vi "MAIN.vi"() -> ()   [LabVIEW 2015]
doc: "Use this template to create an application that executes repeatedly until you click the Stop button. This template polls the state of the Stop button and does not use events. Use the Top-Level Application template (not available in the Base package) to create a single-loop application with event handling."
uses:
  Lib_Bled112 toolkit/type_def/connection_status_bundle.ctl
  Lib_Bled112 toolkit/type_def/address_type.ctl
  Lib_Bled112 toolkit/type_def/message_type.ctl
  Lib_Bled112 toolkit/type_def/message_class.ctl
  <vilib>/Utility/miscctls.llb/LVPointTypeDef.ctl
  SUB_Load and Save Controls.llb/RWC_Actions.ctl
  <vilib>/Utility/miscctls.llb/LVRowAndColumnTypeDef.ctl
  <vilib>/event_ctls.llb/eventvkey.ctl
  <vilib>/Utility/sysdir.llb/System Directory Type.ctl
  <vilib>/addons/_office/_exclsub.llb/font.ctl
  <vilib>/Analysis/baseanly.llb/Mean (DBL).vi
  <vilib>/Utility/config.llb/Read Key (String).vi
  <vilib>/Utility/config.llb/Read Key (I32).vi
  Lib_Bled112 toolkit/ble_functions/ble_write_by_handle_uint8array.vi
  <vilib>/addons/_office/excel.llb/Excel Easy Table (str).vi
  <vilib>/Utility/config.llb/Write Key (String).vi
  <vilib>/Utility/config.llb/Write Key (U32).vi
  <vilib>/Utility/NIReport.llb/NI_report.lvclass
  <vilib>/Utility/config.llb/NI_LVConfig.lvlib
  <vilib>/Analysis/NI_AALBase.lvlib
  <vilib>/addons/_office/NI_ReportGenerationToolkit.lvlib
  <vilib>/Utility/NIReport.llb/Excel/NI_Excel.lvclass
panel:
  out "Packet No.":u16
  out "Rx-debug":bool
  out "FTS table index":i32
  out "ms timer 5":u32=38996702
  out "ms timer 4":u32=27271323
  out "ms timer 3":u32=38996702
  in  "Update(ms)":u16=100
  out "ms timer 2":u32=38996702
  out "Rx-ROM":bool
  out "BLE Packet (mon)":u8[](array[numeric])=[119, 32, 48, 163, 32, 0, 45, 32, 53, 143, 30, 162, 83, 32, 86, 151, 32, 67, 185, 208, 89, 94, 66, 75, 91, 193, 107, 187, 98, 158, 102, 165, 208]
  out "Timer-ble log":u32=38996556
  out "log data1":bool
  out "log ble buf":string
  out "Packet Detect":bool
  out "Disconnected":bool
  out "Rx buf 1":string
  out "Rx Cnt":i32
  out "Rx Packet Structure":T1={"Message Type (Response)"=128, "Payload length"=25, "Command Class (System)"=4, "Message ID"=5, "Connection handle"=0, "Attribute handle"=11, "Attribute type"=1, "Attribute value (data)"=[119, 32, 48, 110, 31, 255, 217, 32, 53, 83, 30, 161, 69, 32, 87, 130, 32, 68, 21, 209]} {"Attribute type" format="%02x" items=["read", "notify", "indicate", "read_by_type", "read_blob", "indicate_rsp_req"]; "Attribute value (data)" format="%02x"; "Attribute handle" format="%04x"; "Connection handle" format="%02x"; "Message ID" format="%02x"; "Message Type (Response)" format="%02x" items=["Command / Response"=0, "Event"=128]; "Command Class (System)" format="%02x" items=["System", "Persistent Store", "Attribute database", "Connection", "Attribute client", "Security Manager", "Generic Access Profile", "Hardware"]}
  out "Device Name":string="GEN4_PERSONA_3rd_jun"
  out "Connection Status":T4={"MAC Address"="F8:B8:54:EF:76:8D", "cnx handle"=0, "cnx flags"=5, "Address Type"=1, "Connection Interval (ms)"=8, "Timeout(ms)"=1000, "Latency"=0, "bonding handle"=255} {"Address Type" items=["Public", "Random"]}
  in  "Log no":string="1" caption="No."
  out "FTS OP status":T6="시험 시작"
  out "Test profile":string[][](array[string])=[["Load(1)-0lb", "0", "1000", "0", "0"], ["Init(1)-70lb", "70", "1000", "0", "0"], ["Init(2)-140lb", "140", "1000", "0", "0"], ["Init(1)-70lb", "70", "1000", "0", "0"], ["Init(2)-140lb", "140", "1000", "0", "0"], ["Load(1)-0lb", "0", "10000", "1", "1"], ["Load(2)-10lb", "10", "3000", "0", "1"], ["Load(3)-20lb", "20", "3000", "0", "1"], ["Load(4)-40lb", "40", "3000", "0", "1"], ["Load(5)-60lb", "60", "3000", "0", "1"], ["Load(6)-80lb", "80", "3000", "0", "1"]]
  out "log refnum":refnum<file> caption="참조 번호 복제"
  out "ms timer":u32=38996556
  out "Logging No.":u32
  in  "Data Logging":bool caption="Data Logging (Desktop folder)"
  out "RxD":string
  out "Graph timer 2":u32=38996702
  out "창크게":bool
  out "Comm err cnt 1":i32
  out "Graph timer 1":u32=38996702
  in  "Setting load":bool=TRUE
  out "ACT-Comm":bool
  in  "Comm con 1":bool
  in  "Port close 1":bool
  in  "Port open 1":bool
  in  "탭-Top":T7(tab)
  in  "CDC Graph plot":bool
  in  "Offset Souce":enum32{"Normal", "Raw"}(radio)
  out "CDC Offet":T8 caption="CDC Offset data" {"Right Wing-C, C6/C0" format="%#.9f"; "Right Wing-B, C5/C0" format="%#.9f"; "Right Wing-A, C4/C0" format="%#.9f"; "Left Wing-C, C3/C0" format="%#.9f"; "Left Wing-B, C2/C0" format="%#.9f"; "Left Wing-A, C1/C0" format="%#.9f"}
  in  "Export graph 1":bool
  in  "Clear graph 1":bool
  out "CDC(PCAP02) Graph":waveform(dbl)[](graph)=[{"t0"=timestamp(3566271640.952271 s since 1904-01-01), "dt"=0.10400000000000001, "Y"=[22878.0]}, {"t0"=timestamp(3566271640.952271 s since 1904-01-01), "dt"=0.10400000000000001, "Y"=[16971.0]}, {"t0"=timestamp(3566271640.952271 s since 1904-01-01), "dt"=0.10400000000000001, "Y"=[23489.0]}, {"t0"=timestamp(3566271640.952271 s since 1904-01-01), "dt"=0.10400000000000001, "Y"=[27579.0]}, {"t0"=timestamp(3566271640.952271 s since 1904-01-01), "dt"=0.10400000000000001, "Y"=[25246.0]}, {"t0"=timestamp(3566271640.952271 s since 1904-01-01), "dt"=0.10400000000000001, "Y"=[26279.0]}, {"t0"=timestamp(3566271640.952271 s since 1904-01-01), "dt"=0.10400000000000001, "Y"=[1.0058650970458984]}, {"t0"=timestamp(3566271640.952271 s since 1904-01-01), "dt"=0.10400000000000001, "Y"=[0.9999599456787109]}, {"t0"=timestamp(3566271640.952271 s since 1904-01-01), "dt"=0.10400000000000001, "Y"=[1.0064787864685059]}, {"t0"=timestamp(3566271640.952271 s since 1904-01-01), "dt"=0.10400000000000001, "Y"=[0.9571785926818848]}, {"t0"=timestamp(3566271640.952271 s since 1904-01-01), "dt"=0.10400000000000001, "Y"=[1.0106620788574219]}, {"t0"=timestamp(3566271640.952271 s since 1904-01-01), "dt"=0.10400000000000001, "Y"=[1.0083107948303223]}]
  out "CDC data":T8 caption="CDC Monitoring data" {"Right Wing-C, C6/C0" format="%#.9f"; "Right Wing-B, C5/C0" format="%#.9f"; "Right Wing-A, C4/C0" format="%#.9f"; "Left Wing-C, C3/C0" format="%#.9f"; "Left Wing-B, C2/C0" format="%#.9f"; "Left Wing-A, C1/C0" format="%#.9f"}
  in  "Offset 1":bool
  out "IMU Offet":T9 caption="IMU Offset data" {"Accelerometer Z" format="%#.9f"; "Accelerometer Y" format="%#.9f"; "Accelerometer X" format="%#.9f"; "Gyroscope Z" format="%#.9f"; "Gyroscope Y" format="%#.9f"; "Gyroscope X" format="%#.9f"}
  out "IMU Graph":waveform(dbl)[](graph)=[{"t0"=timestamp(3566271136.852438 s since 1904-01-01), "dt"=0.108, "Y"=[-1.063125]}, {"t0"=timestamp(3566271136.852438 s since 1904-01-01), "dt"=0.108, "Y"=[0.118125]}, {"t0"=timestamp(3566271136.852438 s since 1904-01-01), "dt"=0.108, "Y"=[0.20125]}, {"t0"=timestamp(3566271136.852438 s since 1904-01-01), "dt"=0.108, "Y"=[-0.014029999999999999]}, {"t0"=timestamp(3566271136.852438 s since 1904-01-01), "dt"=0.108, "Y"=[-0.00366]}, {"t0"=timestamp(3566271136.852438 s since 1904-01-01), "dt"=0.108, "Y"=[1.0149789999999999]}]
  in  "Clear graph 2":bool
  in  "Export graph2":bool
  out "IMU data":T9 caption="IMU Monitoring data" {"Accelerometer Z" format="%#.9f"; "Accelerometer Y" format="%#.9f"; "Accelerometer X" format="%#.9f"; "Gyroscope Z" format="%#.9f"; "Gyroscope Y" format="%#.9f"; "Gyroscope X" format="%#.9f"}
  in  "Offset 2":bool
  out "Full ROM data":bool
  in  "Flash Map":enum32{"Data Map", "Raw Data"}(tab)
  out "ROM Table":string[][](table)=[["Device ID", "-", "-"], ["Main Chip", "-", "-"], ["YEAR", "-", "-"], ["Month", "-", "-"], ["Day", "-", "-"], ["Device Type", "-", "-"], ["Manufacturer ID", "-", "-"], ["Cal_Acc. X", "-", "-"], ["Cal_Acc. Y", "-", "-"], ["Cal_Acc. Z", "-", "-"], ["Cal_Gy. X", "-", "-"], ["Cal_Gy. Y", "-", "-"], ["Cal_Gy. Z", "-", "-"], ["Cal_Vol H", "-", "-"], ["Cal_Vol L", "-", "-"], ["Cal_CDC Off 1", "-", "-"], ["Cal_CDC Off 2", "-", "-"], ["Cal_CDC Off 3", "-", "-"], ["Cal_CDC Off 4", "-", "-"], ["Cal_CDC Off 5", "-", "-"], ["Cal_CDC Off 6", "-", "-"], ["Cal_CDC Gain A", "-", "-"], ["Cal_CDC Gain B", "-", "-"]]
  out "Rx ROM-log":string
  out "ROM Data":T10(array[cluster]) {"Index" format="%02x"; "ROM Data" format="%02x"}
  in  "Mode":bool=TRUE
  in  "Debugging Mode":bool
  in  "Data Log":string
  out "Data_mon(h)":string
  in  "Data(h)":string="\u0001"
  in  "Send":bool
  in  "Handle":u8=16 format="%02x"
  in  "Grahp Clear":bool
  out "BLE RSSI buf":i16(graph)=-63
  out "BLE RSSI Graph":dbl(graph)=-65.56666666666666
  out "BLE RSSI (dBm)":dbl format="%.1f"
  out "BLE AVG-Interval Graph":dbl(graph)=11.355
  out "BLE Interval Time(ms)":dbl format="%.1f"
  out "BLE Interval buf":u32(graph)=11
  out "Bat(raw)":u16 format="%04x"
  in  "Cal/Test select":bool=TRUE
  in  "Head Up":bool
  in  "Load(lb)":dbl=10.0 min=0.0 max=150.0 step=0.1
  in  "Test name":string="Noname"
  out "Load vs CDC Graph":cluster{dbl[], dbl[]}[](graph)
  out "Mark10 Gauge (lb)":dbl format="%.2f"
  out "Test Status":string
  out "Test Data table":string[][](table)=[["-", "-", "-", "-", "-", "-", "-"], ["-", "-", "-", "-", "-", "-", "-"], ["-", "-", "-", "-", "-", "-", "-"], ["-", "-", "-", "-", "-", "-", "-"], ["-", "-", "-", "-", "-", "-", "-"], ["-", "-", "-", "-", "-", "-", "-"], ["-", "-", "-", "-", "-", "-", "-"], ["-", "-", "-", "-", "-", "-", "-"], ["-", "-", "-", "-", "-", "-", "-"]]
  in  "Test Start":bool
  in  "Port-FTS":refnum<visa-resource-name>="COM6" caption="FTS \nCOM port"
  in  "FTS Testing":bool
  out "FTS comm.":bool
  in  "Force Set":bool
  out "Rx-mon":bool
  out "Comm con status 1":bool caption="Status"
  out "*Board ID1":string="None...." caption="S/N"
  in  "Port-set 1":refnum<visa-resource-name>="COM8" caption="COM port"
  out "Port-act 1":refnum<visa-resource-name>="COM8"
  in  "stop":bool=TRUE
  out "Data trx(led)":bool
  in  "Setting load(led)":bool
  out "status string":string="Ready (available after the communication connection)"
  # "GEN4 PP3 - GUI Program"
  # "Ver. 170112A"
  # "Comm. Connection"
  # "(Connection)"
  # "Serial port"
  # "Gyroscope X"
  # "Gyroscope Y"
  # "Gyro. (dps)"
  # "Gyroscope Z"
  # "Accelerometer X"
  # "Accelerometer Y"
  # "Acc. (g)"
  # "Accelerometer Z"
  # "* Debugging mode\nHandler : 0x000B\nWrite : 0x4A 0x73 0x50"
  # "Reserved"
  # "ESM301: 115200bps\nMARK10: 9600bps"
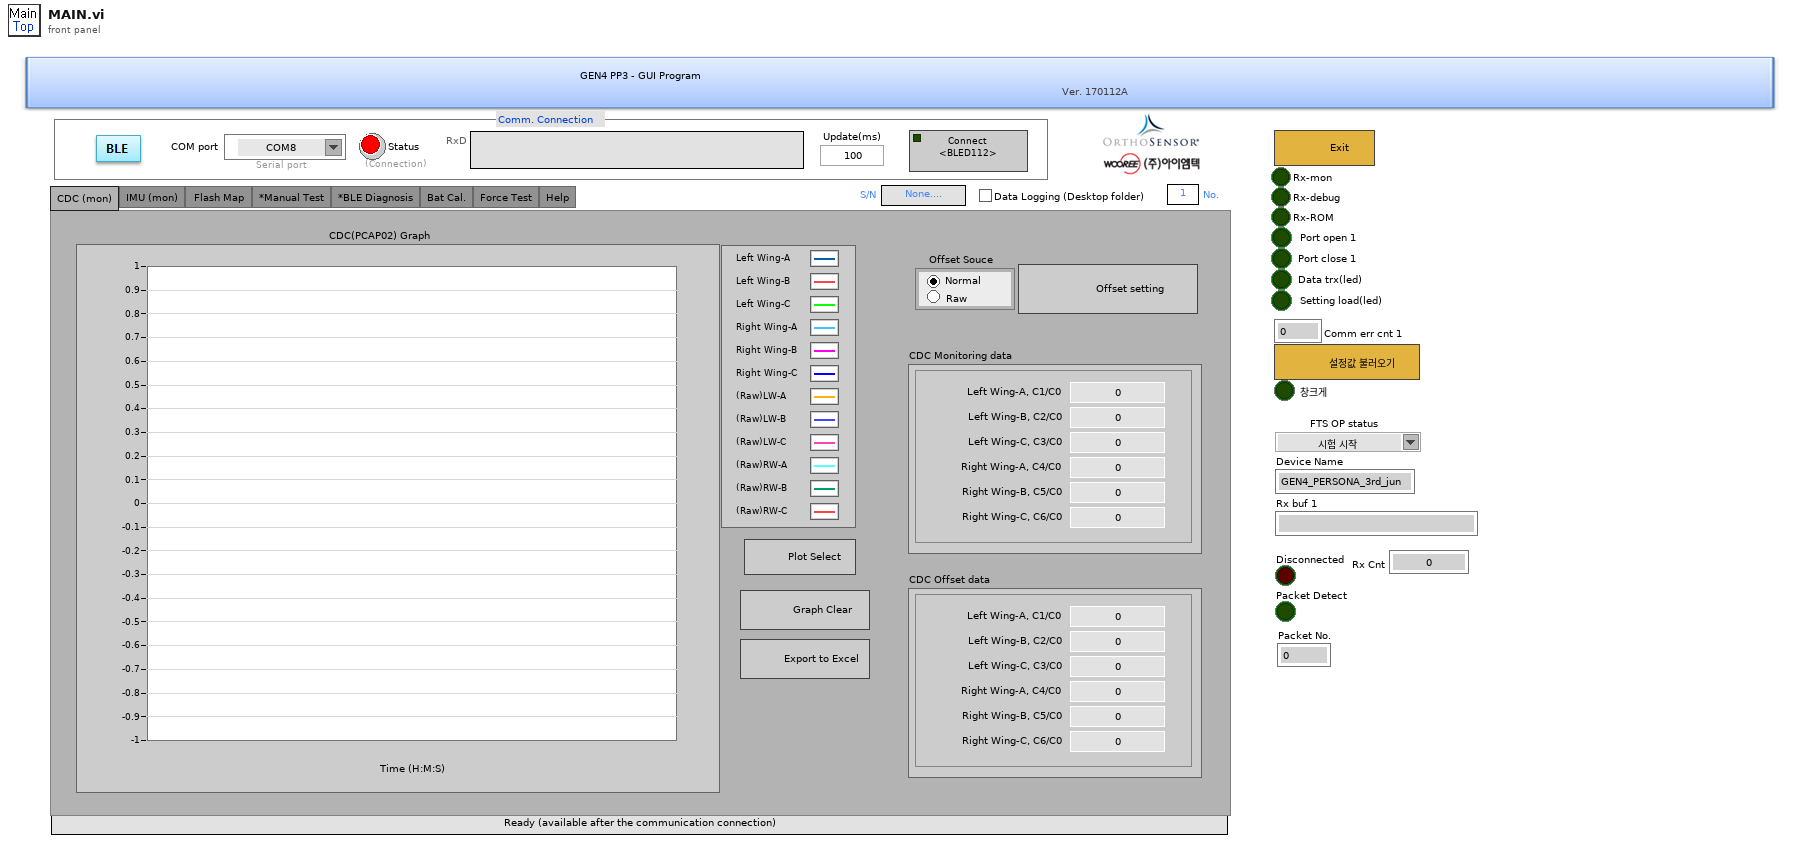
[diagram p1: front panel]
types:
  T1 = typedef "컨트롤-BLED Rx (EVENT-Attribute Client).ctl" = cluster{"Message Type (Response)":T2, "Payload length":u8, "Command Class (System)":T3, "Message ID":u8, "Connection handle":u8, "Attribute handle":u16, "Attribute type":T3, "Attribute value (data)":u8[]}
  T2 = typedef "message_type.ctl" = u8
  T3 = typedef "message_class.ctl" = u8
  T4 = typedef "connection_status_bundle.ctl" = cluster{"MAC Address":string, "cnx handle":u8, "cnx flags":u8, "Address Type":T5, "Connection Interval (ms)":u16, "Timeout(ms)":u16, "Latency":u16, "bonding handle":u8}
  T5 = typedef "address_type.ctl" = u8
  T6 = typedef "컨트롤-동작시험상태 FTS.ctl" = string
  T7 = enum32{"CDC (mon)", "IMU (mon)", "Flash Map ", "*Manual Test", "*BLE Diagnosis", "Bat Cal.", "Force Test", "Help"}
  T8 = typedef "컨트롤-CDC data.ctl" = cluster{"Left Wing-A, C1/C0":dbl, "Left Wing-B, C2/C0":dbl, "Left Wing-C, C3/C0":dbl, "Right Wing-A, C4/C0":dbl, "Right Wing-B, C5/C0":dbl, "Right Wing-C, C6/C0":dbl}
  T9 = typedef "컨트롤-IMU data.ctl" = cluster{"Gyroscope X":dbl, "Gyroscope Y":dbl, "Gyroscope Z":dbl, "Accelerometer X":dbl, "Accelerometer Y":dbl, "Accelerometer Z":dbl}
  T10 = cluster{"RxOK":bool, "ROM Data":u8[], "Index":u8}[]
  T11 = typedef "RWC_Actions.ctl" = enum16{"Read", "Write", "Read and Create"}
  T12 = enum16{"Always On", "Always Off", "Off While Running"}
  T13 = typedef "LVPointTypeDef.ctl" = cluster{"Horizontal":i16, "Vertical":i16}
  T14 = cluster{"RxOK":bool, "ROM Data":u8[], "Index":u8}
  T15 = typedef "LVRowAndColumnTypeDef.ctl" = cluster{"Row":i32, "Column":i32}
  T16 = enum16{"Standard Report", "HTML", "Word", "Excel"}
  T17 = enum16{"maximized", "minimized", "normal", "no change"}
  T18 = typedef "NI_ReportGenerationToolkit.lvlib/font.ctl" = cluster{"font name":string, "font size":dbl, "bold":u16, "italic":u16, "underline":u16, "strike through":u16, "font color":u32}
  T19 = cluster{"on/off":bool, "weight":i32, "color":u32}
  T20 = typedef "컨트롤-동작상태 FTS.ctl" = string
  T21 = typedef "eventvkey.ctl" = enum16{"ASCII", "Enter", "Return", "Shift", "Ctrl", "Alt", "Cmd", "Opt", "Caps", "NumLock", "Clear", "Break", "Up", "Down", "Left", "Right", "Insert", "Delete", "Home", "End", "PageUp", "PageDown", "Escape", "Help", "Pause", "ScrollLock", "F1", "F2", "F3", "F4", "F5", "F6", "F7", "F8", "F9", "F10", "F11", "F12", "F13", "F14", "F15", "F16", "F17", "F18", "F19", "F20", "F21", "F22", "F23", "F24", "Play", "VolumeUp", "VolumeDown", "Mute", "Two Byte Char"}
  T22 = enum16{"open", "replace", "create", "open or create", "replace or create", "replace or create with confirmation"}
  T23 = typedef "NI_LVConfig.lvlib/Config Data RefNum.ctl" = refnum<k1>
  T24 = typedef "System Directory Type.ctl" = i32
  T25 = typedef "LVRectTypeDef.ctl" = cluster{"Left":i16, "Top":i16, "Right":i16, "Bottom":i16}
  T26 = typedef "컨트롤-BLED Rx (EVENT-Connection status).ctl" = cluster{"Message Type (Response)":T2, "Payload length":u8, "Command Class (System)":T3, "Message ID":u8, "Connection handle":u8, "flags":u8, "Bluetooth address":u8[], "address type":T3, "conn_interval(ms)":dbl, "timeout(ms)":dbl, "latency":u16, "bonding(0xFF)":u8}
  T27 = typedef "컨트롤-BLED Rx (Get RSSI).ctl" = cluster{"Message Type (Response)":T2, "Payload length":u8, "Message class":u8, "Message ID":u8, "connection":u8, "rssi":i16}
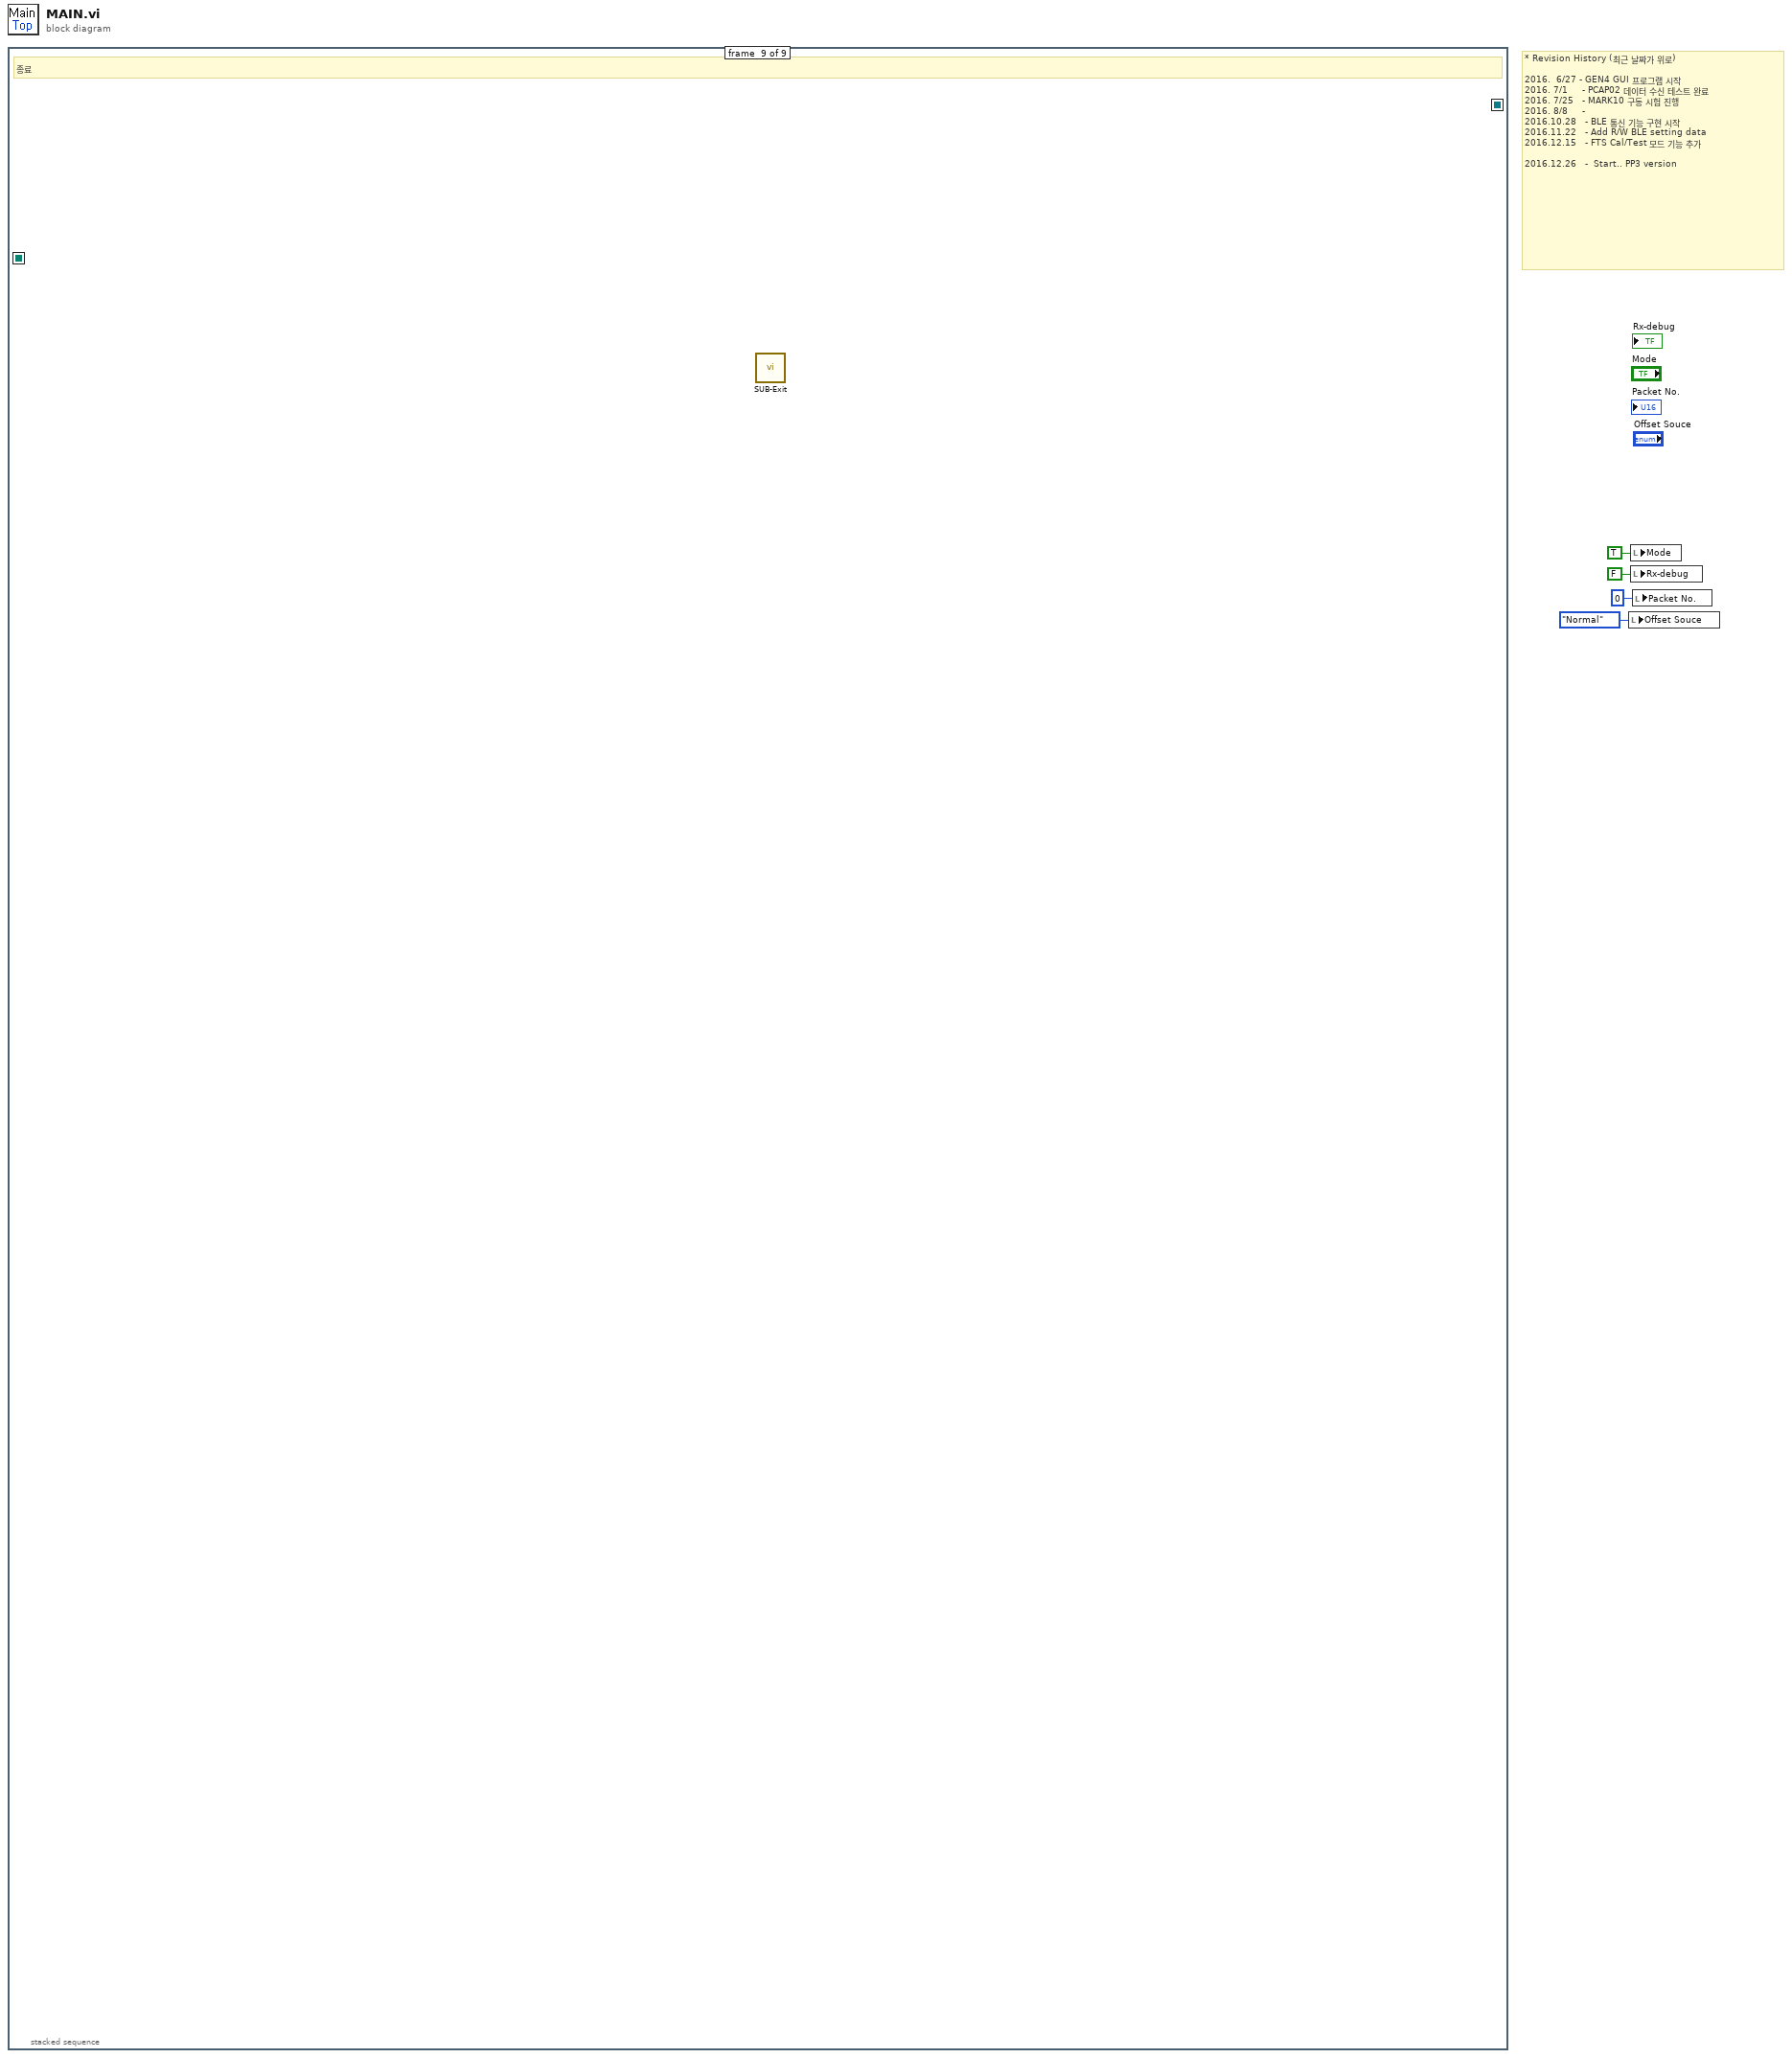
[diagram p0: block diagram]
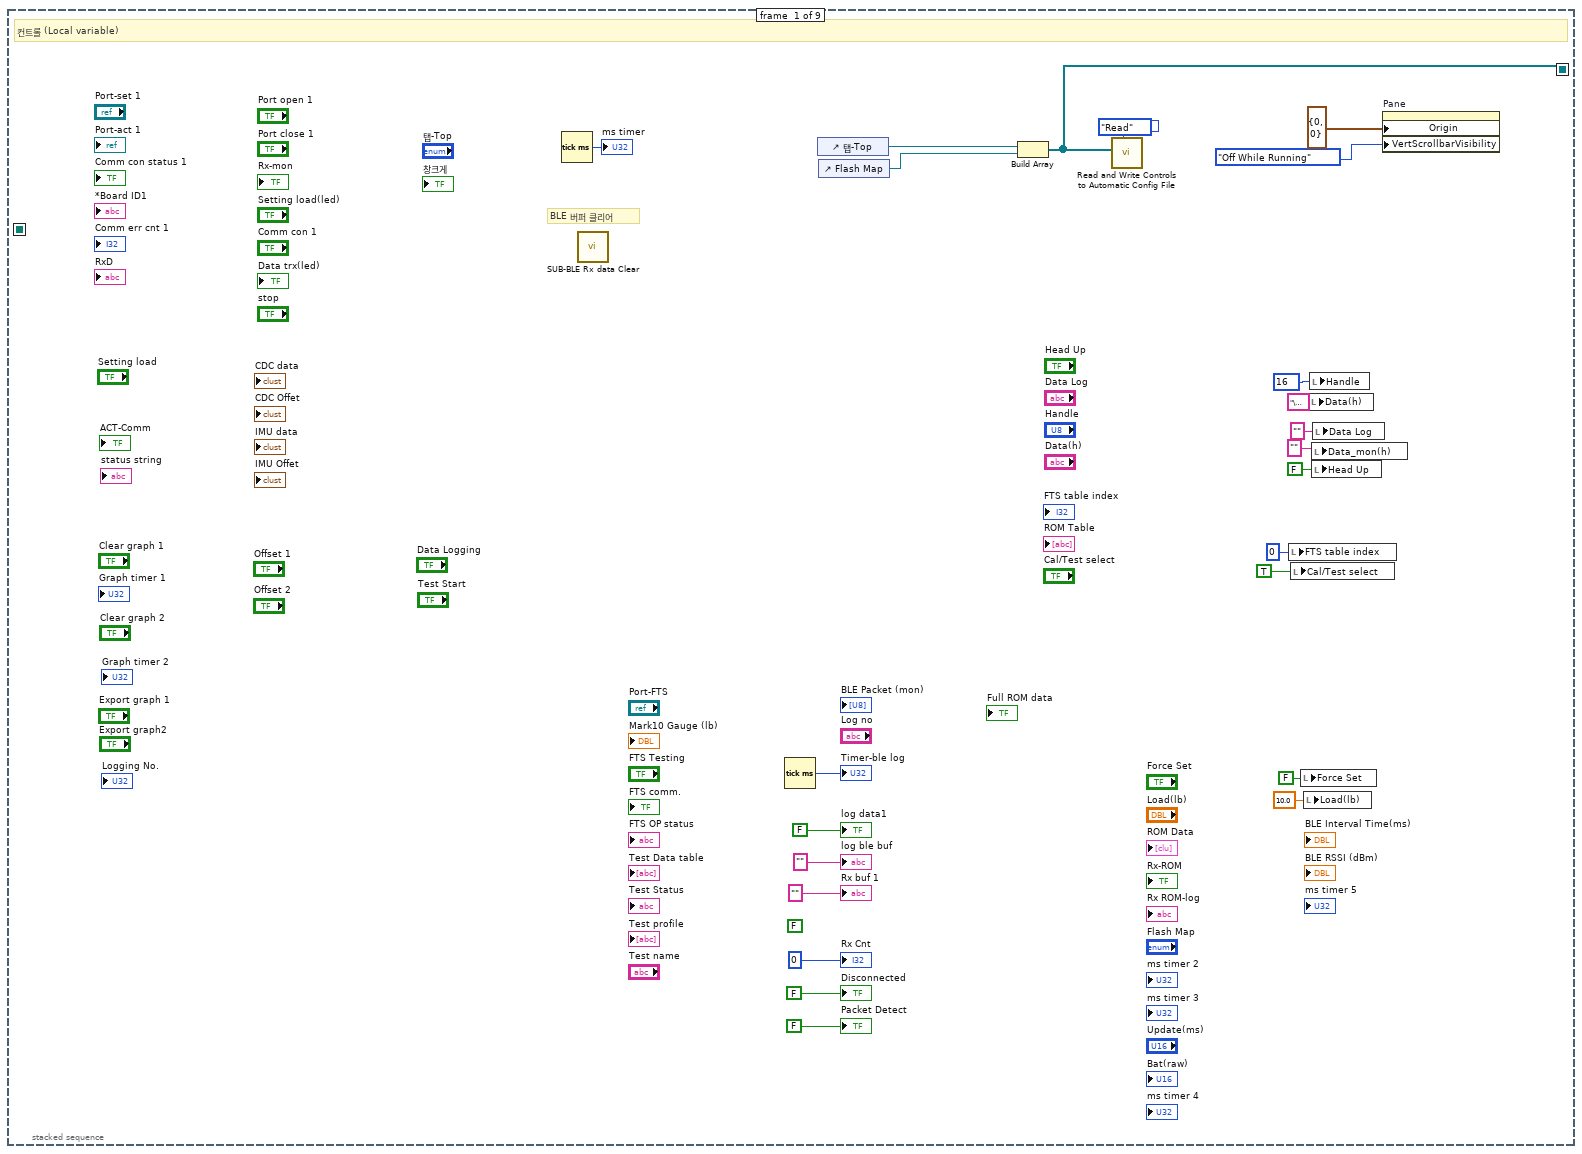
[diagram p2: hidden frame]
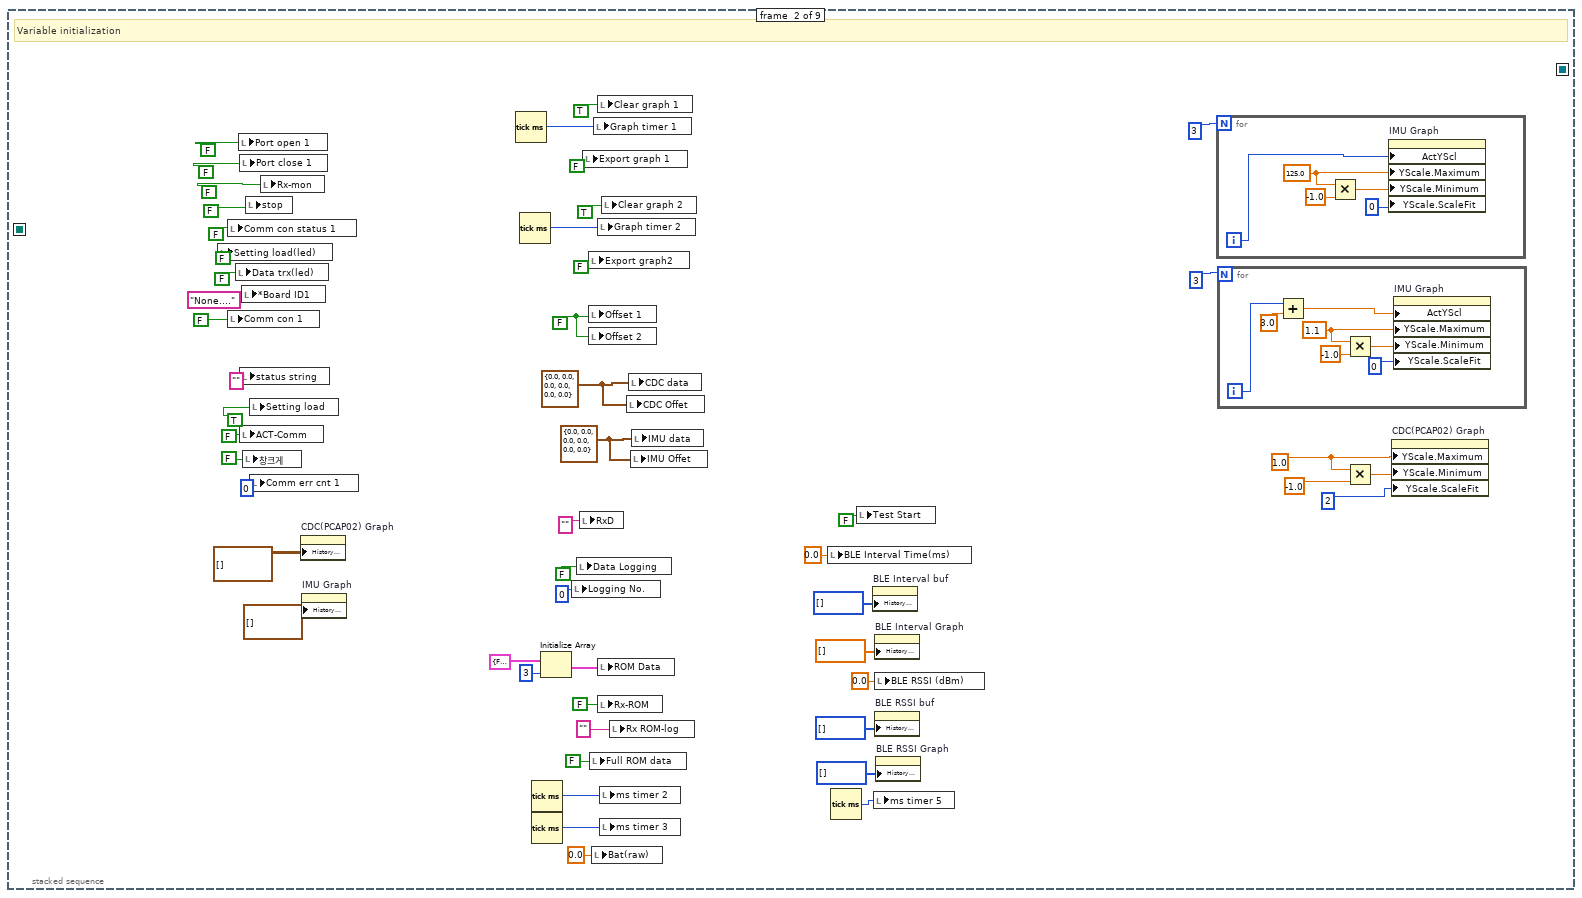
[diagram p3: hidden frame]
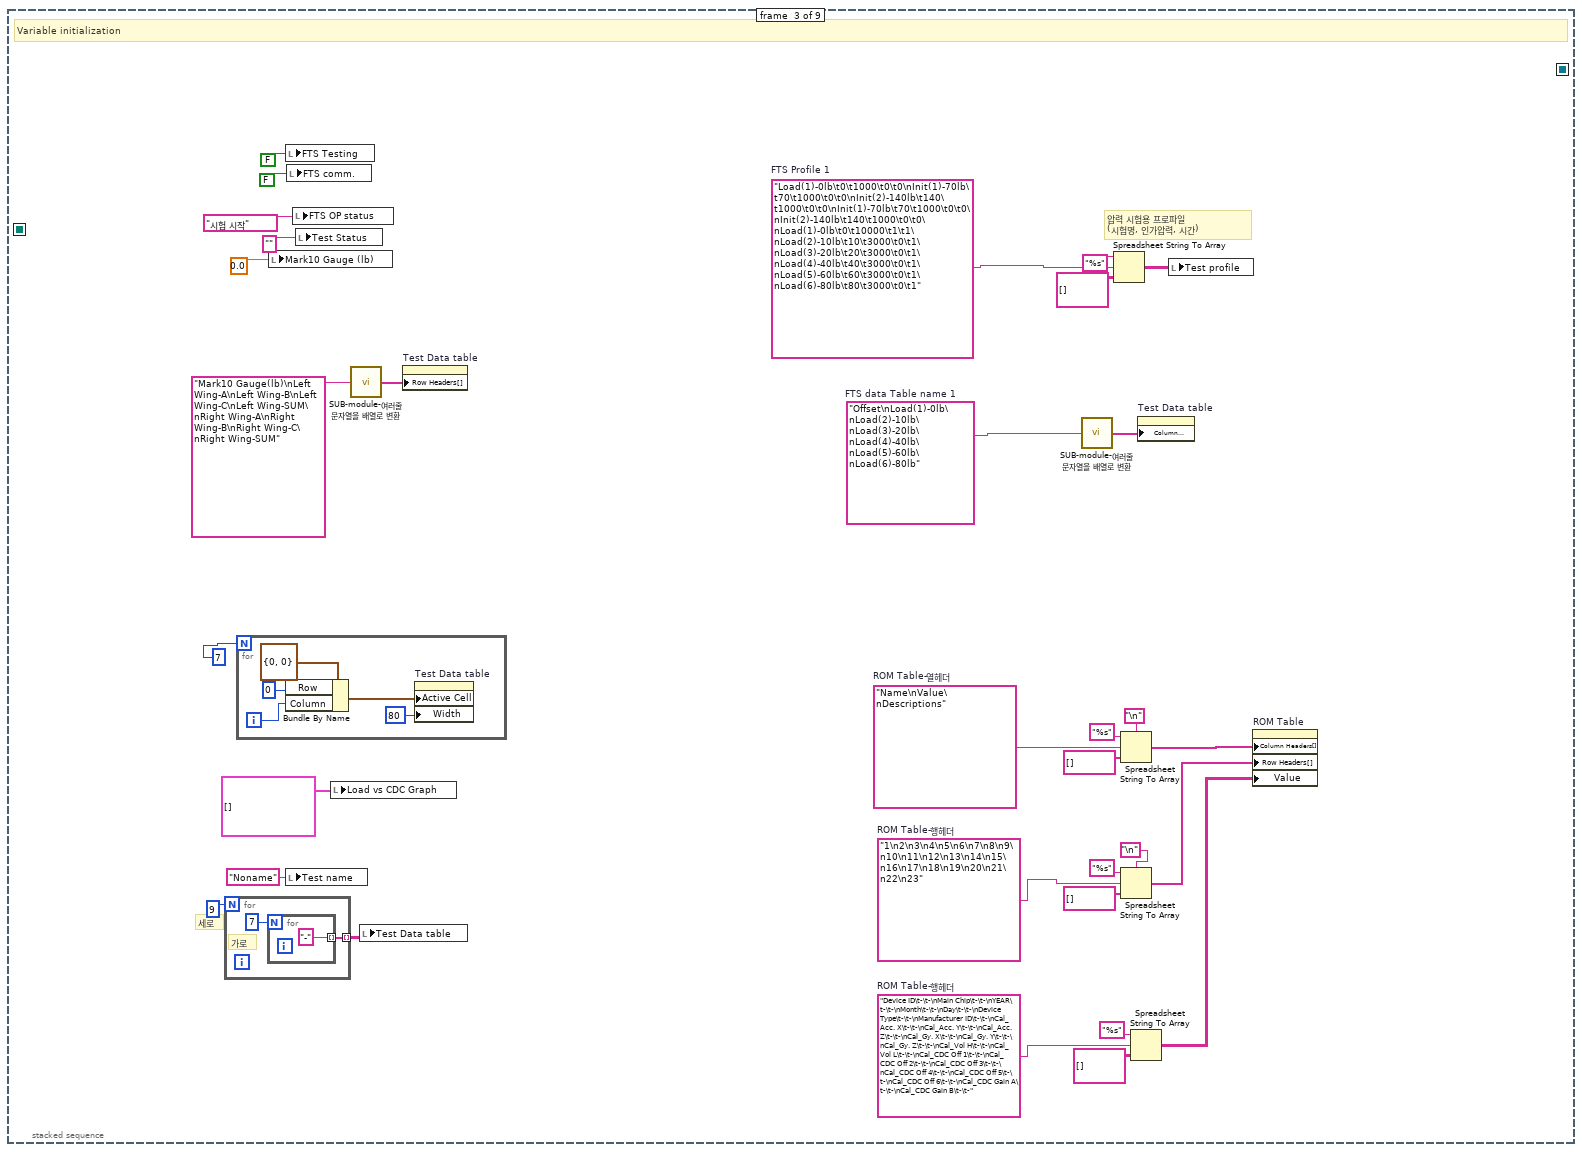
[diagram p4: hidden frame]
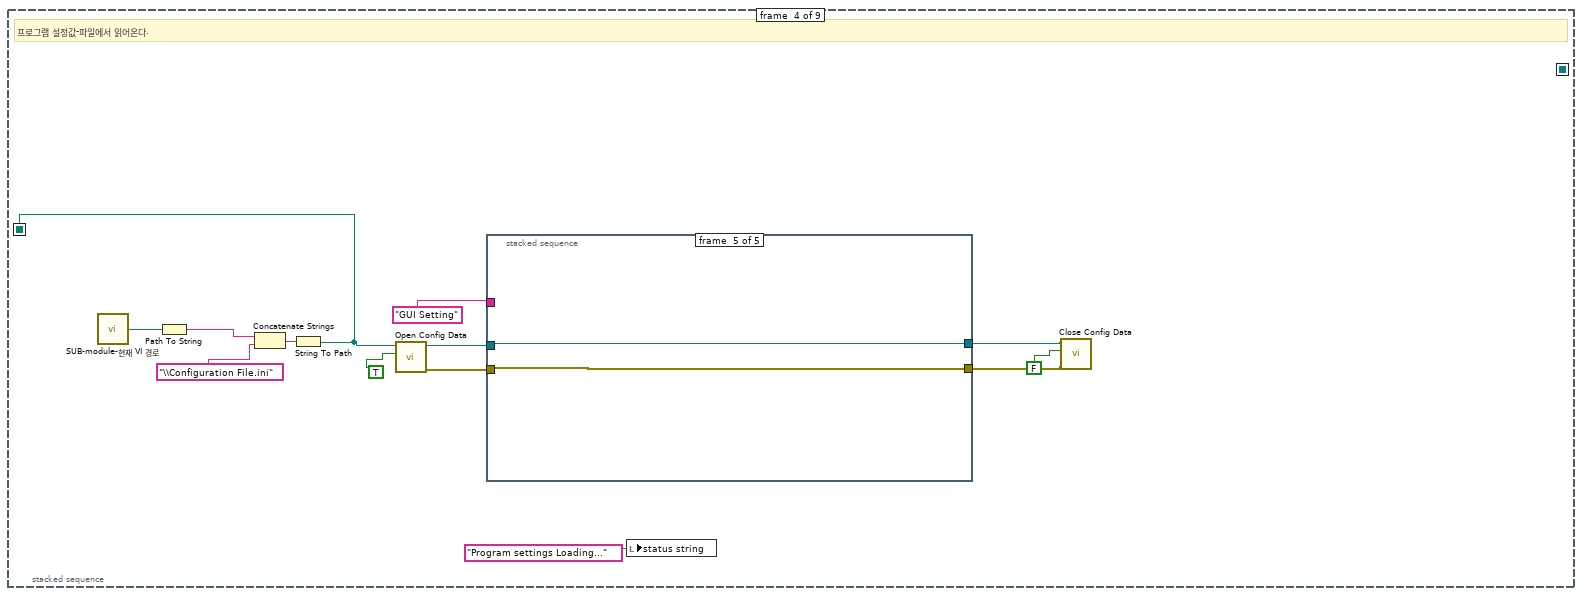
[diagram p5: hidden frame]
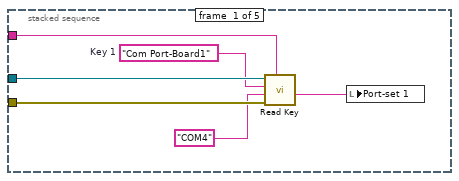
[diagram p6: hidden frame]
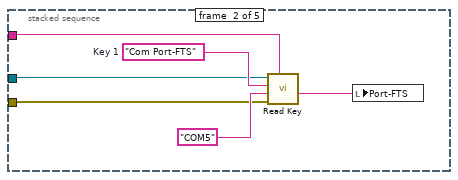
[diagram p7: hidden frame]
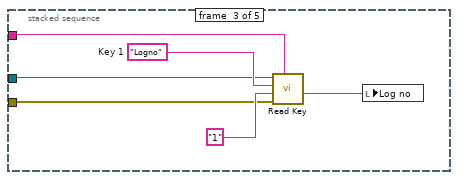
[diagram p8: hidden frame]
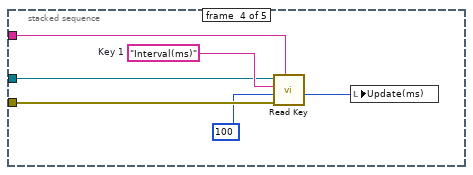
[diagram p9: hidden frame]
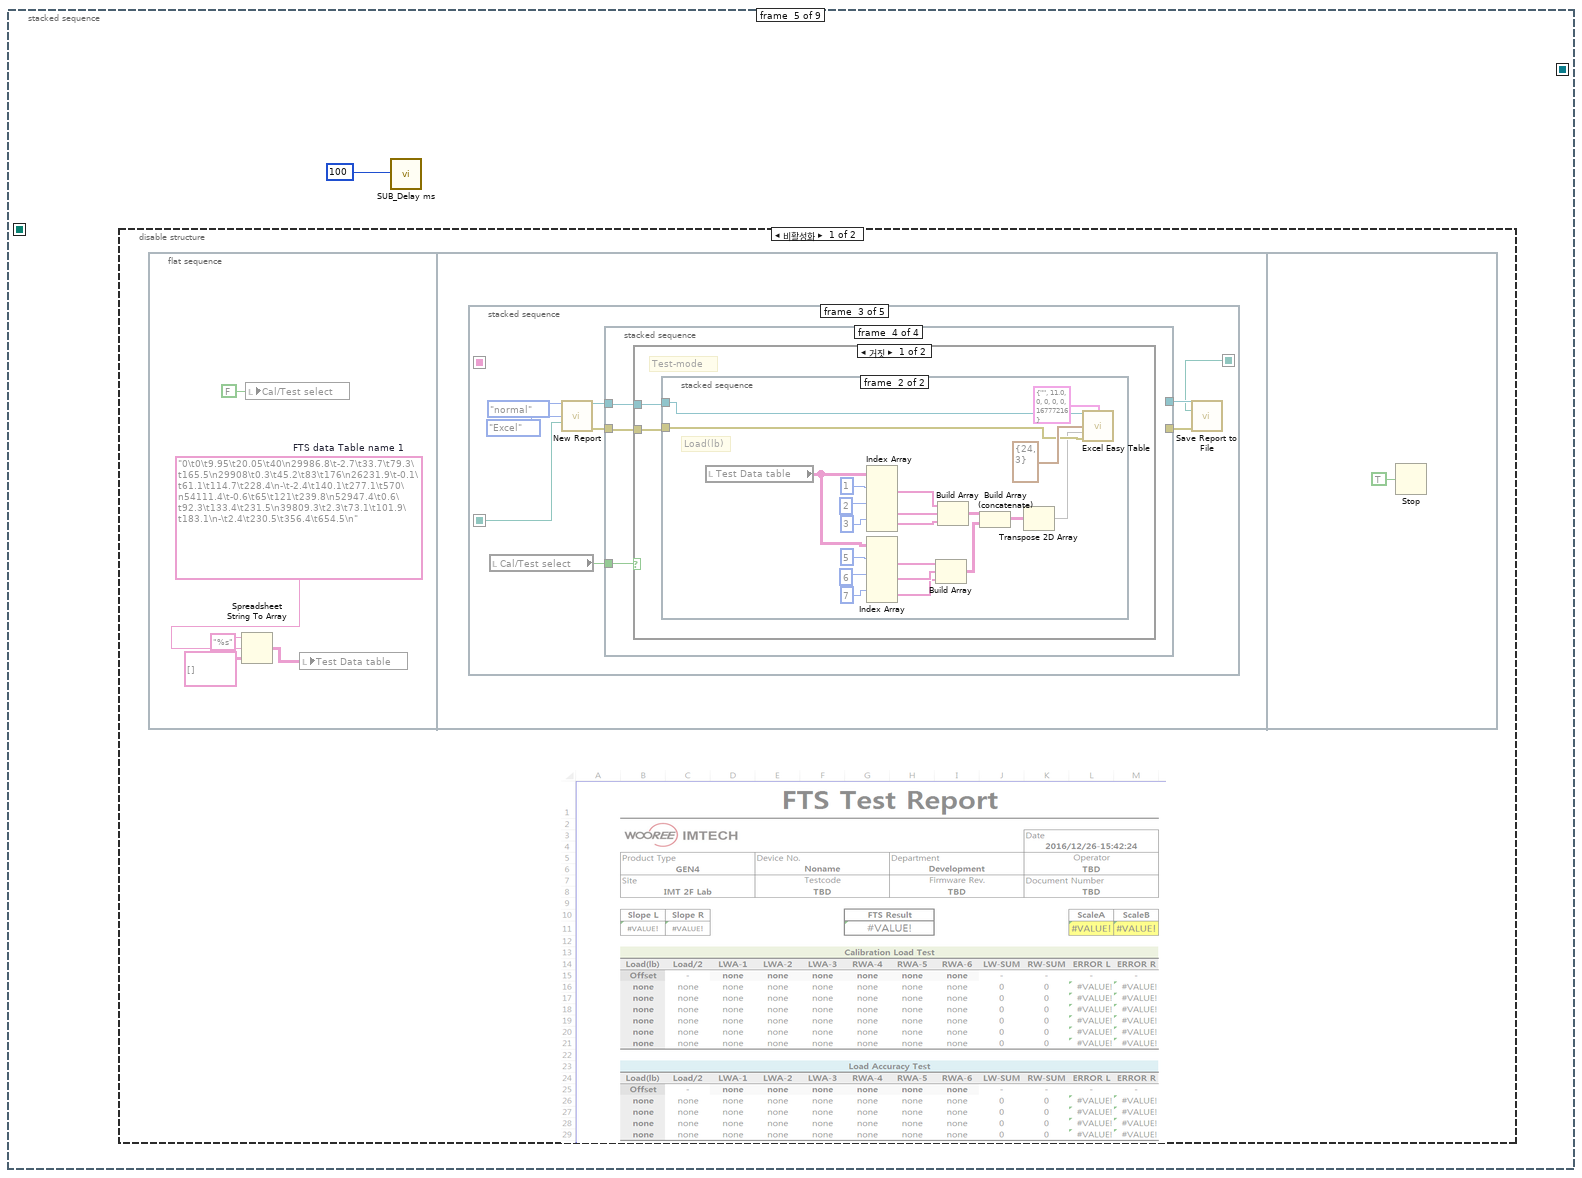
[diagram p10: hidden frame]
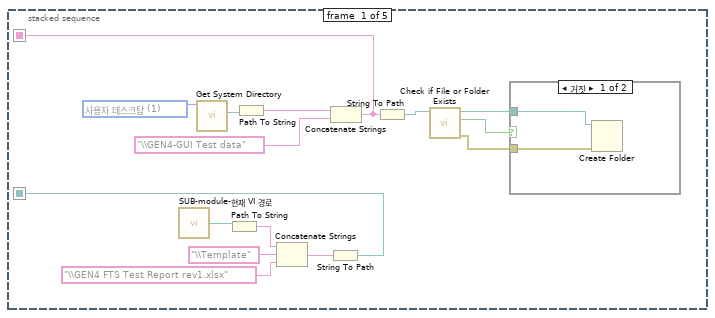
[diagram p11: hidden frame]
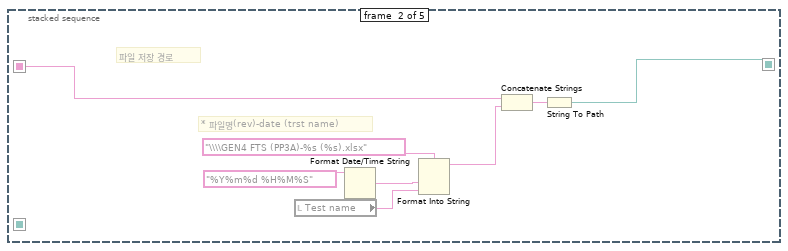
[diagram p13: hidden frame]
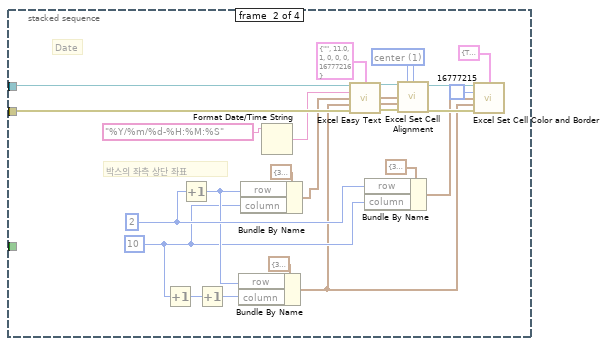
[diagram p15: hidden frame]
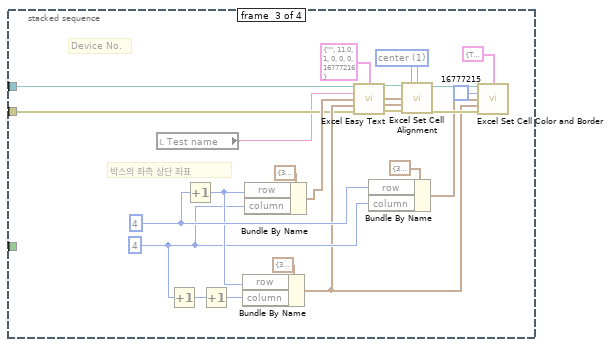
[diagram p16: hidden frame]
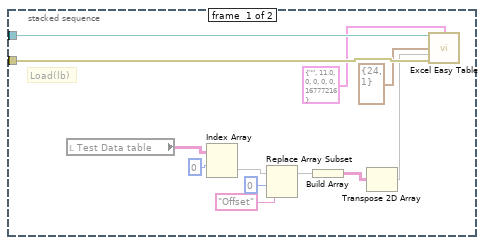
[diagram p17: hidden frame]
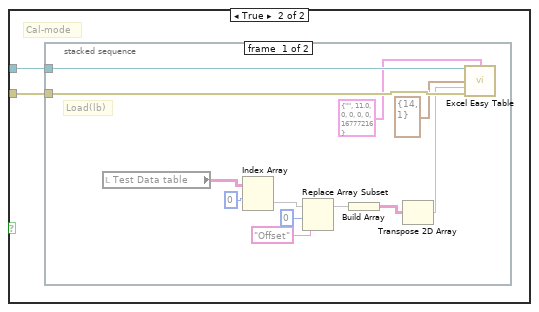
[diagram p18: hidden frame]
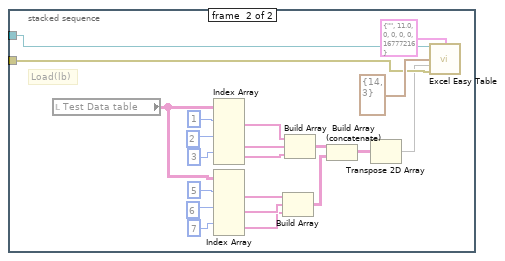
[diagram p19: hidden frame]
diagram:
  # "* Revision History (최근 날짜가 위로)\n\n2016.  6/27 - GEN4 GUI 프로그램 시작\n2016. 7/1     - PCAP02 데이터 수신 테스트 완료\n2016. 7/25   - MARK10 구동 시험 진행\n2016. 8/8     -  \n2016.10.28   - BLE 통신 기능 구현 시작\n2016.11.22   - Add R/W BLE setting data\n2016.12.15   - FTS Cal/Test 모드 기능 추가\n\n2016.12.26   -  Start.. PP3 version"
  n1 = stacked-sequence {
    seq-local: [_ _ _ w135 _ _ _ _ _] -> [_ _ _ _ _ _ _ w1621 _]
    seq-local: [w25 _ _ _ _ _ _ _ _] -> [_ _ _ _ _ _ _ w1617 _]
    frame #0 {
      (unwired) FALSE ("Rx OK")
      # "BLE 버퍼 클리어"
      # "컨트롤 (Local variable)"
      n2 = Tick Count (ms)() -> (millisecond timer value=→"ms timer":u32)
      n3 = call "SUB-BLE Rx data Clear.vi"() -> ()  [unwired: 6 in]
      n4 = Tick Count (ms)() -> (millisecond timer value=→"Timer-ble log":u32)
      n5 = control-ref of="탭-Top"() -> (w23:refnum<vi>)
      n6 = control-ref of="Flash Map"() -> (w7:refnum<vi>)
      n7 = Build Array(w23, w7) -> (w25:refnum<vi>[])
      n8 = call "Read and Write Controls to Automatic Config File.vi"("Action"=RWC_Actions."Read", "Control References"=w25) -> ()  [unwired: 9 in, 1 out]
      n9 = local write "FTS table index"(0 ("FTS table index")) -> ()
      n10 = local write "Cal/Test select"(TRUE ("Cal select")) -> ()
      n11 = local write "Force Set"(FALSE ("Force Set")) -> ()
      n12 = local write "Load(lb)"(10.0 ("Load(lb)")) -> ()
      n13 = local write "Data(h)"("\u0001" ("Data")) -> ()
      n14 = local write "Handle"(u16 16 ("Handle")) -> ()
      n15 = local write "Data_mon(h)"("" ("Data_mon")) -> ()
      n16 = local write "Head Up"(FALSE ("Head Up")) -> ()
      n17 = local write "Data Log"("" ("Data Log")) -> ()
      n18 = property on="Pane" class="Pane"("Origin"=T13 {"Horizontal"=0, "Vertical"=0} ("원점"), "VertScrollbarVisibility"=T12."Off While Running" ("수직 스크롤 막대 보이기")) -> ()  [unwired: 2 in, 2 out]
      "Rx Cnt" <- 0 ("Rx Cnt")
      "Rx buf 1" <- "" ("Rx 문자열 1")
      "Disconnected" <- FALSE ("Disconnected")
      "Packet Detect" <- FALSE ("Packet Detect")
      "log ble buf" <- "" ("log ble buf")
      "log data1" <- FALSE ("log data1")
    }
    frame #1 {
      w49 = 1.0 ("Y 스케일.범위:최대값")
      w55 = T9 {"Gyroscope X"=0.0, "Gyroscope Y"=0.0, "Gyroscope Z"=0.0, "Accelerometer X"=0.0, "Accelerometer Y"=0.0, "Accelerometer Z"=0.0} ("IMU data")
      w56 = T8 {"Left Wing-A, C1/C0"=0.0, "Left Wing-B, C2/C0"=0.0, "Left Wing-C, C3/C0"=0.0, "Right Wing-A, C4/C0"=0.0, "Right Wing-B, C5/C0"=0.0, "Right Wing-C, C6/C0"=0.0} ("CDC data")
      w57 = FALSE ("Offset 1")
      # "Variable initialization"
      n19 = local write "Setting load(led)"(FALSE ("Power On Flag")) -> ()
      n20 = local write "Comm con status 1"(FALSE ("Connected")) -> ()
      n21 = local write "Comm con 1"(FALSE ("포트 연결")) -> ()
      n22 = local write "Data trx(led)"(FALSE ("Rx")) -> ()
      n23 = local write "Port open 1"(FALSE) -> ()
      n24 = local write "Port close 1"(FALSE) -> ()
      n25 = local write "status string"("" ("status string")) -> ()
      n26 = local write "ACT-Comm"(FALSE ("ACT-RS422")) -> ()
      n27 = local write "*Board ID1"("None...." ("*Board ID")) -> ()
      n28 = local write "창크게"(FALSE ("창크게")) -> ()
      n29 = local write "stop"(FALSE ("stop")) -> ()
      n30 = local write "Setting load"(TRUE ("설정값 불러오기")) -> ()
      n31 = local write "Comm err cnt 1"(0 ("통신에러카운트")) -> ()
      n32 = local write "Rx-mon"(FALSE) -> ()
      n33 = property on="CDC(PCAP02) Graph" class="WFChart (엄격한)"("History Data"=waveform(dbl)[][] [] ("히스토리 데이터")) -> ()  [unwired: 2 in, 2 out]
      n34 = property on="IMU Graph" class="WFChart (엄격한)"("History Data"=waveform(dbl)[][] [] ("히스토리 데이터")) -> ()  [unwired: 2 in, 2 out]
      n35 = Tick Count (ms)() -> (millisecond timer value=w66:u32)
      n36 = Tick Count (ms)() -> (millisecond timer value=w59:u32)
      n37 = Tick Count (ms)() -> (millisecond timer value=w41:u32)
      n38 = Tick Count (ms)() -> (millisecond timer value=w42:u32)
      n39 = Initialize Array(T14 {"RxOK"=FALSE, "ROM Data"=[], "Index"=0} ("클러스터"), 3 ("차원 크기")) -> (w37:T10)
      n40 = local write "Logging No."(u32 0 ("Logging No.")) -> ()
      n41 = local write "Data Logging"(FALSE ("Data Logging")) -> ()
      n42 = local write "RxD"("" ("RxD")) -> ()
      n43 = local write "Export graph 1"(FALSE ("그래프 반출")) -> ()
      n44 = local write "Export graph2"(FALSE ("그래프 반출")) -> ()
      n45 = local write "Offset 1"(w57) -> ()
      n46 = local write "Offset 2"(w57) -> ()
      n47 = local write "Full ROM data"(FALSE ("Full ROM data")) -> ()
      n48 = local write "Bat(raw)"(0.0 ("Bat(raw)")) -> ()
      n49 = local write "Graph timer 1"(w66) -> ()
      n50 = local write "Clear graph 1"(TRUE ("그래프 지우기")) -> ()
      n51 = local write "Graph timer 2"(w59) -> ()
      n52 = local write "ROM Data"(w37) -> ()
      n53 = local write "Rx-ROM"(FALSE ("Rx-ROM")) -> ()
      n54 = local write "ms timer 2"(w41) -> ()
      n55 = local write "ms timer 3"(w42) -> ()
      n56 = local write "Clear graph 2"(TRUE ("그래프 지우기")) -> ()
      n57 = local write "Rx ROM-log"("" ("문자열-Rx ROM")) -> ()
      n58 = local write "CDC Offet"(w56) -> ()
      n59 = local write "CDC data"(w56) -> ()
      n60 = local write "IMU Offet"(w55) -> ()
      n61 = local write "IMU data"(w55) -> ()
      n62 = local write "BLE Interval Time(ms)"(0.0 ("BLE Interval Time(ms)")) -> ()
      n63 = Tick Count (ms)() -> (millisecond timer value=w34:u32)
      n64 = local write "Test Start"(FALSE ("Test Start")) -> ()
      n65 = property on="BLE Interval buf" class="WFChart (엄격한)"("History Data"=u32[] [] ("히스토리 데이터")) -> ()  [unwired: 2 in, 2 out]
      n66 = local write "ms timer 5"(w34) -> ()
      n67 = property on="BLE Interval Graph" class="WFChart (엄격한)"("History Data"=dbl[] [] ("히스토리 데이터")) -> ()  [unwired: 2 in, 2 out]
      n68 = local write "BLE RSSI (dBm)"(0.0 ("BLE RSSI (dBm)")) -> ()
      n69 = property on="BLE RSSI buf" class="WFChart (엄격한)"("History Data"=i16[] [] ("히스토리 데이터")) -> ()  [unwired: 2 in, 2 out]
      n70 = property on="BLE RSSI Graph" class="WFChart (엄격한)"("History Data"=i16[] [] ("히스토리 데이터")) -> ()  [unwired: 2 in, 2 out]
      n71 = for {
        N: 3 -> [_]
        i -> [w87]
        w88 = 125.0 ("Y 스케일.범위:최대값")
        n72 = Multiply(x=w88, y=-1.0 ("Y 스케일.범위:최대값")) -> (x*y=w90:dbl)
        n73 = property on="IMU Graph" class="WFChart (엄격한)"("ActYScl"=w87, "YScale.Maximum"=w88, "YScale.Minimum"=w90, "YScale.ScaleFit"=u8 0 ("Y 스케일.스케일 맞춤")) -> ()  [unwired: 2 in, 2 out]
      }
      n74 = for {
        N: 3 -> [_]
        i -> [w82]
        w83 = 1.1 ("Y 스케일.범위:최대값")
        n75 = Add(x=w82, y=3.0 ("Y 스케일.범위:최대값")) -> (x+y=w80:dbl)
        n76 = Multiply(x=w83, y=-1.0 ("Y 스케일.범위:최대값")) -> (x*y=w85:dbl)
        n77 = property on="IMU Graph" class="WFChart (엄격한)"("ActYScl"=w80, "YScale.Maximum"=w83, "YScale.Minimum"=w85, "YScale.ScaleFit"=u8 0 ("Y 스케일.스케일 맞춤")) -> ()  [unwired: 2 in, 2 out]
      }
      n78 = Multiply(x=w49, y=-1.0 ("Y 스케일.범위:최대값")) -> (x*y=w48:dbl)
      n79 = property on="CDC(PCAP02) Graph" class="WFChart (엄격한)"("YScale.Maximum"=w49, "YScale.Minimum"=w48, "YScale.ScaleFit"=u8 2 ("Y 스케일.스케일 맞춤")) -> ()  [unwired: 2 in, 2 out]
    }
    frame #2 {
      w91 = "Device ID\t-\t-\nMain Chip\t-\t-\nYEAR\t-\t-\nMonth\t-\t-\nDay\t-\t-\nDevice Type\t-\t-\nManufacturer ID\t-\t-\nCal_Acc. X\t-\t-\nCal_Acc. Y\t-\t-\nCal_Acc. Z\t-\t-\nCal_Gy. X\t-\t-\nCal_Gy. Y\t-\t-\nCal_Gy. Z\t-\t-\nCal_Vol H\t-\t-\nCal_Vol L\t-\t-\nCal_CDC Off 1\t-\t-\nCal_CDC Off 2\t-\t-\nCal_CDC Off 3\t-\t-\nCal_CDC Off 4\t-\t-\nCal_CDC Off 5\t-\t-\nCal_CDC Off 6\t-\t-\nCal_CDC Gain A\t-\t-\nCal_CDC Gain B\t-\t-"  # ROM Table-행헤더
      w98 = "1\n2\n3\n4\n5\n6\n7\n8\n9\n10\n11\n12\n13\n14\n15\n16\n17\n18\n19\n20\n21\n22\n23"  # ROM Table-행헤더
      w102 = "Name\nValue\nDescriptions"  # ROM Table-열헤더
      w105 = "Load(1)-0lb\t0\t1000\t0\t0\nInit(1)-70lb\t70\t1000\t0\t0\nInit(2)-140lb\t140\t1000\t0\t0\nInit(1)-70lb\t70\t1000\t0\t0\nInit(2)-140lb\t140\t1000\t0\t0\nLoad(1)-0lb\t0\t10000\t1\t1\nLoad(2)-10lb\t10\t3000\t0\t1\nLoad(3)-20lb\t20\t3000\t0\t1\nLoad(4)-40lb\t40\t3000\t0\t1\nLoad(5)-60lb\t60\t3000\t0\t1\nLoad(6)-80lb\t80\t3000\t0\t1"  # FTS Profile 1
      w111 = "Offset\nLoad(1)-0lb\nLoad(2)-10lb\nLoad(3)-20lb\nLoad(4)-40lb\nLoad(5)-60lb\nLoad(6)-80lb"  # FTS data Table name 1
      # "압력 시험용 프로파일\n(시험명, 인가압력, 시간)"
      # "세로"
      # "Variable initialization"
      n80 = for {
        N: 9 -> [_]
        tunnel: [w123] -> w113 mode=indexing
        # "가로"
        n81 = for {
          N: 7 -> [_]
          tunnel: ["-"] -> w123 mode=indexing
        }
      }
      n82 = for {
        N: 7 -> [_]
        i -> [w127]
        n83 = Bundle By Name(cluster=T15 {"Row"=0, "Column"=0} ("활성 셀:활성 셀"), "Row"=0, "Column"=w127) -> (w129:T15)
        n84 = property on="Test Data table" class="Tbl (엄격한)"("Active Cell"=w129, "Width"=u32 80 ("활성 셀:셀 크기:폭")) -> ()  [unwired: 2 in, 2 out]
      }
      n85 = local write "Mark10 Gauge (lb)"(0.0 ("Mark10 Gauge")) -> ()
      n86 = local write "FTS Testing"(FALSE ("FTS 시험 진행")) -> ()
      n87 = local write "Test name"("Noname" ("Test name")) -> ()
      n88 = local write "FTS comm."(FALSE ("FTS 수신 정상")) -> ()
      n89 = local write "FTS OP status"(T6 "시험 시작" ("FTS 동작시험 상태")) -> ()
      n90 = local write "Test Status"("" ("Force Test Status")) -> ()
      n91 = local write "Load vs CDC Graph"(cluster{dbl[], dbl[]}[] [] ("Load vs Ratio Graph")) -> ()
      n92 = call "SUB-module-여러줄 문자열을 배열로 변환.vi"("문자열"="Mark10 Gauge(lb)\nLeft Wing-A\nLeft Wing-B\nLeft Wing-C\nLeft Wing-SUM\nRight Wing-A\nRight Wing-B\nRight Wing-C\nRight Wing-SUM") -> ("배열"=w108:string[])
      n93 = local write "Test Data table"(w113) -> ()
      n94 = property on="Test Data table" class="Tbl (엄격한)"("Row Headers[]"=w108) -> ()  [unwired: 2 in, 2 out]
      n95 = call "SUB-module-여러줄 문자열을 배열로 변환.vi"("문자열"=w111) -> ("배열"=w110:string[])
      n96 = Spreadsheet String To Array(format string="%s" ("포맷 문자열"), spreadsheet string=w105, array type (2D Dbl)=string[][] [] ("배열 타입(2D Dbl)")) -> (array=w117:string[][])  [unwired: 1 in]
      n97 = Spreadsheet String To Array(delimiter (Tab)="\n", format string="%s" ("포맷 문자열"), spreadsheet string=w102, array type (2D Dbl)=string[] [] ("배열 타입(2D Dbl)")) -> (array=w101:string[])
      n98 = Spreadsheet String To Array(delimiter (Tab)="\n", format string="%s" ("포맷 문자열"), spreadsheet string=w98, array type (2D Dbl)=string[] [] ("배열 타입(2D Dbl)")) -> (array=w97:string[])
      n99 = Spreadsheet String To Array(format string="%s" ("포맷 문자열"), spreadsheet string=w91, array type (2D Dbl)=string[][] [] ("배열 타입(2D Dbl)")) -> (array=w92:string[][])  [unwired: 1 in]
      n100 = property on="Test Data table" class="Tbl (엄격한)"("Column Headers[]"=w110) -> ()  [unwired: 2 in, 2 out]
      n101 = local write "Test profile"(w117) -> ()
      n102 = property on="ROM Table" class="Tbl (엄격한)"("Column Headers[]"=w101, "Row Headers[]"=w97, "Value"=w92) -> ()  [unwired: 2 in, 2 out]
    }
    frame #3 {
      # "프로그램 설정값-파일에서 읽어온다."
      n103 = call "SUB-module-현재 VI 경로.vi"() -> ("현재 VI 경로"=w136:path)
      n104 = Path To String(path=w136) -> (string=w138:string)
      n105 = Concatenate Strings(w138, "\\Configuration File.ini") -> (w137:string)
      n106 = String To Path(string=w137) -> (path=w135:path)
      n107 = call <vilib>:"Open Config Data.vi"("create file if necessary (T)"=TRUE, "configuration file path"=w135) -> ("error out"=w142:errorcluster, "refnum"=w141:T23)  [unwired: 7 in, 1 out]
      n108 = stacked-sequence {
        tunnel: w141 -> [w149 w151 w157 w164 w169]
        tunnel: w142 -> [w148 w150 w156 w163 w168]
        tunnel: "GUI Setting" ("section") -> [w147 w152 w158 w165 _]
        tunnel: [_ _ _ _ w169] -> w133
        tunnel: [_ _ _ _ w168] -> w132
        frame #0 {
          w146 = "Com Port-Board1"  # Key 1
          n109 = call-poly <vilib>:"Read Key.vi"("section"=w147, "error in (no error)"=w148, "default value"="COM4" ("output string"), "key"=w146, "refnum"=w149) -> ("value"=w145:string)  [unwired: 3 in, 3 out]
          n110 = local write "Port-set 1"(w145) -> ()
        }
        frame #1 {
          w155 = "Com Port-FTS"  # Key 1
          n111 = call-poly <vilib>:"Read Key.vi"("section"=w152, "error in (no error)"=w150, "default value"="COM5" ("output string"), "key"=w155, "refnum"=w151) -> ("value"=w154:string)  [unwired: 3 in, 3 out]
          n112 = local write "Port-FTS"(w154) -> ()
        }
        frame #2 {
          w161 = "Logno"  # Key 1
          n113 = call-poly <vilib>:"Read Key.vi"("section"=w158, "error in (no error)"=w156, "default value"="1" ("output string"), "key"=w161, "refnum"=w157) -> ("value"=w160:string)  [unwired: 3 in, 3 out]
          n114 = local write "Log no"(w160) -> ()
        }
        frame #3 {
          w167 = "Interval(ms)"  # Key 1
          n115 = call-poly <vilib>:"Read Key.vi"("section"=w165, "error in (no error)"=w163, "default value"=100, "key"=w167, "refnum"=w164) -> ("value"=w166:i32)  [unwired: 3 in, 3 out]
          n116 = local write "Update(ms)"(w166) -> ()
        }
        frame #4 {
        }
      }
      n117 = local write "status string"("Program settings Loading..." ("status string")) -> ()
      n118 = call <vilib>:"Close Config Data.vi"("error in (no error)"=w132, "write file if changed (T)"=FALSE ("write configuration file? (T)"), "refnum"=w133) -> ()  [unwired: 9 out]
    }
    frame #4 {
      n119 = disable-structure shown="비활성화" {
        frame Disabled {
          n120 = flat-sequence {
            frame #0 {
              w173 = "0\t0\t9.95\t20.05\t40\n29986.8\t-2.7\t33.7\t79.3\t165.5\n29908\t0.3\t45.2\t83\t176\n26231.9\t-0.1\t61.1\t114.7\t228.4\n-\t-2.4\t140.1\t277.1\t570\n54111.4\t-0.6\t65\t121\t239.8\n52947.4\t0.6\t92.3\t133.4\t231.5\n39809.3\t2.3\t73.1\t101.9\t183.1\n-\t2.4\t230.5\t356.4\t654.5\n"  # FTS data Table name 1
              n121 = Spreadsheet String To Array(format string="%s" ("포맷 문자열"), spreadsheet string=w173, array type (2D Dbl)=string[][] [] ("배열 타입(2D Dbl)")) -> (array=w172:string[][])  [unwired: 1 in]
              n122 = local write "Cal/Test select"(FALSE ("Cal/Test select")) -> ()
              n123 = local write "Test Data table"(w172) -> ()
            }
            frame #1 {
              n124 = stacked-sequence {
                seq-local: [_ w194 _ _ _] -> [_ _ w203 _ _]
                seq-local: [w182 _ _ _ _] -> [_ w193 _ _ _]
                seq-local: [w176 _ _ _ _] -> [_ _ w202 _ _]
                frame #0 {
                  w190 = T24 1 items=["사용자 홈"=0, "사용자 데스크탑"=1, "사용자 문서"=2, "사용자 어플리케이션 데이터"=3, "사용자 환경"=4, "사용자 임시"=5, "퍼블릭 문서"=6, "퍼블릭 어플리케이션 데이터"=7, "퍼블릭 환경"=8, "퍼블릭 캐시"=13, "시스템 코어 라이브러리"=9, "시스템 설치된 라이브러리"=10, "어플리케이션 파일"=11, "부팅 볼륨 루트"=12] ("system directory type")
                  n125 = call "SUB-module-현재 VI 경로.vi"() -> ("현재 VI 경로"=w179:path)
                  n126 = call <vilib>:"Get System Directory.vi"("system directory type"=w190) -> ("system directory"=w189:path)  [unwired: 10 in]
                  n127 = Path To String(path=w179) -> (string=w178:string)
                  n128 = Path To String(path=w189) -> (string=w188:string)
                  n129 = Concatenate Strings(w178, "\\Template" ("이름 또는 상대 경로"), "\\GEN4 FTS Test Report rev1.xlsx" ("이름 또는 상대 경로")) -> (w177:string)
                  n130 = String To Path(string=w177) -> (path=w176:path)
                  n131 = Concatenate Strings(w188, "\\GEN4-GUI Test data" ("상태")) -> (w182:string)
                  n132 = String To Path(string=w182) -> (path=w186:path)
                  n133 = call <vilib>:"Check if File or Folder Exists.vi"("path"=w186) -> ("error out"=w183:errorcluster, "file or folder exists?"=w185:bool, "dup path"=w184:path)  [unwired: 8 in]
                  n134 = case shown="거짓" w185 {
                    tunnel: w184 -> [w192 _]
                    tunnel: w183 -> [w191 _]
                    frame False {
                      n135 = Create Folder(path (use dialog)=w192, error in=w191) -> ()  [unwired: 1 in, 3 out]
                    }
                    frame True {
                    }
                  }
                }
                frame #1 {
                  # "* 파일명(rev)-date (trst name)"
                  # "파일 저장 경로"
                  n136 = local read "Test name"() -> (w199:string)
                  n137 = Format Date/Time String(time format string (%c)="%Y%m%d %H%M%S" ("상태")) -> (date/time string=w198:string)  [unwired: 2 in]
                  n138 = Format Into String(format string="\\\\GEN4 FTS (PP3A)-%s (%s).xlsx" ("상태"), w198, w199) -> (resulting string=w195:string)  [unwired: 2 in, 1 out]
                  n139 = Concatenate Strings(w193, w195) -> (w200:string)
                  n140 = String To Path(string=w200) -> (path=w194:path)
                }
                frame #2 {
                  n141 = local read "Cal/Test select"() -> (w201:bool)
                  n142 = call <vilib>:"New Report.vi"("window state (normal)"=T17."normal", "report type"=T16."Excel", "template (empty)"=w202) -> ("report out"=w206:refnum<class "NI_report.lvclass">, "error out"=w207:errorcluster)  [unwired: 11 in]
                  n143 = stacked-sequence {
                    tunnel: w206 -> [w211 w236 w238 w263]
                    tunnel: w207 -> [w210 w235 w239 w262]
                    tunnel: [w211 _ _ _] -> w209
                    tunnel: [w210 _ _ _] -> w208
                    tunnel: w201 -> [_ _ _ w261]
                    frame #0 {
                    }
                    frame #1 {
                      w214 = 10 ("column")
                      w221 = 2 ("row")
                      w228 = 1 items=["top", "center", "bottom"] ("vertical alignment (top)")
                      # "Date"
                      # "박스의 좌측 상단 좌표"
                      n144 = Increment(x=w214) -> (x+1=w213:i32)
                      n145 = Increment(x=w221) -> (x+1=w216:i32)
                      n146 = Increment(x=w213) -> (x+1=w215:i32)
                      n147 = Bundle By Name(cluster=cluster{"row":i32, "column":i32} {"row"=3, "column"=10} ("start (-1, -1)"), "row"=w216, "column"=w215) -> (w212:cluster{"row":i32, "column":i32})
                      n148 = Bundle By Name(cluster=cluster{"row":i32, "column":i32} {"row"=3, "column"=10} ("start (-1, -1)"), "row"=w216, "column"=w214) -> (w222:cluster{"row":i32, "column":i32})
                      n149 = Format Date/Time String(time format string (%c)="%Y/%m/%d-%H:%M:%S" ("상태")) -> (date/time string=w234:string)  [unwired: 2 in]
                      n150 = call <vilib>:"Excel Easy Text.vi"("report in"=w236, "font"=T18 {"font name"="", "font size"=11.0, "bold"=1, "italic"=0, "underline"=0, "strike through"=0, "font color"=16777216}, "text"=w234, "start (-1, -1)"=w222, "end (-1, -1)"=w212, "error in (no error)"=w235) -> ("report out"=w232:refnum<class "NI_report.lvclass">, "next cell bottom-left"=w230:cluster{"row":i32, "column":i32}, "next cell top-right"=w229:cluster{"row":i32, "column":i32}, "error out"=w231:errorcluster)  [unwired: 5 in, 1 out]
                      n151 = Bundle By Name(cluster=cluster{"row":i32, "column":i32} {"row"=3, "column"=10} ("start (-1, -1)"), "row"=w221, "column"=w214) -> (w220:cluster{"row":i32, "column":i32})
                      n152 = call <vilib>:"Excel Set Cell Alignment.vi"("report in"=w232, "vertical alignment (top)"=w228, "horizontal alignment (left)"=w228, "start (-1, -1)"=w230, "end (-1, -1)"=w229, "error in (no error)"=w231) -> ("report out"=w227:refnum<class "NI_report.lvclass">, "error out"=w226:errorcluster)  [unwired: 8 in]
                      n153 = call <vilib>:"Excel Set Cell Color and Border.vi"("report in"=w227, "outside border"=T19 {"on/off"=TRUE, "weight"=2, "color"=0}, "background color (w)"=u32 16777215, "start (-1, -1)"=w220, "end (-1, -1)"=w212, "error in (no error)"=w226) -> ()  [unwired: 8 in, 2 out]
                    }
                    frame #2 {
                      w242 = 4 ("column")
                      w249 = 4 ("row")
                      w256 = 1 items=["top", "center", "bottom"] ("vertical alignment (top)")
                      # "Device No."
                      # "박스의 좌측 상단 좌표"
                      n154 = local read "Test name"() -> (w237:string)
                      n155 = Increment(x=w242) -> (x+1=w241:i32)
                      n156 = Increment(x=w249) -> (x+1=w244:i32)
                      n157 = Increment(x=w241) -> (x+1=w243:i32)
                      n158 = Bundle By Name(cluster=cluster{"row":i32, "column":i32} {"row"=3, "column"=10} ("start (-1, -1)"), "row"=w244, "column"=w243) -> (w240:cluster{"row":i32, "column":i32})
                      n159 = Bundle By Name(cluster=cluster{"row":i32, "column":i32} {"row"=3, "column"=10} ("start (-1, -1)"), "row"=w244, "column"=w242) -> (w250:cluster{"row":i32, "column":i32})
                      n160 = call <vilib>:"Excel Easy Text.vi"("report in"=w238, "font"=T18 {"font name"="", "font size"=11.0, "bold"=1, "italic"=0, "underline"=0, "strike through"=0, "font color"=16777216}, "text"=w237, "start (-1, -1)"=w250, "end (-1, -1)"=w240, "error in (no error)"=w239) -> ("report out"=w260:refnum<class "NI_report.lvclass">, "next cell bottom-left"=w258:cluster{"row":i32, "column":i32}, "next cell top-right"=w257:cluster{"row":i32, "column":i32}, "error out"=w259:errorcluster)  [unwired: 5 in, 1 out]
                      n161 = Bundle By Name(cluster=cluster{"row":i32, "column":i32} {"row"=3, "column"=10} ("start (-1, -1)"), "row"=w249, "column"=w242) -> (w248:cluster{"row":i32, "column":i32})
                      n162 = call <vilib>:"Excel Set Cell Alignment.vi"("report in"=w260, "vertical alignment (top)"=w256, "horizontal alignment (left)"=w256, "start (-1, -1)"=w258, "end (-1, -1)"=w257, "error in (no error)"=w259) -> ("report out"=w255:refnum<class "NI_report.lvclass">, "error out"=w254:errorcluster)  [unwired: 8 in]
                      n163 = call <vilib>:"Excel Set Cell Color and Border.vi"("report in"=w255, "outside border"=T19 {"on/off"=TRUE, "weight"=2, "color"=0}, "background color (w)"=u32 16777215, "start (-1, -1)"=w248, "end (-1, -1)"=w240, "error in (no error)"=w254) -> ()  [unwired: 8 in, 2 out]
                    }
                    frame #3 {
                      n164 = case shown="거짓" w261 {
                        tunnel: w263 -> [w265 w300]
                        tunnel: w262 -> [w264 w299]
                        frame False {
                          # "Test-mode"
                          n165 = stacked-sequence {
                            tunnel: w265 -> [w277 w296]
                            tunnel: w264 -> [w276 w295]
                            frame #0 {
                              # "Load(lb)"
                              n166 = local read "Test Data table"() -> (w275:string[][])
                              n167 = Index Array(array=w275, index (row)=0 ("인덱스 (행)")) -> (element=w272:string[])  [unwired: 1 in]
                              n168 = Replace Array Subset(array=w272, new element="Offset" ("새 원소/부분배열"), index=0 ("인덱스")) -> (w269:string[])
                              n169 = Build Array(w269) -> (w268:string[][])
                              n170 = Transpose 2D Array(2D array=w268) -> (transposed array=w267:string[][])
                              n171 = call-poly <vilib>:"Excel Easy Table.vi"("report in"=w277, "font"=T18 {"font name"="", "font size"=11.0, "bold"=0, "italic"=0, "underline"=0, "strike through"=0, "font color"=16777216}, "start (0, 0)"=cluster{"row":i32, "column":i32} {"row"=24, "column"=1}, "text data"=w267, "error in (no error)"=w276) -> ()  [unwired: 6 in, 5 out]
                            }
                            frame #1 {
                              # "Load(lb)"
                              n172 = local read "Test Data table"() -> (w289:string[][])
                              n173 = Index Array(array=w289, index (row) #1=1 ("인덱스 (행)"), index (row) #2=2 ("인덱스 (행)"), index (row) #3=3 ("인덱스 (행)")) -> (element #1=w288:string[], element #2=w287:string[], element #3=w286:string[])  [unwired: 3 in]
                              n174 = Index Array(array=w289, index (row) #1=5 ("인덱스 (행)"), index (row) #2=6 ("인덱스 (행)"), index (row) #3=7 ("인덱스 (행)")) -> (element #1=w285:string[], element #2=w284:string[], element #3=w283:string[])  [unwired: 3 in]
                              n175 = Build Array(w285, w284, w283) -> (w281:string[][])
                              n176 = Build Array(w288, w287, w286) -> (w282:string[][])
                              n177 = Build Array (concatenate)(w282, w281) -> (w280:string[][])
                              n178 = Transpose 2D Array(2D array=w280) -> (transposed array=w279:string[][])
                              n179 = call-poly <vilib>:"Excel Easy Table.vi"("report in"=w296, "font"=T18 {"font name"="", "font size"=11.0, "bold"=0, "italic"=0, "underline"=0, "strike through"=0, "font color"=16777216}, "start (0, 0)"=cluster{"row":i32, "column":i32} {"row"=24, "column"=3}, "text data"=w279, "error in (no error)"=w295) -> ()  [unwired: 6 in, 5 out]
                            }
                          }
                        }
                        frame True {
                          # "Cal-mode"
                          n180 = stacked-sequence {
                            tunnel: w300 -> [w312 w331]
                            tunnel: w299 -> [w311 w330]
                            frame #0 {
                              # "Load(lb)"
                              n181 = local read "Test Data table"() -> (w310:string[][])
                              n182 = Index Array(array=w310, index (row)=0 ("인덱스 (행)")) -> (element=w307:string[])  [unwired: 1 in]
                              n183 = Replace Array Subset(array=w307, new element="Offset" ("새 원소/부분배열"), index=0 ("인덱스")) -> (w304:string[])
                              n184 = Build Array(w304) -> (w303:string[][])
                              n185 = Transpose 2D Array(2D array=w303) -> (transposed array=w302:string[][])
                              n186 = call-poly <vilib>:"Excel Easy Table.vi"("report in"=w312, "font"=T18 {"font name"="", "font size"=11.0, "bold"=0, "italic"=0, "underline"=0, "strike through"=0, "font color"=16777216}, "start (0, 0)"=cluster{"row":i32, "column":i32} {"row"=14, "column"=1}, "text data"=w302, "error in (no error)"=w311) -> ()  [unwired: 6 in, 5 out]
                            }
                            frame #1 {
                              # "Load(lb)"
                              n187 = local read "Test Data table"() -> (w324:string[][])
                              n188 = Index Array(array=w324, index (row) #1=1 ("인덱스 (행)"), index (row) #2=2 ("인덱스 (행)"), index (row) #3=3 ("인덱스 (행)")) -> (element #1=w323:string[], element #2=w322:string[], element #3=w321:string[])  [unwired: 3 in]
                              n189 = Index Array(array=w324, index (row) #1=5 ("인덱스 (행)"), index (row) #2=6 ("인덱스 (행)"), index (row) #3=7 ("인덱스 (행)")) -> (element #1=w320:string[], element #2=w319:string[], element #3=w318:string[])  [unwired: 3 in]
                              n190 = Build Array(w320, w319, w318) -> (w316:string[][])
                              n191 = Build Array(w323, w322, w321) -> (w317:string[][])
                              n192 = Build Array (concatenate)(w317, w316) -> (w315:string[][])
                              n193 = Transpose 2D Array(2D array=w315) -> (transposed array=w314:string[][])
                              n194 = call-poly <vilib>:"Excel Easy Table.vi"("report in"=w331, "font"=T18 {"font name"="", "font size"=11.0, "bold"=0, "italic"=0, "underline"=0, "strike through"=0, "font color"=16777216}, "start (0, 0)"=cluster{"row":i32, "column":i32} {"row"=14, "column"=3}, "text data"=w314, "error in (no error)"=w330) -> ()  [unwired: 6 in, 5 out]
                            }
                          }
                        }
                      }
                    }
                  }
                  n195 = call-dynamic "Save Report to File.vi"("report in"=w209, "report file path"=w203, "error in (no error)"=w208) -> ()  [unwired: 11 in, 2 out]
                }
                frame #3 {
                }
                frame #4 {
                }
              }
            }
            frame #2 {
              n196 = Stop(stop? (T)=TRUE ("정지? (참)")) -> ()
            }
          }
        }
        frame Enabled {
        }
      }
      n197 = call "SUB_Delay ms.vi"("delay(ms)"=u32 100 ("ms 타이머 값")) -> ()  [unwired: 3 in]
    }
    frame #5 {
      # "메인 루프"
      n198 = while {
        i -> [w475]
        stop <- w477 stop-if-true
        n199 = stacked-sequence {
          tunnel: w475 -> [_ w547 _ _ _ _ _ _ _ _ _ _ _ _]
          frame #0 {
            # "통신 연결 관리 - BLE"
            n200 = local read "Port close 1"() -> (w478:bool)
            n201 = local read "Port open 1"() -> (w479:bool)
            n202 = case shown="참" w479 {
              frame False {
              }
              frame True {
                # "통신 연결"
                n203 = stacked-sequence {
                  frame #0 {
                    # "BLE 버퍼 클리어"
                    # "초기화"
                    n204 = call "SUB-BLE Rx data Clear.vi"() -> ()  [unwired: 6 in]
                    n205 = Tick Count (ms)() -> (millisecond timer value=w481:u32)
                    n206 = local write "ACT-Comm"(TRUE ("ACT-RS422")) -> ()
                    n207 = local write "Full ROM data"(FALSE ("Full ROM data")) -> ()
                    n208 = local write "Port open 1"(FALSE) -> ()
                    n209 = Initialize Array(T14 {"RxOK"=FALSE, "ROM Data"=[], "Index"=0} ("클러스터"), 3 ("차원 크기")) -> (w485:T10)
                    n210 = local write "Data trx(led)"(TRUE ("Rx")) -> ()
                    n211 = local write "Rx ROM-log"("" ("문자열-Rx ROM")) -> ()
                    n212 = local write "Timer-ble log"(w481) -> ()
                    n213 = local write "ROM Data"(w485) -> ()
                    n214 = local write "status string"("Communication connection attempt.." ("status string")) -> ()
                  }
                  frame #1 {
                    n215 = local read "Port-set 1"() -> (w490:refnum<visa-resource-name>)
                    n216 = call "_시리얼 포트-초기화.vi"("baud rate"=u32 115200, "시리얼 포트"=w490) -> ("정상"=w492:bool)  [unwired: 2 in, 1 out]
                    n217 = local write "Port-act 1"(w490) -> ()
                    n218 = case shown="참" w492 {
                      tunnel: w490 -> [_ w501]
                      frame False {
                        n219 = local write "Comm con status 1"(FALSE ("Connected")) -> ()
                        n220 = local write "Comm con 1"(FALSE ("보드 통신 연결 1")) -> ()
                        n221 = local write "Rx-mon"(TRUE ("수신 실패(T) 2")) -> ()
                        n222 = local write "RxD"("Can not find COM port" ("status string")) -> ()
                      }
                      frame True {
                        n223 = call "SUB-BLE SCAN.vi"("Port-set 1"=w501) -> ("Device Name"=→"Device Name":string, "Connection Status"=w497:T4, "Connected"=w500:bool)  [unwired: 2 in]
                        "Connection Status" <- w497
                        n224 = Not(x=w500) -> (.not. x?=w499:bool)
                        n225 = local write "Rx-mon"(w499) -> ()
                        n226 = case shown="거짓" w499 {
                          tunnel: w497 -> [_ w509]
                          frame True {
                            # "수신 데이터 에러 상태"
                            n227 = local read "Port-act 1"() -> (w505:refnum<visa-resource-name>)
                            n228 = VISA Close(VISA resource name=w505) -> ()  [unwired: 1 in, 1 out]
                            n229 = local write "Comm con status 1"(FALSE ("Connected")) -> ()
                            n230 = local write "*Board ID1"("None...." ("*Board ID")) -> ()
                            n231 = local write "Comm con 1"(FALSE ("보드 통신 연결 1")) -> ()
                            n232 = local write "Rx-mon"(TRUE ("수신 실패(T) 2")) -> ()
                          }
                          frame False {
                            w511 = T8 {"Left Wing-A, C1/C0"=0.0, "Left Wing-B, C2/C0"=0.0, "Left Wing-C, C3/C0"=0.0, "Right Wing-A, C4/C0"=0.0, "Right Wing-B, C5/C0"=0.0, "Right Wing-C, C6/C0"=0.0} ("CDC data")
                            w510 = T9 {"Gyroscope X"=0.0, "Gyroscope Y"=0.0, "Gyroscope Z"=0.0, "Accelerometer X"=0.0, "Accelerometer Y"=0.0, "Accelerometer Z"=0.0} ("IMU data")
                            # "수신 데이터 정상"
                            n233 = stacked-sequence {
                              tunnel: w509 -> [_ w526 w527]
                              frame #0 {
                                # "BLE 버퍼 클리어"
                                n234 = call "SUB-BLE Rx data Clear.vi"() -> ()  [unwired: 6 in]
                                n235 = Wait Until Next ms Multiple(millisecond multiple=u32 500 ("ms 타이머 값")) -> ()  [unwired: 1 out]
                              }
                              frame #1 {
                                # "데이터 전송\n- 핸들/0x01"
                                n236 = local read "Port-act 1"() -> (w525:refnum<visa-resource-name>)
                                n237 = Tick Count (ms)() -> (millisecond timer value=w524:u32)
                                n238 = Build Array(u16 1 ("Handle")) -> (w523:u16[])
                                n239 = local write "ms timer 4"(w524) -> ()
                                n240 = call-poly "ble_write_by_handle.vi"("Connection Status"=w526, "Handle"=u16 12, "data (uint8array)"=w523, "COM Bluegiga in"=w525) -> ()  [unwired: 6 in, 2 out]
                              }
                              frame #2 {
                                # "데이터 전송\n- 핸들/0x01"
                                n241 = local read "Port-act 1"() -> (w532:refnum<visa-resource-name>)
                                n242 = Tick Count (ms)() -> (millisecond timer value=w531:u32)
                                n243 = Build Array(u16 1 ("Handle")) -> (w530:u16[])
                                n244 = local write "ms timer 4"(w531) -> ()
                                n245 = call-poly "ble_write_by_handle.vi"("Connection Status"=w527, "Handle"=u16 16, "data (uint8array)"=w530, "COM Bluegiga in"=w532) -> ()  [unwired: 6 in, 2 out]
                              }
                            }
                            n246 = local write "*Board ID1"("" ("*Board ID")) -> ()
                            n247 = local write "RxD"("Connection. OK....." ("status string")) -> ()
                            n248 = local write "Setting load(led)"(FALSE ("Power On Flag")) -> ()
                            n249 = local write "Comm con status 1"(TRUE ("Connected")) -> ()
                            n250 = local write "Comm err cnt 1"(0 ("통신에러카운트")) -> ()
                            n251 = local write "Clear graph 1"(TRUE ("그래프 지우기")) -> ()
                            n252 = local write "Clear graph 2"(TRUE ("그래프 지우기")) -> ()
                            n253 = local write "Data_mon(h)"("" ("Data_mon")) -> ()
                            n254 = local write "Data Log"("" ("Data Log")) -> ()
                            n255 = local write "Comm con 1"(TRUE ("포트 연결")) -> ()
                            n256 = local write "CDC Offet"(w511) -> ()
                            n257 = local write "IMU Offet"(w510) -> ()
                            n258 = local write "CDC data"(w511) -> ()
                            n259 = local write "IMU data"(w510) -> ()
                          }
                        }
                      }
                    }
                  }
                  frame #2 {
                    n260 = local write "ACT-Comm"(FALSE ("ACT-RS422")) -> ()
                    n261 = local write "Data trx(led)"(FALSE ("Rx")) -> ()
                  }
                }
              }
            }
            n262 = case shown="참" w478 {
              frame False {
              }
              frame True {
                # "BLE 통신 종료"
                # "포트 닫기"
                n263 = local write "Port close 1"(FALSE ("포트닫기 1")) -> ()
                n264 = local write "Comm con status 1"(FALSE ("Connected")) -> ()
                n265 = local write "*Board ID1"("None...." ("*Board ID")) -> ()
                n266 = local write "status string"("Close communication port." ("status string")) -> ()
                n267 = local write "ACT-Comm"(FALSE ("ACT-RS422")) -> ()
                n268 = local write "Comm con 1"(FALSE ("보드 통신 연결 1")) -> ()
                n269 = local read "Port-act 1"() -> (w535:refnum<visa-resource-name>)
                n270 = local read "Connection Status"() -> (w540:T4)
                n271 = call "_시리얼_buf clear.vi"("시리얼 포트"=w535) -> ("에러 출력"=w538:errorcluster, "시리얼 포트 2"=w539:refnum<visa-resource-name>)  [unwired: 3 in]
                n272 = call "ble_disconnect_device.vi"("Connection Status"=w540, "error in (no error)"=w538, "COM Bluegiga in"=w539) -> ("error out"=w537:errorcluster, "COM Bluegiga out"=w536:refnum<visa-resource-name>)  [unwired: 7 in]
                n273 = VISA Close(VISA resource name=w536, error in (no error)=w537) -> ()  [unwired: 1 out]
              }
            }
          }
          frame #1 {
            # "#BLE_Packet_data_process"
            # "BLE 수신 패킷 데이터 처리"
            n274 = local read "Comm con status 1"() -> (w548:bool)
            n275 = case shown="참" w548 {
              tunnel: w547 -> [_ w554]
              frame False {
              }
              frame True {
                w557 = 80 ("y")
                n276 = call "SUB-BLE Rx data (Mon)-Classify.vi"() -> ("data out"=w553:u8[], "Rx-set"=w551:bool, "Rx-debug"=w550:bool, "Rx-mon"=w552:bool, "Packet No."=w549:i32)  [unwired: 5 in]
                n277 = local write "Packet No."(w549) -> ()
                n278 = stacked-sequence {
                  tunnel: w553 -> [w561 w581 w602]
                  tunnel: w552 -> [w560 _ _]
                  tunnel: w551 -> [_ _ w603]
                  tunnel: w550 -> [_ w582 _]
                  frame #0 {
                    # "Monitoring Data"
                    n279 = case shown="참" w560 {
                      tunnel: w561 -> [_ w568]
                      frame False {
                      }
                      frame True {
                        # "모니터링 데이터 수신 완료"
                        n280 = local read "ms timer"() -> (w577:u32)
                        n281 = local write "Rx-mon"(TRUE ("Rx-mon")) -> ()
                        n282 = local write "Rx-ROM"(FALSE ("Rx-ROM")) -> ()
                        n283 = local write "Rx-debug"(FALSE ("Rx-debug")) -> ()
                        n284 = Tick Count (ms)() -> (millisecond timer value=w576:u32)
                        n285 = call <vilib>:"Space Constant.vi"() -> ("String"=w571:string)
                        n286 = Subtract(x=w576, y=w577) -> (x-y=w574:u32)
                        n287 = local write "BLE Packet (mon)"(w568) -> ()
                        n288 = Array To Spreadsheet String(delimiter (Tab)=w571, array=w568, 3:"%02X" ("포맷 문자열")) -> (spreadsheet string=w569:string)
                        n289 = local write "ms timer"(w576) -> ()
                        n290 = local write "status string"("Receive a monitoring data..." ("status string")) -> ()
                        n291 = Format Into String(format string="[%d ms] " ("포맷 문자열"), w574) -> (resulting string=w573:string)  [unwired: 2 in, 1 out]
                        n292 = local read "ms timer 2"() -> (w565:u32)
                        n293 = Tick Count (ms)() -> (millisecond timer value=w564:u32)
                        n294 = Concatenate Strings(w573, w569) -> (w572:string)
                        n295 = Subtract(x=w564, y=w565) -> (x-y=w563:u32)
                        n296 = case shown="150.." w563 {
                          tunnel: w572 -> [_ w580]
                          frame 0, Default {
                          }
                          frame 150.. {
                            n297 = Tick Count (ms)() -> (millisecond timer value=w579:u32)
                            n298 = local write "RxD"(w580) -> ()
                            n299 = local write "ms timer 2"(w579) -> ()
                          }
                        }
                      }
                    }
                  }
                  frame #1 {
                    # "Debugging Data"
                    n300 = case shown="참" w582 {
                      tunnel: w581 -> [_ w589]
                      frame False {
                      }
                      frame True {
                        # "debugging 데이터 수신 완료"
                        n301 = local read "ms timer"() -> (w598:u32)
                        n302 = local write "Rx-mon"(FALSE ("Rx-mon")) -> ()
                        n303 = local write "Rx-ROM"(FALSE ("Rx-ROM")) -> ()
                        n304 = local write "Rx-debug"(TRUE ("Rx-debug")) -> ()
                        n305 = Tick Count (ms)() -> (millisecond timer value=w597:u32)
                        n306 = call <vilib>:"Space Constant.vi"() -> ("String"=w592:string)
                        n307 = Subtract(x=w597, y=w598) -> (x-y=w595:u32)
                        n308 = local write "BLE Packet (mon)"(w589) -> ()
                        n309 = Array To Spreadsheet String(delimiter (Tab)=w592, array=w589, 3:"%02X" ("포맷 문자열")) -> (spreadsheet string=w590:string)
                        n310 = local write "ms timer"(w597) -> ()
                        n311 = local write "status string"("Receive a debugging data..." ("status string")) -> ()
                        n312 = Format Into String(format string="[%d ms] " ("포맷 문자열"), w595) -> (resulting string=w594:string)  [unwired: 2 in, 1 out]
                        n313 = local read "ms timer 2"() -> (w586:u32)
                        n314 = Tick Count (ms)() -> (millisecond timer value=w585:u32)
                        n315 = Concatenate Strings(w594, w590) -> (w593:string)
                        n316 = Subtract(x=w585, y=w586) -> (x-y=w584:u32)
                        n317 = case shown="150.." w584 {
                          tunnel: w593 -> [_ w601]
                          frame 0, Default {
                          }
                          frame 150.. {
                            n318 = Tick Count (ms)() -> (millisecond timer value=w600:u32)
                            n319 = local write "RxD"(w601) -> ()
                            n320 = local write "ms timer 2"(w600) -> ()
                          }
                        }
                      }
                    }
                  }
                  frame #2 {
                    # "Init data"
                    n321 = case shown="참" w603 {
                      tunnel: w602 -> [_ w606]
                      frame False {
                      }
                      frame True {
                        n322 = local write "Rx-debug"(FALSE ("Rx-debug")) -> ()
                        n323 = local write "Rx-mon"(FALSE ("수신 실패(T) 1")) -> ()
                        n324 = local write "Rx-ROM"(TRUE ("Rx-ROM")) -> ()
                        n325 = stacked-sequence {
                          tunnel: w606 -> [w629 _]
                          frame #0 {
                            # "데이터 입력 상태 체크"
                            n326 = call "SUB-BLE Rx data (Mon)-ROM.vi"("data in"=w629) -> ("data Out"=w614:u8[], "Index"=w615:u8)  [unwired: 3 in]
                            n327 = property on="ROM Data" class="Arr (엄격한)"("Index Values"=u32[] [] ("인덱스 값")) -> ()  [unwired: 2 in, 2 out]
                            n328 = local read "ROM Data"() -> (w628:T10)
                            n329 = Bundle By Name(cluster=T14 {"RxOK"=FALSE, "ROM Data"=[], "Index"=0} ("클러스터"), "RxOK"=TRUE ("Packet Detect"), "ROM Data"=w614, "Index"=w615) -> (w626:T14)
                            n330 = Replace Array Subset(array=w628, new element=w626, index=w615) -> (w612:T10)
                            n331 = local read "Rx ROM-log"() -> (w623:string)
                            n332 = Format Into String(format string="[Packet ID]%02d  " ("포맷 문자열"), w615) -> (resulting string=w617:string)  [unwired: 2 in, 1 out]
                            n333 = for {
                              tunnel: w612 -> [w631] mode=indexing
                              tunnel: [w630] -> w611 mode=indexing
                              n334 = Unbundle By Name(w631) -> ("RxOK"=w630:bool)
                            }
                            n335 = local write "ROM Data"(w612) -> ()
                            n336 = call <vilib>:"Space Constant.vi"() -> ("String"=w616:string)
                            n337 = Array To Spreadsheet String(delimiter (Tab)=w616, array=w614, 3:"%02X" ("포맷 문자열")) -> (spreadsheet string=w619:string)
                            n338 = Format Date/Time String(time format string (%c)="%H:%M:%S%3u>  " ("상태")) -> (date/time string=w621:string)  [unwired: 2 in]
                            n339 = Concatenate Strings(w623, w617, w621, w619) -> (w622:string)
                            n340 = Boolean Array To Number(Boolean array=w611) -> (number=w610:u32)
                            n341 = local write "Rx ROM-log"(w622) -> ()
                            n342 = Equal?(x=w610, y=u32 7) -> (x = y?=w609:bool)
                            n343 = local write "Full ROM data"(w609) -> ()
                          }
                          frame #1 {
                            n344 = control-ref of="ROM Data"() -> (w633:refnum<vi>)
                            n345 = control-ref of="ROM Table"() -> (w632:refnum<vi>)
                            n346 = call "SUB-ROM Data convert to table.vi"("ROM Table Ref"=w632, "ROM Data Ref"=w633) -> ()  [unwired: 2 in, 2 out]
                          }
                        }
                      }
                    }
                  }
                }
                n347 = Quotient & Remainder(x=w554, y=w557) -> (x-y*floor(x/y)=w555:i32)  [unwired: 1 out]
                n348 = Divide(x=w557, y=2) -> (x/y=w558:dbl)
                n349 = Greater?(x=w555, y=w558) -> (0:w556:bool)
                n350 = local write "ACT-Comm"(w556) -> ()
              }
            }
          }
          frame #2 {
            # "모니터링 데이터"
            n351 = local read "Rx-mon"() -> (w634:bool)
            n352 = case shown="참" w634 {
              frame False {
              }
              frame True {
                # "#수신 데이터 처리"
                n353 = local read "ms timer 3"() -> (w639:u32)
                n354 = local read "Update(ms)"() -> (w635:u16)
                n355 = Tick Count (ms)() -> (millisecond timer value=w638:u32)
                n356 = Subtract(x=w638, y=w639) -> (x-y=w636:u32)
                n357 = Greater Or Equal?(x=w636, y=w635) -> (x >= y?=w637:bool)
                n358 = case shown="참" w637 {
                  frame False {
                  }
                  frame True {
                    n359 = local read "BLE Packet (mon)"() -> (w644:u8[])
                    n360 = call "SUB-BLE Rx data (Mon)-CDC IMU.vi"("data in"=w644) -> ("IMU data"=w641:T9, "CDC data"=w642:T8, "Bat"=w640:u16, "*Board ID"=w643:string)  [unwired: 4 in]
                    n361 = stacked-sequence {
                      seq-local: [w647 _ _ _ _ _] -> [_ _ w694 _ w725 _]
                      tunnel: w643 -> [w646 _ _ _ _ _]
                      tunnel: w642 -> [_ w665 _ _ _ _]
                      tunnel: w641 -> [_ _ _ w709 _ _]
                      tunnel: w640 -> [_ _ _ _ _ w747]
                      frame #0 {
                        # "SN"
                        n362 = Tick Count (ms)() -> (millisecond timer value=w645:u32)
                        n363 = local write "ms timer 3"(w645) -> ()
                        n364 = local write "*Board ID1"(w646) -> ()
                        n365 = local read "Graph timer 1"() -> (w648:u32)
                        n366 = Tick Count (ms)() -> (millisecond timer value=w649:u32)
                        n367 = flat-sequence {
                          tunnel: w649 -> [w654]
                          tunnel: w648 -> [w651]
                          tunnel: [w650] -> w647
                          frame #0 {
                            n368 = Subtract(x=w654, y=w651) -> (x-y=w652:u32)
                            n369 = local write "Graph timer 1"(w654) -> ()
                            n370 = Multiply(x=w652, y=0.001 ("dt")) -> (x*y=w650:dbl)
                          }
                        }
                      }
                      frame #1 {
                        # "CDC 데이터"
                        n371 = local read "Offset Souce"() -> (w658:enum32{"Normal", "Raw"})
                        n372 = Unbundle By Name(w665) -> ("Left Wing-A, C1/C0"=w664:dbl, "Left Wing-B, C2/C0"=w663:dbl, "Left Wing-C, C3/C0"=w662:dbl, "Right Wing-A, C4/C0"=w661:dbl, "Right Wing-B, C5/C0"=w660:dbl, "Right Wing-C, C6/C0"=w659:dbl)
                        n373 = Equal?(x=w658, y=enum32{"Normal", "Raw"}."Normal" ("Offset Souce")) -> (x = y?=w656:bool)
                        n374 = case shown="참" w656 {
                          tunnel: [_ w680] -> w655
                          frame False {
                          }
                          frame True {
                            n375 = local read "CDC Offet"() -> (w680:T8)
                          }
                        }
                        n376 = Unbundle By Name(w655) -> ("Left Wing-A, C1/C0"=w679:dbl, "Left Wing-B, C2/C0"=w678:dbl, "Left Wing-C, C3/C0"=w677:dbl, "Right Wing-A, C4/C0"=w676:dbl, "Right Wing-B, C5/C0"=w675:dbl, "Right Wing-C, C6/C0"=w674:dbl)
                        n377 = Subtract(x=w664, y=w679) -> (x-y=w671:dbl)
                        n378 = Subtract(x=w663, y=w678) -> (x-y=w670:dbl)
                        n379 = Subtract(x=w662, y=w677) -> (x-y=w669:dbl)
                        n380 = Subtract(x=w661, y=w676) -> (x-y=w668:dbl)
                        n381 = Subtract(x=w660, y=w675) -> (x-y=w667:dbl)
                        n382 = Subtract(x=w659, y=w674) -> (x-y=w666:dbl)
                        n383 = local read "CDC data"() -> (w673:T8)
                        n384 = Bundle By Name(cluster=w673, "Left Wing-A, C1/C0"=w671, "Left Wing-B, C2/C0"=w670, "Left Wing-C, C3/C0"=w669, "Right Wing-A, C4/C0"=w668, "Right Wing-B, C5/C0"=w667, "Right Wing-C, C6/C0"=w666) -> (w672:T8)
                        n385 = local write "CDC data"(w672) -> ()
                      }
                      frame #2 {
                        # "* 그래프 출력"
                        n386 = local read "CDC data"() -> (w693:T8)
                        n387 = Unbundle By Name(w693) -> ("Left Wing-A, C1/C0"=w692:dbl, "Left Wing-B, C2/C0"=w685:dbl, "Left Wing-C, C3/C0"=w684:dbl, "Right Wing-A, C4/C0"=w683:dbl, "Right Wing-B, C5/C0"=w682:dbl, "Right Wing-C, C6/C0"=w681:dbl)
                        n388 = Build Array(w692) -> (w691:dbl[])
                        n389 = Get Date/Time In Seconds() -> (seconds since 1Jan1904=w697:timestamp)
                        n390 = Build Array(w685) -> (w690:dbl[])
                        n391 = Build Array(w684) -> (w689:dbl[])
                        n392 = Build Array(w682) -> (w687:dbl[])
                        n393 = Build Array(w683) -> (w688:dbl[])
                        n394 = Build Array(w681) -> (w686:dbl[])
                        n395 = Bundle By Name("t0"=w697, "Y"=w691, "dt"=w694) -> (w702:waveform(dbl))  [unwired: 1 in]
                        n396 = Bundle By Name("t0"=w697, "Y"=w690, "dt"=w694) -> (w701:waveform(dbl))  [unwired: 1 in]
                        n397 = Bundle By Name("t0"=w697, "Y"=w689, "dt"=w694) -> (w700:waveform(dbl))  [unwired: 1 in]
                        n398 = Bundle By Name("t0"=w697, "Y"=w688, "dt"=w694) -> (w698:waveform(dbl))  [unwired: 1 in]
                        n399 = Bundle By Name("t0"=w697, "Y"=w687, "dt"=w694) -> (w696:waveform(dbl))  [unwired: 1 in]
                        n400 = Bundle By Name("t0"=w697, "Y"=w686, "dt"=w694) -> (w695:waveform(dbl))  [unwired: 1 in]
                        n401 = Build Array(w702, w701, w700, w698, w696, w695) -> (→"CDC(PCAP02) Graph":waveform(dbl)[])
                      }
                      frame #3 {
                        # "IMU Data"
                        n402 = local read "IMU Offet"() -> (w724:T9)
                        n403 = Unbundle By Name(w709) -> ("Gyroscope X"=w708:dbl, "Gyroscope Y"=w707:dbl, "Gyroscope Z"=w706:dbl, "Accelerometer X"=w705:dbl, "Accelerometer Y"=w704:dbl, "Accelerometer Z"=w703:dbl)
                        n404 = Unbundle By Name(w724) -> ("Gyroscope X"=w721:dbl, "Gyroscope Y"=w720:dbl, "Gyroscope Z"=w719:dbl, "Accelerometer X"=w718:dbl, "Accelerometer Y"=w717:dbl, "Accelerometer Z"=w716:dbl)
                        n405 = Subtract(x=w708, y=w721) -> (x-y=w715:dbl)
                        n406 = Subtract(x=w707, y=w720) -> (x-y=w714:dbl)
                        n407 = Subtract(x=w706, y=w719) -> (x-y=w713:dbl)
                        n408 = Subtract(x=w705, y=w718) -> (x-y=w712:dbl)
                        n409 = Subtract(x=w704, y=w717) -> (x-y=w711:dbl)
                        n410 = Subtract(x=w703, y=w716) -> (x-y=w710:dbl)
                        n411 = local read "IMU data"() -> (w723:T9)
                        n412 = Bundle By Name(cluster=w723, "Gyroscope X"=w715, "Gyroscope Y"=w714, "Gyroscope Z"=w713, "Accelerometer X"=w712, "Accelerometer Y"=w711, "Accelerometer Z"=w710) -> (w722:T9)
                        n413 = local write "IMU data"(w722) -> ()
                      }
                      frame #4 {
                        # "* 그래프 출력"
                        n414 = local read "IMU data"() -> (w738:T9)
                        n415 = Unbundle By Name(w738) -> ("Gyroscope X"=w737:dbl, "Gyroscope Y"=w730:dbl, "Gyroscope Z"=w729:dbl, "Accelerometer X"=w728:dbl, "Accelerometer Y"=w727:dbl, "Accelerometer Z"=w726:dbl)
                        n416 = Build Array(w737) -> (w736:dbl[])
                        n417 = Get Date/Time In Seconds() -> (seconds since 1Jan1904=w741:timestamp)
                        n418 = Build Array(w730) -> (w735:dbl[])
                        n419 = Build Array(w729) -> (w734:dbl[])
                        n420 = Build Array(w727) -> (w732:dbl[])
                        n421 = Build Array(w728) -> (w733:dbl[])
                        n422 = Build Array(w726) -> (w731:dbl[])
                        n423 = Bundle By Name("t0"=w741, "Y"=w736, "dt"=w725) -> (w745:waveform(dbl))  [unwired: 1 in]
                        n424 = Bundle By Name("t0"=w741, "Y"=w735, "dt"=w725) -> (w744:waveform(dbl))  [unwired: 1 in]
                        n425 = Bundle By Name("t0"=w741, "Y"=w734, "dt"=w725) -> (w743:waveform(dbl))  [unwired: 1 in]
                        n426 = Bundle By Name("t0"=w741, "Y"=w733, "dt"=w725) -> (w742:waveform(dbl))  [unwired: 1 in]
                        n427 = Bundle By Name("t0"=w741, "Y"=w732, "dt"=w725) -> (w740:waveform(dbl))  [unwired: 1 in]
                        n428 = Bundle By Name("t0"=w741, "Y"=w731, "dt"=w725) -> (w739:waveform(dbl))  [unwired: 1 in]
                        n429 = Build Array(w745, w744, w743, w742, w740, w739) -> (→"IMU Graph":waveform(dbl)[])
                      }
                      frame #5 {
                        # "BAT raw data"
                        n430 = local write "Bat(raw)"(w747) -> ()
                      }
                    }
                  }
                }
              }
            }
          }
          frame #3 {
            # "Debugging data"
            n431 = local read "Rx-debug"() -> (w748:bool)
            n432 = case shown="참" w748 {
              frame False {
              }
              frame True {
                # "#수신 데이터 처리"
                n433 = local read "ms timer 3"() -> (w753:u32)
                n434 = local read "Update(ms)"() -> (w749:u16)
                n435 = Tick Count (ms)() -> (millisecond timer value=w752:u32)
                n436 = Subtract(x=w752, y=w753) -> (x-y=w750:u32)
                n437 = Greater Or Equal?(x=w750, y=w749) -> (x >= y?=w751:bool)
                n438 = case shown="참" w751 {
                  frame False {
                  }
                  frame True {
                    n439 = local read "BLE Packet (mon)"() -> (w756:u8[])
                    n440 = call "SUB-BLE Rx data (Debug)-CDC.vi"("data in"=w756) -> ("CDC debug"=w754:T8, "CDC mon"=w755:T8)  [unwired: 6 in]
                    n441 = stacked-sequence {
                      seq-local: [w758 _ _ _ _] -> [_ _ _ w833 w852]
                      seq-local: [_ _ _ w819 _] -> [_ _ _ _ w841]
                      seq-local: [_ _ _ w818 _] -> [_ _ _ _ w861]
                      seq-local: [_ _ w792 _ _] -> [_ _ _ _ w840]
                      tunnel: w755 -> [_ w770 _ _ _]
                      tunnel: w754 -> [_ _ w793 _ _]
                      frame #0 {
                        n442 = Tick Count (ms)() -> (millisecond timer value=w757:u32)
                        n443 = local write "ms timer 3"(w757) -> ()
                        n444 = local read "Graph timer 1"() -> (w759:u32)
                        n445 = Tick Count (ms)() -> (millisecond timer value=w760:u32)
                        n446 = flat-sequence {
                          tunnel: w760 -> [w765]
                          tunnel: w759 -> [w762]
                          tunnel: [w761] -> w758
                          frame #0 {
                            n447 = Subtract(x=w765, y=w762) -> (x-y=w763:u32)
                            n448 = local write "Graph timer 1"(w765) -> ()
                            n449 = Multiply(x=w763, y=0.001 ("dt")) -> (x*y=w761:dbl)
                          }
                        }
                      }
                      frame #1 {
                        # "CDC 데이터"
                        n450 = local read "Offset Souce"() -> (w769:enum32{"Normal", "Raw"})
                        n451 = Unbundle By Name(w770) -> ("Left Wing-A, C1/C0"=w776:dbl, "Left Wing-B, C2/C0"=w775:dbl, "Left Wing-C, C3/C0"=w774:dbl, "Right Wing-A, C4/C0"=w773:dbl, "Right Wing-B, C5/C0"=w772:dbl, "Right Wing-C, C6/C0"=w771:dbl)
                        n452 = Equal?(x=w769, y=enum32{"Normal", "Raw"}."Normal" ("Offset Souce")) -> (x = y?=w767:bool)
                        n453 = case shown="참" w767 {
                          tunnel: [_ w791] -> w766
                          frame False {
                          }
                          frame True {
                            n454 = local read "CDC Offet"() -> (w791:T8)
                          }
                        }
                        n455 = Unbundle By Name(w766) -> ("Left Wing-A, C1/C0"=w790:dbl, "Left Wing-B, C2/C0"=w789:dbl, "Left Wing-C, C3/C0"=w788:dbl, "Right Wing-A, C4/C0"=w787:dbl, "Right Wing-B, C5/C0"=w786:dbl, "Right Wing-C, C6/C0"=w785:dbl)
                        n456 = Subtract(x=w776, y=w790) -> (x-y=w782:dbl)
                        n457 = Subtract(x=w775, y=w789) -> (x-y=w781:dbl)
                        n458 = Subtract(x=w774, y=w788) -> (x-y=w780:dbl)
                        n459 = Subtract(x=w773, y=w787) -> (x-y=w779:dbl)
                        n460 = Subtract(x=w772, y=w786) -> (x-y=w778:dbl)
                        n461 = Subtract(x=w771, y=w785) -> (x-y=w777:dbl)
                        n462 = local read "CDC data"() -> (w784:T8)
                        n463 = Bundle By Name(cluster=w784, "Left Wing-A, C1/C0"=w782, "Left Wing-B, C2/C0"=w781, "Left Wing-C, C3/C0"=w780, "Right Wing-A, C4/C0"=w779, "Right Wing-B, C5/C0"=w778, "Right Wing-C, C6/C0"=w777) -> (w783:T8)
                        n464 = local write "CDC data"(w783) -> ()
                      }
                      frame #2 {
                        n465 = local read "Offset Souce"() -> (w797:enum32{"Normal", "Raw"})
                        n466 = Unbundle By Name(w793) -> ("Left Wing-A, C1/C0"=w803:dbl, "Left Wing-B, C2/C0"=w802:dbl, "Left Wing-C, C3/C0"=w801:dbl, "Right Wing-A, C4/C0"=w800:dbl, "Right Wing-B, C5/C0"=w799:dbl, "Right Wing-C, C6/C0"=w798:dbl)
                        n467 = Equal?(x=w797, y=enum32{"Normal", "Raw"}."Raw" ("Offset Souce")) -> (x = y?=w795:bool)
                        n468 = case shown="참" w795 {
                          tunnel: [_ w817] -> w794
                          frame False {
                          }
                          frame True {
                            n469 = local read "CDC Offet"() -> (w817:T8)
                          }
                        }
                        n470 = Unbundle By Name(w794) -> ("Left Wing-A, C1/C0"=w816:dbl, "Left Wing-B, C2/C0"=w815:dbl, "Left Wing-C, C3/C0"=w814:dbl, "Right Wing-A, C4/C0"=w813:dbl, "Right Wing-B, C5/C0"=w812:dbl, "Right Wing-C, C6/C0"=w811:dbl)
                        n471 = Subtract(x=w803, y=w816) -> (x-y=w809:dbl)
                        n472 = Subtract(x=w802, y=w815) -> (x-y=w808:dbl)
                        n473 = Subtract(x=w801, y=w814) -> (x-y=w807:dbl)
                        n474 = Subtract(x=w800, y=w813) -> (x-y=w806:dbl)
                        n475 = Subtract(x=w799, y=w812) -> (x-y=w805:dbl)
                        n476 = Subtract(x=w798, y=w811) -> (x-y=w804:dbl)
                        n477 = local read "CDC data"() -> (w810:T8)
                        n478 = Bundle By Name(cluster=w810, "Left Wing-A, C1/C0"=w809, "Left Wing-B, C2/C0"=w808, "Left Wing-C, C3/C0"=w807, "Right Wing-A, C4/C0"=w806, "Right Wing-B, C5/C0"=w805, "Right Wing-C, C6/C0"=w804) -> (w792:T8)
                      }
                      frame #3 {
                        # "* 그래프 출력"
                        n479 = local read "CDC data"() -> (w832:T8)
                        n480 = Unbundle By Name(w832) -> ("Left Wing-A, C1/C0"=w831:dbl, "Left Wing-B, C2/C0"=w824:dbl, "Left Wing-C, C3/C0"=w823:dbl, "Right Wing-A, C4/C0"=w822:dbl, "Right Wing-B, C5/C0"=w821:dbl, "Right Wing-C, C6/C0"=w820:dbl)
                        n481 = Build Array(w831) -> (w830:dbl[])
                        n482 = Get Date/Time In Seconds() -> (seconds since 1Jan1904=w819:timestamp)
                        n483 = Build Array(w824) -> (w829:dbl[])
                        n484 = Build Array(w823) -> (w828:dbl[])
                        n485 = Build Array(w821) -> (w826:dbl[])
                        n486 = Build Array(w822) -> (w827:dbl[])
                        n487 = Build Array(w820) -> (w825:dbl[])
                        n488 = Bundle By Name("t0"=w819, "Y"=w830, "dt"=w833) -> (w839:waveform(dbl))  [unwired: 1 in]
                        n489 = Bundle By Name("t0"=w819, "Y"=w829, "dt"=w833) -> (w838:waveform(dbl))  [unwired: 1 in]
                        n490 = Bundle By Name("t0"=w819, "Y"=w828, "dt"=w833) -> (w837:waveform(dbl))  [unwired: 1 in]
                        n491 = Bundle By Name("t0"=w819, "Y"=w827, "dt"=w833) -> (w836:waveform(dbl))  [unwired: 1 in]
                        n492 = Bundle By Name("t0"=w819, "Y"=w826, "dt"=w833) -> (w835:waveform(dbl))  [unwired: 1 in]
                        n493 = Bundle By Name("t0"=w819, "Y"=w825, "dt"=w833) -> (w834:waveform(dbl))  [unwired: 1 in]
                        n494 = Build Array(w839, w838, w837, w836, w835, w834) -> (w818:waveform(dbl)[])
                      }
                      frame #4 {
                        n495 = Unbundle By Name(w840) -> ("Left Wing-A, C1/C0"=w859:dbl, "Left Wing-B, C2/C0"=w858:dbl, "Left Wing-C, C3/C0"=w845:dbl, "Right Wing-A, C4/C0"=w844:dbl, "Right Wing-B, C5/C0"=w843:dbl, "Right Wing-C, C6/C0"=w842:dbl)
                        n496 = Build Array(w859) -> (w860:dbl[])
                        n497 = Build Array(w844) -> (w850:dbl[])
                        n498 = Build Array(w858) -> (w857:dbl[])
                        n499 = Build Array(w845) -> (w856:dbl[])
                        n500 = Build Array(w843) -> (w853:dbl[])
                        n501 = Build Array(w842) -> (w854:dbl[])
                        n502 = Bundle By Name("t0"=w841, "Y"=w860, "dt"=w852) -> (w862:waveform(dbl))  [unwired: 1 in]
                        n503 = Bundle By Name("t0"=w841, "Y"=w857, "dt"=w852) -> (w855:waveform(dbl))  [unwired: 1 in]
                        n504 = Bundle By Name("t0"=w841, "Y"=w856, "dt"=w852) -> (w851:waveform(dbl))  [unwired: 1 in]
                        n505 = Bundle By Name("t0"=w841, "Y"=w850, "dt"=w852) -> (w849:waveform(dbl))  [unwired: 1 in]
                        n506 = Bundle By Name("t0"=w841, "Y"=w853, "dt"=w852) -> (w848:waveform(dbl))  [unwired: 1 in]
                        n507 = Bundle By Name("t0"=w841, "Y"=w854, "dt"=w852) -> (w847:waveform(dbl))  [unwired: 1 in]
                        n508 = Build Array (concatenate)(w861, w862, w855, w851, w849, w848, w847) -> (w846:waveform(dbl)[])
                        n509 = local write "CDC(PCAP02) Graph"(w846) -> ()
                      }
                    }
                  }
                }
              }
            }
          }
          frame #4 {
            # "Force Test"
            n510 = local read "Comm con status 1"() -> (w864:bool)
            n511 = local read "Test Start"() -> (w863:bool)
            n512 = case shown="참" w864 {
              tunnel: w863 -> [_ w868]
              frame False {
                n513 = local write "FTS Testing"(FALSE ("FTS 시험 진행")) -> ()
                n514 = local write "Test Start"(FALSE ("Test Start")) -> ()
                n515 = local write "FTS comm."(FALSE ("FTS 수신 정상")) -> ()
              }
              frame True {
                n516 = case shown="참" w868 {
                  frame False {
                  }
                  frame True {
                    n517 = stacked-sequence {
                      frame #0 {
                        # "Test Mode"
                        # "Calibration Mode"
                        # "가로"
                        # "세로"
                        # "초기화"
                        n518 = local read "Cal/Test select"() -> (w872:bool)
                        n519 = Wait Until Next ms Multiple(millisecond multiple=u32 100 ("ms 배수")) -> ()  [unwired: 1 out]
                        n520 = Select(t=7, s=w872, f=5) -> (s? t:f=w869:i32)
                        n521 = for {
                          N: 9 -> [_]
                          tunnel: [w886] -> w877 mode=indexing
                          tunnel: w869 -> [w885]
                          # "가로"
                          n522 = for {
                            N: w885 -> [_]
                            tunnel: ["-"] -> w886 mode=indexing
                          }
                        }
                        n523 = local write "Mark10 Gauge (lb)"(0.0 ("Mark10 Gauge")) -> ()
                        n524 = local write "FTS Testing"(TRUE ("FTS 시험 진행")) -> ()
                        n525 = local write "FTS comm."(FALSE ("FTS 수신 정상")) -> ()
                        n526 = local write "FTS OP status"(T6 "시험 시작" ("FTS 동작시험 상태")) -> ()
                        n527 = local write "status string"("Force Test Mode..." ("status string")) -> ()
                        n528 = Format Date/Time String(time format string (%c)="%Y/%m/%d %H:%M:%S> Force Test Start\n" ("상태")) -> (date/time string=w875:string)  [unwired: 2 in]
                        n529 = local write "Test Data table"(w877) -> ()
                        n530 = local write "Test Status"(w875) -> ()
                        n531 = local write "FTS table index"(0 ("FTS table index")) -> ()
                        n532 = local write "Load vs CDC Graph"(cluster{dbl[], dbl[]}[] [] ("Load vs Ratio Graph")) -> ()
                      }
                      frame #1 {
                        w889 = "Offset\nLoad(1)-0lb\nLoad(2)-20lb\nLoad(3)-40lb\nLoad(4)-80lb"  # FTS data Table name 1
                        w893 = "Load(1)-0lb\t0\t10000\t1\t1\t0\nLoad(2)-20lb\t20\t3000\t0\t1\t0\nLoad(3)-40lb\t40\t3000\t0\t1\t0\nLoad(4)-80lb\t80\t3000\t0\t1\t1"  # FTS Profile 2
                        w894 = "Load(1)-0lb\t0\t2000\t0\t0\t0\nInit(1)-70lb\t70\t100\t0\t0\t0\nInit(2)-140lb\t140\t100\t0\t0\t0\nInit(1)-70lb\t70\t100\t0\t0\t0\nInit(2)-140lb\t140\t100\t0\t0\t1\nLoad(1)-0lb\t0\t10000\t1\t1\t0\nLoad(2)-10lb\t10\t3000\t0\t1\t0\nLoad(3)-20lb\t20\t3000\t0\t1\t0\nLoad(4)-40lb\t40\t3000\t0\t1\t0\nLoad(5)-60lb\t60\t3000\t0\t1\t0\nLoad(6)-80lb\t80\t3000\t0\t1\t1"  # FTS Profile 1
                        w891 = "Offset\nLoad(1)-0lb\nLoad(2)-10lb\nLoad(3)-20lb\nLoad(4)-40lb\nLoad(5)-60lb\nLoad(6)-80lb"  # FTS data Table name 1
                        # "#FTS_PROFILE"
                        # "Test Mode"
                        # "Calibration Mode"
                        # "압력 시험용 프로파일\n(시험명, 인가압력, 시간)"
                        n533 = local read "Cal/Test select"() -> (w890:bool)
                        n534 = Select(t=w894, s=w890, f=w893) -> (s? t:f=w892:string)
                        n535 = Spreadsheet String To Array(format string="%s" ("포맷 문자열"), spreadsheet string=w892, array type (2D Dbl)=string[][] [] ("배열 타입(2D Dbl)")) -> (array=w898:string[][])  [unwired: 1 in]
                        n536 = local write "Test profile"(w898) -> ()
                        n537 = Select(t=w891, s=w890, f=w889) -> (s? t:f=w888:string)
                        n538 = call "SUB-module-여러줄 문자열을 배열로 변환.vi"("문자열"=w888) -> ("배열"=w895:string[])
                        n539 = property on="Test Data table" class="Tbl (엄격한)"("Column Headers[]"=w895) -> ()  [unwired: 2 in, 2 out]
                      }
                      frame #2 {
                        n540 = local read "Port-FTS"() -> (w904:refnum<visa-resource-name>)
                        n541 = control-ref of="Test Status"() -> (w900:refnum<vi>)
                        n542 = call "_시리얼_Mark10-연결확인.vi"("시리얼 포트"=w904) -> ("수신 정상"=w903:bool, "VISA resource name out"=w902:refnum<visa-resource-name>)  [unwired: 3 in]
                        n543 = call "SUB-Status string update.vi"("텍스트 입력"="Check Serial port of Mark-10\n" ("Force Test Status"), "날짜추가"=TRUE, "reference"=w900) -> ()  [unwired: 2 in, 1 out]
                        n544 = local write "FTS comm."(w903) -> ()
                        n545 = case shown="거짓" w903 {
                          tunnel: w902 -> [_ _]
                          frame False {
                            # "통신 불량"
                            n546 = local write "FTS OP status"(T6 "시험 종료" ("FTS 동작시험 상태")) -> ()
                            n547 = One Button Dialog(message="Cannot find MARK10.\nCheck comm port." ("메시지")) -> ()  [unwired: 1 in, 1 out]
                          }
                          frame True {
                          }
                        }
                      }
                      frame #3 {
                        n548 = while {
                          stop <- w908 stop-if-true
                          # "시험 프로파일"
                          n549 = local read "FTS OP status"() -> (w909:T6)
                          n550 = local read "Test profile"() -> (w907:string[][])
                          n551 = case shown="\"시험 진행-압력시험\"" w909 {
                            tunnel: [w914 _ _ _ _ TRUE] -> w908
                            tunnel: w907 -> [_ _ _ w964 _ _]
                            frame "시험 시작" {
                              n552 = control-ref of="Test Status"() -> (w911:refnum<vi>)
                              n553 = local write "FTS OP status"(T6 "시험전 점검" ("FTS 동작시험 상태")) -> ()
                              n554 = call "SUB-Status string update.vi"("텍스트 입력"="Force Test Start!\n" ("Force Test Status"), "날짜추가"=TRUE, "reference"=w911) -> ()  [unwired: 2 in, 1 out]
                              n555 = local read "stop"() -> (w914:bool)
                            }
                            frame "시험전 점검" {
                              n556 = local read "Port-FTS"() -> (w916:refnum<visa-resource-name>)
                              n557 = call "_시리얼_Mark10-데이터 수신 (게이지).vi"("시리얼 포트"=w916) -> ("데이터(lb)"=w915:dbl, "수신 정상"=w917:bool)  [unwired: 2 in, 1 out]
                              n558 = local write "Mark10 Gauge (lb)"(w915) -> ()
                              n559 = local write "FTS comm."(w917) -> ()
                              n560 = local write "FTS OP status"(T6 "시험 진행-CDC 옵셋" ("FTS 동작시험 상태")) -> ()
                            }
                            frame "시험 진행-CDC 옵셋" {
                              n561 = disable-structure shown="비활성화" {
                                frame Disabled {
                                n562 = stacked-sequence {
                                frame #0 {
                                n563 = control-ref of="Test Status"() -> (w921:refnum<vi>)
                                n564 = call "SUB-Status string update.vi"("텍스트 입력"="Offset data set... start" ("Force Test Status"), "날짜추가"=TRUE, "reference"=w921) -> ()  [unwired: 2 in, 1 out]
                                }
                                frame #1 {
                                n565 = Wait Until Next ms Multiple(millisecond multiple=u32 500 ("ms 배수")) -> ()  [unwired: 1 out]
                                }
                                frame #2 {
                                # "BLE 버퍼 클리어"
                                n566 = call "SUB-BLE Rx data Clear.vi"() -> ()  [unwired: 6 in]
                                }
                                frame #3 {
                                n567 = Wait Until Next ms Multiple(millisecond multiple=u32 500 ("ms 배수")) -> ()  [unwired: 1 out]
                                }
                                frame #4 {
                                n568 = for {
                                N: 50 -> [_]
                                tunnel: [w947] -> w938 mode=indexing
                                tunnel: [w946] -> w937 mode=indexing
                                tunnel: [w945] -> w936 mode=indexing
                                tunnel: [w944] -> w935 mode=indexing
                                tunnel: [w943] -> w934 mode=indexing
                                tunnel: [w942] -> w933 mode=indexing
                                n569 = local read "CDC Offet"() -> (w941:T8)
                                n570 = local read "Test Status"() -> (w952:string)
                                n571 = call "SUB-BLE Rx data (Mon)-Wait.vi"("Timeout(ms)"=u16 100) -> ("RxReady"=w948:bool)  [unwired: 4 in]
                                n572 = case shown="참" w948 {
                                tunnel: [w954 w955] -> w940
                                tunnel: w941 -> [w954 _]
                                frame False {
                                }
                                frame True {
                                n573 = call "SUB-BLE Rx data (Mon)-Classify.vi"() -> ("data out"=w956:u8[])  [unwired: 3 in, 2 out]
                                n574 = call "SUB-BLE Rx data (Mon)-CDC IMU.vi"("data in"=w956) -> ("CDC data"=w955:T8)  [unwired: 4 in, 3 out]
                                }
                                }
                                n575 = local write "CDC Offet"(w940) -> ()
                                n576 = Concatenate Strings(w952, ".") -> (w953:string)
                                n577 = local write "Test Status"(w953) -> ()
                                n578 = Unbundle By Name(w940) -> ("Left Wing-A, C1/C0"=w947:dbl, "Left Wing-B, C2/C0"=w946:dbl, "Left Wing-C, C3/C0"=w945:dbl, "Right Wing-A, C4/C0"=w944:dbl, "Right Wing-B, C5/C0"=w943:dbl, "Right Wing-C, C6/C0"=w942:dbl)
                                n579 = Wait Until Next ms Multiple(millisecond multiple=u32 5 ("ms 배수")) -> ()  [unwired: 1 out]
                                }
                                n580 = call-poly <vilib>:"Mean.vi"("X"=w938) -> ("mean"=w931:dbl)  [unwired: 1 out]
                                n581 = call-poly <vilib>:"Mean.vi"("X"=w937) -> ("mean"=w930:dbl)  [unwired: 1 out]
                                n582 = call-poly <vilib>:"Mean.vi"("X"=w936) -> ("mean"=w929:dbl)  [unwired: 1 out]
                                n583 = call-poly <vilib>:"Mean.vi"("X"=w935) -> ("mean"=w928:dbl)  [unwired: 1 out]
                                n584 = call-poly <vilib>:"Mean.vi"("X"=w934) -> ("mean"=w927:dbl)  [unwired: 1 out]
                                n585 = call-poly <vilib>:"Mean.vi"("X"=w933) -> ("mean"=w926:dbl)  [unwired: 1 out]
                                n586 = Bundle By Name(cluster=T8 {"Left Wing-A, C1/C0"=0.0, "Left Wing-B, C2/C0"=0.0, "Left Wing-C, C3/C0"=0.0, "Right Wing-A, C4/C0"=0.0, "Right Wing-B, C5/C0"=0.0, "Right Wing-C, C6/C0"=0.0} ("CDC data"), "Left Wing-A, C1/C0"=w931, "Left Wing-B, C2/C0"=w930, "Left Wing-C, C3/C0"=w929, "Right Wing-A, C4/C0"=w928, "Right Wing-B, C5/C0"=w927, "Right Wing-C, C6/C0"=w926) -> (w932:T8)
                                n587 = local write "CDC Offet"(w932) -> ()
                                }
                                frame #5 {
                                n588 = local read "Test Status"() -> (w958:string)
                                n589 = Concatenate Strings(w958, "\n") -> (w959:string)
                                n590 = local write "Test Status"(w959) -> ()
                                }
                                frame #6 {
                                n591 = control-ref of="Test Status"() -> (w962:refnum<vi>)
                                n592 = call "SUB-Status string update.vi"("텍스트 입력"="Offset data set... done\n" ("Force Test Status"), "날짜추가"=TRUE, "reference"=w962) -> ()  [unwired: 2 in, 1 out]
                                n593 = local write "FTS OP status"(T6 "시험 진행-압력시험" ("FTS 동작시험 상태")) -> ()
                                }
                                }
                                }
                                frame Enabled {
                                }
                              }
                              n594 = local write "FTS OP status"(T6 "시험 진행-압력시험" ("FTS 동작시험 상태")) -> ()
                            }
                            frame "시험 진행-압력시험" {
                              n595 = stacked-sequence {
                                tunnel: w964 -> [_ w968 _ _]
                                frame #0 {
                                n596 = control-ref of="Test Status"() -> (w966:refnum<vi>)
                                n597 = call "SUB-Status string update.vi"("텍스트 입력"="Start Force test by Profile" ("Force Test Status"), "날짜추가"=TRUE, "reference"=w966) -> ()  [unwired: 2 in, 1 out]
                                }
                                frame #1 {
                                n598 = for {
                                tunnel: w968 -> [w971] mode=indexing
                                i -> [w969]
                                stop <- w970 continue-if-true
                                n599 = stacked-sequence {
                                tunnel: w969 -> [w975 _ _ _ _ _ _ _ _ _]
                                tunnel: w971 -> [w974 w987 w991 _ _ w1005 _ w1104 _ w1151]
                                tunnel: [_ w982 _ _ _ _ _ _ _ _] -> w970
                                frame #0 {
                                # "진행 상태 문자열"
                                n600 = Index Array(array=w974, index=0 ("인덱스")) -> (element=w972:string)
                                n601 = Increment(x=w975) -> (x+1=w976:i32)
                                n602 = control-ref of="Test Status"() -> (w979:refnum<vi>)
                                n603 = Format Into String(format string="Force Testing-Profile(%d)...%s" ("Force Test Status"), w976, w972) -> (resulting string=w978:string)  [unwired: 2 in, 1 out]
                                n604 = call "SUB-Status string update.vi"("텍스트 입력"=w978, "날짜추가"=TRUE, "reference"=w979) -> ()  [unwired: 2 in, 1 out]
                                }
                                frame #1 {
                                # "압력 인가"
                                n605 = Index Array(array=w987, index=1 ("인덱스")) -> (element=w985:string)
                                n606 = local read "Port-FTS"() -> (w988:refnum<visa-resource-name>)
                                n607 = Fract/Exp String To Number(string=w985) -> (number=w984:dbl)  [unwired: 3 in, 1 out]
                                n608 = call "_시리얼_Mark10-제어 (압력설정).vi"("FTS 제어 상태"=T20 "압력제어 시작", "압력 설정(lb)"=w984, "시리얼 포트"=w988) -> ("게이지 압력(lb)"=w981:dbl, "통신 정상"=w982:bool)  [unwired: 1 out]
                                n609 = local write "Mark10 Gauge (lb)"(w981) -> ()
                                n610 = local write "FTS comm."(w982) -> ()
                                }
                                frame #2 {
                                # "대기 시간."
                                n611 = Tick Count (ms)() -> (millisecond timer value=w990:u32)
                                n612 = Index Array(array=w991, index=2 ("인덱스")) -> (element=w992:string)
                                n613 = Fract/Exp String To Number(string=w992) -> (number=w989:dbl)  [unwired: 3 in, 1 out]
                                n614 = while {
                                tunnel: w990 -> [w1000]
                                tunnel: w989 -> [w998]
                                stop <- w997 stop-if-true
                                n615 = Tick Count (ms)() -> (millisecond timer value=w1001:u32)
                                n616 = Subtract(x=w1001, y=w1000) -> (x-y=w999:u32)
                                n617 = local read "Port-FTS"() -> (w994:refnum<visa-resource-name>)
                                n618 = Greater Or Equal?(x=w999, y=w998) -> (x >= y?=w997:bool)
                                n619 = call "_시리얼_Mark10-데이터 수신 (게이지).vi"("시리얼 포트"=w994) -> ("데이터(lb)"=w995:dbl)  [unwired: 2 in, 2 out]
                                n620 = local write "Mark10 Gauge (lb)"(w995) -> ()
                                n621 = Wait Until Next ms Multiple(millisecond multiple=u32 50 ("ms 배수")) -> ()  [unwired: 1 out]
                                }
                                }
                                frame #3 {
                                # "BLE 버퍼 클리어"
                                n622 = call "SUB-BLE Rx data Clear.vi"() -> ()  [unwired: 6 in]
                                }
                                frame #4 {
                                n623 = Wait Until Next ms Multiple(millisecond multiple=u32 500 ("ms 배수")) -> ()  [unwired: 1 out]
                                }
                                frame #5 {
                                # "Offset"
                                n624 = Index Array(array=w1005, index=3 ("인덱스")) -> (element=w1006:string)
                                n625 = Fract/Exp String To Number(string=w1006) -> (number=w1004:dbl)  [unwired: 3 in, 1 out]
                                n626 = Not Equal To 0?(x=w1004) -> (x != 0?=w1003:bool)
                                n627 = case shown="참" w1003 {
                                frame False {
                                }
                                frame True {
                                n628 = stacked-sequence {
                                frame #0 {
                                # "Offset"
                                n629 = for {
                                N: 50 -> [_]
                                tunnel: [w1030] -> w1021 mode=indexing
                                tunnel: [w1029] -> w1020 mode=indexing
                                tunnel: [w1028] -> w1019 mode=indexing
                                tunnel: [w1027] -> w1018 mode=indexing
                                tunnel: [w1026] -> w1017 mode=indexing
                                tunnel: [w1025] -> w1016 mode=indexing
                                n630 = local read "CDC Offet"() -> (w1024:T8)
                                n631 = call "SUB-BLE Rx data (Mon)-Wait.vi"("Timeout(ms)"=u16 100) -> ("RxReady"=w1031:bool)  [unwired: 4 in]
                                n632 = case shown="참" w1031 {
                                tunnel: [w1034 w1035] -> w1023
                                tunnel: w1024 -> [w1034 _]
                                frame False {
                                }
                                frame True {
                                n633 = call "SUB-BLE Rx data (Mon)-Classify.vi"() -> ("data out"=w1036:u8[])  [unwired: 5 in, 4 out]
                                n634 = call "SUB-BLE Rx data (Mon)-CDC IMU.vi"("data in"=w1036) -> ("CDC data"=w1035:T8)  [unwired: 4 in, 3 out]
                                }
                                }
                                n635 = local write "CDC Offet"(w1023) -> ()
                                n636 = Unbundle By Name(w1023) -> ("Left Wing-A, C1/C0"=w1030:dbl, "Left Wing-B, C2/C0"=w1029:dbl, "Left Wing-C, C3/C0"=w1028:dbl, "Right Wing-A, C4/C0"=w1027:dbl, "Right Wing-B, C5/C0"=w1026:dbl, "Right Wing-C, C6/C0"=w1025:dbl)
                                n637 = Wait Until Next ms Multiple(millisecond multiple=u32 5 ("ms 배수")) -> ()  [unwired: 1 out]
                                }
                                n638 = call-poly <vilib>:"Mean.vi"("X"=w1021) -> ("mean"=w1013:dbl)  [unwired: 1 out]
                                n639 = call-poly <vilib>:"Mean.vi"("X"=w1020) -> ("mean"=w1012:dbl)  [unwired: 1 out]
                                n640 = call-poly <vilib>:"Mean.vi"("X"=w1019) -> ("mean"=w1011:dbl)  [unwired: 1 out]
                                n641 = call-poly <vilib>:"Mean.vi"("X"=w1018) -> ("mean"=w1010:dbl)  [unwired: 1 out]
                                n642 = call-poly <vilib>:"Mean.vi"("X"=w1017) -> ("mean"=w1009:dbl)  [unwired: 1 out]
                                n643 = call-poly <vilib>:"Mean.vi"("X"=w1016) -> ("mean"=w1008:dbl)  [unwired: 1 out]
                                n644 = Bundle By Name(cluster=T8 {"Left Wing-A, C1/C0"=0.0, "Left Wing-B, C2/C0"=0.0, "Left Wing-C, C3/C0"=0.0, "Right Wing-A, C4/C0"=0.0, "Right Wing-B, C5/C0"=0.0, "Right Wing-C, C6/C0"=0.0} ("CDC data"), "Left Wing-A, C1/C0"=w1013, "Left Wing-B, C2/C0"=w1012, "Left Wing-C, C3/C0"=w1011, "Right Wing-A, C4/C0"=w1010, "Right Wing-B, C5/C0"=w1009, "Right Wing-C, C6/C0"=w1008) -> (w1014:T8)
                                n645 = local write "CDC Offet"(w1014) -> ()
                                }
                                frame #1 {
                                w1040 = "-"
                                w1046 = i16 1 ("정밀도(6)")
                                n646 = local read "CDC Offet"() -> (w1059:T8)
                                n647 = Unbundle By Name(w1059) -> ("Left Wing-A, C1/C0"=w1058:dbl, "Left Wing-B, C2/C0"=w1057:dbl, "Left Wing-C, C3/C0"=w1056:dbl, "Right Wing-A, C4/C0"=w1052:dbl, "Right Wing-B, C5/C0"=w1051:dbl, "Right Wing-C, C6/C0"=w1050:dbl)
                                n648 = local read "FTS table index"() -> (w1037:i32)
                                n649 = local read "Mark10 Gauge (lb)"() -> (w1042:dbl)
                                n650 = local read "Test Data table"() -> (w1043:string[][])
                                n651 = Number To Fractional String(number=w1042, precision (6)=i16 2 ("정밀도(6)")) -> (F-format string=w1039:string)  [unwired: 2 in]
                                n652 = Number To Fractional String(number=w1058, precision (6)=w1046) -> (F-format string=w1055:string)  [unwired: 2 in]
                                n653 = Number To Fractional String(number=w1057, precision (6)=w1046) -> (F-format string=w1054:string)  [unwired: 2 in]
                                n654 = Number To Fractional String(number=w1056, precision (6)=w1046) -> (F-format string=w1053:string)  [unwired: 2 in]
                                n655 = Number To Fractional String(number=w1052, precision (6)=w1046) -> (F-format string=w1049:string)  [unwired: 2 in]
                                n656 = Number To Fractional String(number=w1051, precision (6)=w1046) -> (F-format string=w1048:string)  [unwired: 2 in]
                                n657 = Number To Fractional String(number=w1050, precision (6)=w1046) -> (F-format string=w1047:string)  [unwired: 2 in]
                                n658 = Build Array(w1039, w1055, w1054, w1053, w1040, w1049, w1048, w1047, w1040) -> (w1045:string[])
                                n659 = Replace Array Subset(array=w1043, new element=w1045, index (col)=w1037) -> (w1044:string[][])  [unwired: 1 in]
                                n660 = local write "Test Data table"(w1044) -> ()
                                n661 = Increment(x=w1037) -> (x+1=w1038:i32)
                                n662 = local write "FTS table index"(w1038) -> ()
                                }
                                frame #2 {
                                n663 = Wait Until Next ms Multiple(millisecond multiple=u32 500 ("ms 배수")) -> ()  [unwired: 1 out]
                                }
                                }
                                }
                                }
                                }
                                frame #6 {
                                # "CDC 데이터 수집"
                                n664 = for {
                                N: 10 -> [_]
                                tunnel: [w1096] -> w1061 mode=indexing
                                tunnel: [w1095] -> w1087 mode=indexing
                                tunnel: [w1094] -> w1086 mode=indexing
                                tunnel: [w1093] -> w1085 mode=indexing
                                tunnel: [w1092] -> w1084 mode=indexing
                                tunnel: [w1091] -> w1083 mode=indexing
                                n665 = local read "CDC data"() -> (w1089:T8)
                                n666 = call "SUB-BLE Rx data (Mon)-Wait.vi"("Timeout(ms)"=u16 100) -> ("RxReady"=w1097:bool)  [unwired: 4 in]
                                n667 = case shown="참" w1097 {
                                tunnel: [w1100 w1101] -> w1090
                                tunnel: w1089 -> [w1100 _]
                                frame False {
                                }
                                frame True {
                                n668 = call "SUB-BLE Rx data (Mon)-Classify.vi"() -> ("data out"=w1102:u8[])  [unwired: 5 in, 4 out]
                                n669 = call "SUB-BLE Rx data (Mon)-CDC IMU.vi"("data in"=w1102) -> ("CDC data"=w1101:T8)  [unwired: 4 in, 3 out]
                                }
                                }
                                n670 = Unbundle By Name(w1090) -> ("Left Wing-A, C1/C0"=w1096:dbl, "Left Wing-B, C2/C0"=w1095:dbl, "Left Wing-C, C3/C0"=w1094:dbl, "Right Wing-A, C4/C0"=w1093:dbl, "Right Wing-B, C5/C0"=w1092:dbl, "Right Wing-C, C6/C0"=w1091:dbl)
                                n671 = Wait Until Next ms Multiple(millisecond multiple=u32 5 ("ms 배수")) -> ()  [unwired: 1 out]
                                }
                                n672 = local read "CDC Offet"() -> (w1080:T8)
                                n673 = Unbundle By Name(w1080) -> ("Left Wing-A, C1/C0"=w1067:dbl, "Left Wing-B, C2/C0"=w1066:dbl, "Left Wing-C, C3/C0"=w1065:dbl, "Right Wing-A, C4/C0"=w1064:dbl, "Right Wing-B, C5/C0"=w1063:dbl, "Right Wing-C, C6/C0"=w1062:dbl)
                                n674 = call-poly <vilib>:"Mean.vi"("X"=w1061) -> ("mean"=w1073:dbl)  [unwired: 1 out]
                                n675 = call-poly <vilib>:"Mean.vi"("X"=w1087) -> ("mean"=w1072:dbl)  [unwired: 1 out]
                                n676 = call-poly <vilib>:"Mean.vi"("X"=w1086) -> ("mean"=w1071:dbl)  [unwired: 1 out]
                                n677 = call-poly <vilib>:"Mean.vi"("X"=w1085) -> ("mean"=w1070:dbl)  [unwired: 1 out]
                                n678 = call-poly <vilib>:"Mean.vi"("X"=w1084) -> ("mean"=w1069:dbl)  [unwired: 1 out]
                                n679 = call-poly <vilib>:"Mean.vi"("X"=w1083) -> ("mean"=w1068:dbl)  [unwired: 1 out]
                                n680 = Subtract(x=w1073, y=w1067) -> (x-y=w1079:dbl)
                                n681 = Subtract(x=w1072, y=w1066) -> (x-y=w1078:dbl)
                                n682 = Subtract(x=w1071, y=w1065) -> (x-y=w1077:dbl)
                                n683 = Subtract(x=w1070, y=w1064) -> (x-y=w1076:dbl)
                                n684 = Subtract(x=w1069, y=w1063) -> (x-y=w1075:dbl)
                                n685 = Subtract(x=w1068, y=w1062) -> (x-y=w1074:dbl)
                                n686 = Bundle By Name(cluster=T8 {"Left Wing-A, C1/C0"=0.0, "Left Wing-B, C2/C0"=0.0, "Left Wing-C, C3/C0"=0.0, "Right Wing-A, C4/C0"=0.0, "Right Wing-B, C5/C0"=0.0, "Right Wing-C, C6/C0"=0.0} ("CDC data"), "Left Wing-A, C1/C0"=w1079, "Left Wing-B, C2/C0"=w1078, "Left Wing-C, C3/C0"=w1077, "Right Wing-A, C4/C0"=w1076, "Right Wing-B, C5/C0"=w1075, "Right Wing-C, C6/C0"=w1074) -> (w1081:T8)
                                n687 = local write "CDC data"(w1081) -> ()
                                }
                                frame #7 {
                                n688 = Index Array(array=w1104, index=4 ("인덱스")) -> (element=w1106:string)
                                n689 = Fract/Exp String To Number(string=w1106) -> (number=w1105:dbl)  [unwired: 3 in, 1 out]
                                n690 = Not Equal To 0?(x=w1105) -> (x != 0?=w1103:bool)
                                n691 = case shown="참" w1103 {
                                frame False {
                                }
                                frame True {
                                w1122 = i16 1 ("정밀도(6)")
                                n692 = local read "CDC data"() -> (w1133:T8)
                                n693 = Unbundle By Name(w1133) -> ("Left Wing-A, C1/C0"=w1117:dbl, "Left Wing-B, C2/C0"=w1118:dbl, "Left Wing-C, C3/C0"=w1119:dbl, "Right Wing-A, C4/C0"=w1115:dbl, "Right Wing-B, C5/C0"=w1114:dbl, "Right Wing-C, C6/C0"=w1113:dbl)
                                n694 = local read "Mark10 Gauge (lb)"() -> (w1112:dbl)
                                n695 = local read "FTS table index"() -> (w1108:i32)
                                n696 = Compound Arithmetic op=ADD(w1119, w1118, w1117) -> (w1120:dbl)
                                n697 = Compound Arithmetic op=ADD(w1115, w1114, w1113) -> (w1116:dbl)
                                n698 = Number To Fractional String(number=w1117, precision (6)=w1122) -> (F-format string=w1132:string)  [unwired: 2 in]
                                n699 = Number To Fractional String(number=w1118, precision (6)=w1122) -> (F-format string=w1131:string)  [unwired: 2 in]
                                n700 = Number To Fractional String(number=w1112, precision (6)=i16 2 ("정밀도(6)")) -> (F-format string=w1110:string)  [unwired: 2 in]
                                n701 = Number To Fractional String(number=w1119, precision (6)=w1122) -> (F-format string=w1130:string)  [unwired: 2 in]
                                n702 = Number To Fractional String(number=w1120, precision (6)=w1122) -> (F-format string=w1123:string)  [unwired: 2 in]
                                n703 = Number To Fractional String(number=w1115, precision (6)=w1122) -> (F-format string=w1129:string)  [unwired: 2 in]
                                n704 = Number To Fractional String(number=w1114, precision (6)=w1122) -> (F-format string=w1128:string)  [unwired: 2 in]
                                n705 = Number To Fractional String(number=w1113, precision (6)=w1122) -> (F-format string=w1127:string)  [unwired: 2 in]
                                n706 = Number To Fractional String(number=w1116, precision (6)=w1122) -> (F-format string=w1121:string)  [unwired: 2 in]
                                n707 = local read "Test Data table"() -> (w1124:string[][])
                                n708 = Increment(x=w1108) -> (x+1=w1109:i32)
                                n709 = Build Array(w1110, w1132, w1131, w1130, w1123, w1129, w1128, w1127, w1121) -> (w1126:string[])
                                n710 = local write "FTS table index"(w1109) -> ()
                                n711 = Replace Array Subset(array=w1124, new element=w1126, index (col)=w1108) -> (w1125:string[][])  [unwired: 1 in]
                                n712 = local write "Test Data table"(w1125) -> ()
                                }
                                }
                                }
                                frame #8 {
                                # "그래프 플롯 갯수 8개"
                                # "로드 그래프"
                                n713 = local read "FTS table index"() -> (w1136:i32)
                                n714 = local read "Test Data table"() -> (w1141:string[][])
                                n715 = Decrement(x=w1136) -> (x-1=w1135:i32)
                                n716 = Array Subset(array=w1141, index (col)=1 ("비활성화된 인덱스 (열)"), length (col)=w1135) -> (w1137:string[][])  [unwired: 2 in]
                                n717 = Fract/Exp String To Number(string=w1137) -> (number=w1140:dbl[][])  [unwired: 3 in, 1 out]
                                n718 = for {
                                N: 8 -> [_]
                                tunnel: [w1149] -> w1139 mode=indexing
                                tunnel: w1140 -> [w1148]
                                i -> [w1146]
                                # "Y"
                                # "X"
                                n719 = Add(x=1, y=w1146) -> (x+y=w1144:i32)
                                n720 = Index Array(array=w1148, index (row)=0 ("비활성화된 인덱스 (열)")) -> (element=w1143:dbl[])  [unwired: 1 in]
                                n721 = Index Array(array=w1148, index (row)=w1144) -> (element=w1142:dbl[])  [unwired: 1 in]
                                n722 = Bundle(w1143, w1142) -> (w1149:cluster{dbl[], dbl[]})  [unwired: 1 in]
                                }
                                "Load vs CDC Graph" <- w1139
                                }
                                frame #9 {
                                n723 = Index Array(array=w1151, index=5 ("인덱스")) -> (element=w1153:string)
                                n724 = Fract/Exp String To Number(string=w1153) -> (number=w1152:dbl)  [unwired: 3 in, 1 out]
                                n725 = Not Equal To 0?(x=w1152) -> (x != 0?=w1150:bool)
                                n726 = case shown="참" w1150 {
                                frame False {
                                }
                                frame True {
                                n727 = local read "Port-FTS"() -> (w1160:refnum<visa-resource-name>)
                                n728 = control-ref of="Test Status"() -> (w1156:refnum<vi>)
                                n729 = call "_시리얼_Mark10-제어 (압력설정).vi"("FTS 제어 상태"=T20 "헤더 상단 이동", "시리얼 포트"=w1160) -> ("게이지 압력(lb)"=w1158:dbl, "통신 정상"=w1161:bool)  [unwired: 1 in, 1 out]
                                n730 = local write "Mark10 Gauge (lb)"(w1158) -> ()
                                n731 = local write "FTS comm."(w1161) -> ()
                                n732 = call "SUB-Status string update.vi"("텍스트 입력"="Head Up" ("Force Test Status"), "날짜추가"=TRUE, "reference"=w1156) -> ()  [unwired: 2 in, 1 out]
                                }
                                }
                                }
                                }
                                }
                                }
                                frame #2 {
                                n733 = disable-structure shown="비활성화" {
                                frame Disabled {
                                n734 = local read "Port-FTS"() -> (w1164:refnum<visa-resource-name>)
                                n735 = call "_시리얼_Mark10-제어 (압력설정).vi"("FTS 제어 상태"=T20 "헤더 상단 이동", "시리얼 포트"=w1164) -> ("게이지 압력(lb)"=w1162:dbl, "통신 정상"=w1165:bool)  [unwired: 1 in, 1 out]
                                n736 = local write "Mark10 Gauge (lb)"(w1162) -> ()
                                n737 = local write "FTS comm."(w1165) -> ()
                                }
                                frame Enabled {
                                }
                                }
                                }
                                frame #3 {
                                n738 = control-ref of="Test Status"() -> (w1167:refnum<vi>)
                                n739 = local write "FTS OP status"(T6 "시험 후 점검" ("FTS 동작시험 상태")) -> ()
                                n740 = call "SUB-Status string update.vi"("텍스트 입력"="Done Force test by Profile\n" ("Force Test Status"), "날짜추가"=TRUE, "reference"=w1167) -> ()  [unwired: 2 in, 1 out]
                                }
                              }
                            }
                            frame "시험 후 점검" {
                              # "시험 종료 & \n측정 데이터 저장"
                              n741 = stacked-sequence {
                                seq-local: [_ w1192 _ _ _] -> [_ _ w1201 _ _]
                                seq-local: [w1180 _ _ _ _] -> [_ w1191 _ _ _]
                                seq-local: [w1174 _ _ _ _] -> [_ _ w1200 _ _]
                                frame #0 {
                                w1188 = T24 1 items=["사용자 홈"=0, "사용자 데스크탑"=1, "사용자 문서"=2, "사용자 어플리케이션 데이터"=3, "사용자 환경"=4, "사용자 임시"=5, "퍼블릭 문서"=6, "퍼블릭 어플리케이션 데이터"=7, "퍼블릭 환경"=8, "퍼블릭 캐시"=13, "시스템 코어 라이브러리"=9, "시스템 설치된 라이브러리"=10, "어플리케이션 파일"=11, "부팅 볼륨 루트"=12] ("system directory type")
                                n742 = call "SUB-module-현재 VI 경로.vi"() -> ("현재 VI 경로"=w1177:path)
                                n743 = call <vilib>:"Get System Directory.vi"("system directory type"=w1188) -> ("system directory"=w1187:path)  [unwired: 10 in]
                                n744 = Path To String(path=w1177) -> (string=w1176:string)
                                n745 = Path To String(path=w1187) -> (string=w1186:string)
                                n746 = Concatenate Strings(w1176, "\\Template" ("이름 또는 상대 경로"), "\\GEN4 FTS Test Report rev1.xlsx" ("이름 또는 상대 경로")) -> (w1175:string)
                                n747 = String To Path(string=w1175) -> (path=w1174:path)
                                n748 = Concatenate Strings(w1186, "\\GEN4-GUI Test data" ("상태")) -> (w1180:string)
                                n749 = String To Path(string=w1180) -> (path=w1184:path)
                                n750 = call <vilib>:"Check if File or Folder Exists.vi"("path"=w1184) -> ("error out"=w1181:errorcluster, "file or folder exists?"=w1183:bool, "dup path"=w1182:path)  [unwired: 8 in]
                                n751 = case shown="거짓" w1183 {
                                tunnel: w1182 -> [w1190 _]
                                tunnel: w1181 -> [w1189 _]
                                frame False {
                                n752 = Create Folder(path (use dialog)=w1190, error in=w1189) -> ()  [unwired: 1 in, 3 out]
                                }
                                frame True {
                                }
                                }
                                }
                                frame #1 {
                                # "* 파일명(rev)-date (trst name)"
                                # "파일 저장 경로"
                                n753 = local read "Test name"() -> (w1197:string)
                                n754 = Format Date/Time String(time format string (%c)="%Y%m%d %H%M%S" ("상태")) -> (date/time string=w1196:string)  [unwired: 2 in]
                                n755 = Format Into String(format string="\\\\GEN4 FTS (PP3A)-%s (%s).xlsx" ("상태"), w1196, w1197) -> (resulting string=w1193:string)  [unwired: 2 in, 1 out]
                                n756 = Concatenate Strings(w1191, w1193) -> (w1198:string)
                                n757 = String To Path(string=w1198) -> (path=w1192:path)
                                }
                                frame #2 {
                                n758 = local read "Cal/Test select"() -> (w1199:bool)
                                n759 = call <vilib>:"New Report.vi"("window state (normal)"=T17."normal", "report type"=T16."Excel", "template (empty)"=w1200) -> ("report out"=w1204:refnum<class "NI_report.lvclass">, "error out"=w1205:errorcluster)  [unwired: 11 in]
                                n760 = stacked-sequence {
                                tunnel: w1204 -> [w1209 w1234 w1236 w1261]
                                tunnel: w1205 -> [w1208 w1233 w1237 w1260]
                                tunnel: [w1209 _ _ _] -> w1207
                                tunnel: [w1208 _ _ _] -> w1206
                                tunnel: w1199 -> [_ _ _ w1259]
                                frame #0 {
                                }
                                frame #1 {
                                w1212 = 10 ("column")
                                w1219 = 2 ("row")
                                w1226 = 1 items=["top", "center", "bottom"] ("vertical alignment (top)")
                                # "Date"
                                # "박스의 좌측 상단 좌표"
                                n761 = Increment(x=w1212) -> (x+1=w1211:i32)
                                n762 = Increment(x=w1219) -> (x+1=w1214:i32)
                                n763 = Increment(x=w1211) -> (x+1=w1213:i32)
                                n764 = Bundle By Name(cluster=cluster{"row":i32, "column":i32} {"row"=3, "column"=10} ("start (-1, -1)"), "row"=w1214, "column"=w1213) -> (w1210:cluster{"row":i32, "column":i32})
                                n765 = Bundle By Name(cluster=cluster{"row":i32, "column":i32} {"row"=3, "column"=10} ("start (-1, -1)"), "row"=w1214, "column"=w1212) -> (w1220:cluster{"row":i32, "column":i32})
                                n766 = Format Date/Time String(time format string (%c)="%Y/%m/%d-%H:%M:%S" ("상태")) -> (date/time string=w1232:string)  [unwired: 2 in]
                                n767 = call <vilib>:"Excel Easy Text.vi"("report in"=w1234, "font"=T18 {"font name"="", "font size"=11.0, "bold"=1, "italic"=0, "underline"=0, "strike through"=0, "font color"=16777216}, "text"=w1232, "start (-1, -1)"=w1220, "end (-1, -1)"=w1210, "error in (no error)"=w1233) -> ("report out"=w1230:refnum<class "NI_report.lvclass">, "next cell bottom-left"=w1228:cluster{"row":i32, "column":i32}, "next cell top-right"=w1227:cluster{"row":i32, "column":i32}, "error out"=w1229:errorcluster)  [unwired: 5 in, 1 out]
                                n768 = Bundle By Name(cluster=cluster{"row":i32, "column":i32} {"row"=3, "column"=10} ("start (-1, -1)"), "row"=w1219, "column"=w1212) -> (w1218:cluster{"row":i32, "column":i32})
                                n769 = call <vilib>:"Excel Set Cell Alignment.vi"("report in"=w1230, "vertical alignment (top)"=w1226, "horizontal alignment (left)"=w1226, "start (-1, -1)"=w1228, "end (-1, -1)"=w1227, "error in (no error)"=w1229) -> ("report out"=w1225:refnum<class "NI_report.lvclass">, "error out"=w1224:errorcluster)  [unwired: 8 in]
                                n770 = call <vilib>:"Excel Set Cell Color and Border.vi"("report in"=w1225, "outside border"=T19 {"on/off"=TRUE, "weight"=2, "color"=0}, "background color (w)"=u32 16777215, "start (-1, -1)"=w1218, "end (-1, -1)"=w1210, "error in (no error)"=w1224) -> ()  [unwired: 8 in, 2 out]
                                }
                                frame #2 {
                                w1240 = 4 ("column")
                                w1247 = 4 ("row")
                                w1254 = 1 items=["top", "center", "bottom"] ("vertical alignment (top)")
                                # "Device No."
                                # "박스의 좌측 상단 좌표"
                                n771 = local read "Test name"() -> (w1235:string)
                                n772 = Increment(x=w1240) -> (x+1=w1239:i32)
                                n773 = Increment(x=w1247) -> (x+1=w1242:i32)
                                n774 = Increment(x=w1239) -> (x+1=w1241:i32)
                                n775 = Bundle By Name(cluster=cluster{"row":i32, "column":i32} {"row"=3, "column"=10} ("start (-1, -1)"), "row"=w1242, "column"=w1241) -> (w1238:cluster{"row":i32, "column":i32})
                                n776 = Bundle By Name(cluster=cluster{"row":i32, "column":i32} {"row"=3, "column"=10} ("start (-1, -1)"), "row"=w1242, "column"=w1240) -> (w1248:cluster{"row":i32, "column":i32})
                                n777 = call <vilib>:"Excel Easy Text.vi"("report in"=w1236, "font"=T18 {"font name"="", "font size"=11.0, "bold"=1, "italic"=0, "underline"=0, "strike through"=0, "font color"=16777216}, "text"=w1235, "start (-1, -1)"=w1248, "end (-1, -1)"=w1238, "error in (no error)"=w1237) -> ("report out"=w1258:refnum<class "NI_report.lvclass">, "next cell bottom-left"=w1256:cluster{"row":i32, "column":i32}, "next cell top-right"=w1255:cluster{"row":i32, "column":i32}, "error out"=w1257:errorcluster)  [unwired: 5 in, 1 out]
                                n778 = Bundle By Name(cluster=cluster{"row":i32, "column":i32} {"row"=3, "column"=10} ("start (-1, -1)"), "row"=w1247, "column"=w1240) -> (w1246:cluster{"row":i32, "column":i32})
                                n779 = call <vilib>:"Excel Set Cell Alignment.vi"("report in"=w1258, "vertical alignment (top)"=w1254, "horizontal alignment (left)"=w1254, "start (-1, -1)"=w1256, "end (-1, -1)"=w1255, "error in (no error)"=w1257) -> ("report out"=w1253:refnum<class "NI_report.lvclass">, "error out"=w1252:errorcluster)  [unwired: 8 in]
                                n780 = call <vilib>:"Excel Set Cell Color and Border.vi"("report in"=w1253, "outside border"=T19 {"on/off"=TRUE, "weight"=2, "color"=0}, "background color (w)"=u32 16777215, "start (-1, -1)"=w1246, "end (-1, -1)"=w1238, "error in (no error)"=w1252) -> ()  [unwired: 8 in, 2 out]
                                }
                                frame #3 {
                                n781 = case shown="거짓" w1259 {
                                tunnel: w1261 -> [w1263 w1298]
                                tunnel: w1260 -> [w1262 w1297]
                                frame False {
                                # "Test-mode"
                                n782 = stacked-sequence {
                                tunnel: w1263 -> [w1275 w1294]
                                tunnel: w1262 -> [w1274 w1293]
                                frame #0 {
                                # "Load(lb)"
                                n783 = local read "Test Data table"() -> (w1273:string[][])
                                n784 = Index Array(array=w1273, index (row)=0 ("인덱스 (행)")) -> (element=w1270:string[])  [unwired: 1 in]
                                n785 = Replace Array Subset(array=w1270, new element="Offset" ("새 원소/부분배열"), index=0 ("인덱스")) -> (w1267:string[])
                                n786 = Build Array(w1267) -> (w1266:string[][])
                                n787 = Transpose 2D Array(2D array=w1266) -> (transposed array=w1265:string[][])
                                n788 = call-poly <vilib>:"Excel Easy Table.vi"("report in"=w1275, "font"=T18 {"font name"="", "font size"=11.0, "bold"=0, "italic"=0, "underline"=0, "strike through"=0, "font color"=16777216}, "start (0, 0)"=cluster{"row":i32, "column":i32} {"row"=24, "column"=1}, "text data"=w1265, "error in (no error)"=w1274) -> ()  [unwired: 6 in, 5 out]
                                }
                                frame #1 {
                                # "Load(lb)"
                                n789 = local read "Test Data table"() -> (w1287:string[][])
                                n790 = Index Array(array=w1287, index (row) #1=1 ("인덱스 (행)"), index (row) #2=2 ("인덱스 (행)"), index (row) #3=3 ("인덱스 (행)")) -> (element #1=w1286:string[], element #2=w1285:string[], element #3=w1284:string[])  [unwired: 3 in]
                                n791 = Index Array(array=w1287, index (row) #1=5 ("인덱스 (행)"), index (row) #2=6 ("인덱스 (행)"), index (row) #3=7 ("인덱스 (행)")) -> (element #1=w1283:string[], element #2=w1282:string[], element #3=w1281:string[])  [unwired: 3 in]
                                n792 = Build Array(w1283, w1282, w1281) -> (w1279:string[][])
                                n793 = Build Array(w1286, w1285, w1284) -> (w1280:string[][])
                                n794 = Build Array (concatenate)(w1280, w1279) -> (w1278:string[][])
                                n795 = Transpose 2D Array(2D array=w1278) -> (transposed array=w1277:string[][])
                                n796 = call-poly <vilib>:"Excel Easy Table.vi"("report in"=w1294, "font"=T18 {"font name"="", "font size"=11.0, "bold"=0, "italic"=0, "underline"=0, "strike through"=0, "font color"=16777216}, "start (0, 0)"=cluster{"row":i32, "column":i32} {"row"=24, "column"=3}, "text data"=w1277, "error in (no error)"=w1293) -> ()  [unwired: 6 in, 5 out]
                                }
                                }
                                }
                                frame True {
                                # "Cal-mode"
                                n797 = stacked-sequence {
                                tunnel: w1298 -> [w1310 w1329]
                                tunnel: w1297 -> [w1309 w1328]
                                frame #0 {
                                # "Load(lb)"
                                n798 = local read "Test Data table"() -> (w1308:string[][])
                                n799 = Index Array(array=w1308, index (row)=0 ("인덱스 (행)")) -> (element=w1305:string[])  [unwired: 1 in]
                                n800 = Replace Array Subset(array=w1305, new element="Offset" ("새 원소/부분배열"), index=0 ("인덱스")) -> (w1302:string[])
                                n801 = Build Array(w1302) -> (w1301:string[][])
                                n802 = Transpose 2D Array(2D array=w1301) -> (transposed array=w1300:string[][])
                                n803 = call-poly <vilib>:"Excel Easy Table.vi"("report in"=w1310, "font"=T18 {"font name"="", "font size"=11.0, "bold"=0, "italic"=0, "underline"=0, "strike through"=0, "font color"=16777216}, "start (0, 0)"=cluster{"row":i32, "column":i32} {"row"=14, "column"=1}, "text data"=w1300, "error in (no error)"=w1309) -> ()  [unwired: 6 in, 5 out]
                                }
                                frame #1 {
                                # "Load(lb)"
                                n804 = local read "Test Data table"() -> (w1322:string[][])
                                n805 = Index Array(array=w1322, index (row) #1=1 ("인덱스 (행)"), index (row) #2=2 ("인덱스 (행)"), index (row) #3=3 ("인덱스 (행)")) -> (element #1=w1321:string[], element #2=w1320:string[], element #3=w1319:string[])  [unwired: 3 in]
                                n806 = Index Array(array=w1322, index (row) #1=5 ("인덱스 (행)"), index (row) #2=6 ("인덱스 (행)"), index (row) #3=7 ("인덱스 (행)")) -> (element #1=w1318:string[], element #2=w1317:string[], element #3=w1316:string[])  [unwired: 3 in]
                                n807 = Build Array(w1318, w1317, w1316) -> (w1314:string[][])
                                n808 = Build Array(w1321, w1320, w1319) -> (w1315:string[][])
                                n809 = Build Array (concatenate)(w1315, w1314) -> (w1313:string[][])
                                n810 = Transpose 2D Array(2D array=w1313) -> (transposed array=w1312:string[][])
                                n811 = call-poly <vilib>:"Excel Easy Table.vi"("report in"=w1329, "font"=T18 {"font name"="", "font size"=11.0, "bold"=0, "italic"=0, "underline"=0, "strike through"=0, "font color"=16777216}, "start (0, 0)"=cluster{"row":i32, "column":i32} {"row"=14, "column"=3}, "text data"=w1312, "error in (no error)"=w1328) -> ()  [unwired: 6 in, 5 out]
                                }
                                }
                                }
                                }
                                }
                                }
                                n812 = call-dynamic "Save Report to File.vi"("report in"=w1207, "report file path"=w1201, "error in (no error)"=w1206) -> ()  [unwired: 11 in, 2 out]
                                }
                                frame #3 {
                                }
                                frame #4 {
                                }
                              }
                              n813 = control-ref of="Test Status"() -> (w1172:refnum<vi>)
                              n814 = call "SUB-Status string update.vi"("텍스트 입력"="Result Data Process\n" ("Force Test Status"), "날짜추가"=TRUE, "reference"=w1172) -> ()  [unwired: 2 in, 1 out]
                              n815 = local write "FTS OP status"(T6 "시험 종료" ("FTS 동작시험 상태")) -> ()
                            }
                            frame "시험 종료", Default {
                              # "BLE 버퍼 클리어"
                              # "시험 종료"
                              n816 = control-ref of="Test Status"() -> (w1335:refnum<vi>)
                              n817 = local write "Mark10 Gauge (lb)"(0.0 ("Mark10 Gauge")) -> ()
                              n818 = local write "Clear graph 1"(TRUE ("그래프 지우기")) -> ()
                              n819 = call "SUB-Status string update.vi"("텍스트 입력"="Test complete." ("Force Test Status"), "날짜추가"=TRUE, "reference"=w1335) -> ()  [unwired: 2 in, 1 out]
                              n820 = call <vilib>:"Beep.vi"() -> ()  [unwired: 12 in]
                              n821 = call "SUB-BLE Rx data Clear.vi"() -> ()  [unwired: 6 in]
                            }
                          }
                        }
                      }
                      frame #4 {
                        n822 = local write "Test Start"(FALSE ("Test Start")) -> ()
                        n823 = local write "FTS comm."(FALSE ("FTS 수신 정상")) -> ()
                        n824 = local write "FTS Testing"(FALSE ("FTS 시험 진행")) -> ()
                      }
                    }
                  }
                }
              }
            }
          }
          frame #5 {
            # "설정값 읽기"
            n825 = call "SUB-BLE Rx data (Set)-Classify.vi"() -> ("data out"=w1341:u8[], "Rx-data"=w1342:bool)  [unwired: 4 in]
            n826 = case shown="참" w1342 {
              tunnel: w1341 -> [_ w1345]
              frame False {
              }
              frame True {
                n827 = flat-sequence {
                  tunnel: w1345 -> [w1347]
                  tunnel: [w1347] -> w1343
                  tunnel: [w1349] -> w1344
                  tunnel: w1343 -> [w1349]
                  tunnel: w1344 -> [w1351]
                  frame #0 {
                    n828 = local write "Data_mon(h)"("" ("Data_mon")) -> ()
                  }
                  frame #1 {
                    n829 = Wait (ms)(milliseconds to wait=u32 20 ("대기 시간(ms)")) -> ()  [unwired: 1 out]
                  }
                  frame #2 {
                    n830 = Byte Array To String(unsigned byte array=w1351) -> (string=→"Data_mon(h)":string)
                    n831 = local read "Data Log"() -> (w1350:string)
                    n832 = call <vilib>:"Space Constant.vi"() -> ("String"=w1356:string)
                    n833 = Format Date/Time String(time format string (%c)="%H:%M:%S%3u>  " ("상태")) -> (date/time string=w1355:string)  [unwired: 2 in]
                    n834 = Array To Spreadsheet String(delimiter (Tab)=w1356, array=w1351, 3:"%02X" ("포맷 문자열")) -> (spreadsheet string=w1353:string)
                    n835 = Concatenate Strings(w1355, w1353, w1350) -> (w1352:string)
                    n836 = local write "Data Log"(w1352) -> ()
                  }
                }
              }
            }
          }
          frame #6 {
            # "설정값 저장"
            n837 = local read "Comm con status 1"() -> (w1359:bool)
            n838 = case shown="참" w1359 {
              frame False {
              }
              frame True {
              }
            }
          }
          frame #7 {
            # "지연 시간, 상태값 리셋"
            n839 = local read "Comm con status 1"() -> (w1365:bool)
            n840 = local read "Clear graph 1"() -> (w1364:bool)
            n841 = Not(x=w1365) -> (.not. x?=w1362:bool)
            n842 = case shown="참" w1362 {
              frame False {
              }
              frame True {
                n843 = local write "status string"("Ready (available after the communication connection)" ("status string")) -> ()
              }
            }
            n844 = case shown="참" w1364 {
              frame False {
              }
              frame True {
                # "BLE 버퍼 클리어"
                n845 = local write "Clear graph 1"(FALSE ("그래프 지우기")) -> ()
                n846 = call "SUB-BLE Rx data Clear.vi"() -> ()  [unwired: 6 in]
                n847 = property on="CDC(PCAP02) Graph" class="WFChart (엄격한)"("History Data"=waveform(dbl)[][] [] ("히스토리 데이터")) -> ()  [unwired: 2 in, 2 out]
              }
            }
            n848 = local read "Export graph 1"() -> (w1363:bool)
            n849 = local read "Export graph2"() -> (w1361:bool)
            n850 = local read "Clear graph 2"() -> (w1360:bool)
            n851 = case shown="참" w1361 {
              frame False {
              }
              frame True {
                n852 = invoke on="IMU Graph" class="WFChart (엄격한)" method="Export Data to Excel"() -> ()  [unwired: 3 in, 3 out]
                n853 = local write "Export graph2"(FALSE ("그래프 반출")) -> ()
              }
            }
            n854 = case shown="참" w1363 {
              frame False {
              }
              frame True {
                n855 = invoke on="CDC(PCAP02) Graph" class="WFChart (엄격한)" method="Export Data to Excel"() -> ()  [unwired: 3 in, 3 out]
                n856 = local write "Export graph 1"(FALSE ("그래프 반출")) -> ()
              }
            }
            n857 = case shown="참" w1360 {
              frame False {
              }
              frame True {
                # "BLE 버퍼 클리어"
                n858 = local write "Clear graph 2"(FALSE ("그래프 지우기")) -> ()
                n859 = call "SUB-BLE Rx data Clear.vi"() -> ()  [unwired: 6 in]
                n860 = property on="IMU Graph" class="WFChart (엄격한)"("History Data"=waveform(dbl)[][] [] ("히스토리 데이터")) -> ()  [unwired: 2 in, 2 out]
              }
            }
          }
          frame #8 {
            # "옵셋 설정 (저장)"
            n861 = local read "Comm con status 1"() -> (w1375:bool)
            n862 = local read "Comm con status 1"() -> (w1376:bool)
            n863 = local read "Offset 2"() -> (w1374:bool)
            n864 = local read "Offset 1"() -> (w1377:bool)
            n865 = And(x=w1375, y=w1374) -> (x .and. y?=w1373:bool)
            n866 = And(x=w1376, y=w1377) -> (x .and. y?=w1378:bool)
            n867 = case shown="참" w1373 {
              frame False {
                n868 = local write "Offset 2"(FALSE ("Offset 1")) -> ()
              }
              frame True {
                n869 = local write "Offset 2"(FALSE ("Offset 1")) -> ()
                n870 = local write "Clear graph 2"(TRUE ("그래프 지우기")) -> ()
                n871 = for {
                  N: 50 -> [_]
                  tunnel: [w1449] -> w1427 mode=indexing
                  tunnel: [w1448] -> w1428 mode=indexing
                  tunnel: [w1447] -> w1429 mode=indexing
                  tunnel: [w1446] -> w1430 mode=indexing
                  tunnel: [w1445] -> w1431 mode=indexing
                  tunnel: [w1444] -> w1432 mode=indexing
                  n872 = local read "IMU Offet"() -> (w1443:T9)
                  n873 = call "SUB-BLE Rx data (Mon)-Wait.vi"("Timeout(ms)"=u16 200) -> ("RxReady"=w1450:bool)  [unwired: 4 in]
                  n874 = case shown="참" w1450 {
                    tunnel: [w1453 w1455] -> w1442
                    tunnel: w1443 -> [w1453 _]
                    frame False {
                    }
                    frame True {
                      n875 = call "SUB-BLE Rx data (Mon)-Classify.vi"() -> ("data out"=w1456:u8[], "Rx-mon"=w1454:bool)  [unwired: 5 in, 3 out]
                      n876 = case shown="참" w1454 {
                        tunnel: w1456 -> [_ w1458]
                        tunnel: [_ w1457] -> w1455
                        frame False {
                        }
                        frame True {
                          n877 = call "SUB-BLE Rx data (Mon)-CDC IMU.vi"("data in"=w1458) -> ("IMU data"=w1457:T9)  [unwired: 4 in, 3 out]
                        }
                      }
                    }
                  }
                  n878 = Unbundle By Name(w1442) -> ("Gyroscope X"=w1449:dbl, "Gyroscope Y"=w1448:dbl, "Gyroscope Z"=w1447:dbl, "Accelerometer X"=w1446:dbl, "Accelerometer Y"=w1445:dbl, "Accelerometer Z"=w1444:dbl)
                  n879 = Wait Until Next ms Multiple(millisecond multiple=u32 20 ("ms 배수")) -> ()  [unwired: 1 out]
                }
                n880 = call-poly <vilib>:"Mean.vi"("X"=w1427) -> ("mean"=w1434:dbl)  [unwired: 1 out]
                n881 = call-poly <vilib>:"Mean.vi"("X"=w1428) -> ("mean"=w1435:dbl)  [unwired: 1 out]
                n882 = call-poly <vilib>:"Mean.vi"("X"=w1429) -> ("mean"=w1436:dbl)  [unwired: 1 out]
                n883 = call-poly <vilib>:"Mean.vi"("X"=w1430) -> ("mean"=w1437:dbl)  [unwired: 1 out]
                n884 = call-poly <vilib>:"Mean.vi"("X"=w1431) -> ("mean"=w1438:dbl)  [unwired: 1 out]
                n885 = call-poly <vilib>:"Mean.vi"("X"=w1432) -> ("mean"=w1439:dbl)  [unwired: 1 out]
                n886 = Bundle By Name(cluster=T9 {"Gyroscope X"=0.0, "Gyroscope Y"=0.0, "Gyroscope Z"=0.0, "Accelerometer X"=0.0, "Accelerometer Y"=0.0, "Accelerometer Z"=0.0} ("IMU data"), "Gyroscope X"=w1434, "Gyroscope Y"=w1435, "Gyroscope Z"=w1436, "Accelerometer X"=w1437, "Accelerometer Y"=w1438, "Accelerometer Z"=w1439) -> (w1433:T9)
                n887 = local write "IMU Offet"(w1433) -> ()
              }
            }
            n888 = case shown="참" w1378 {
              frame False {
                n889 = local write "Offset 1"(FALSE ("Offset 1")) -> ()
              }
              frame True {
                n890 = local write "Offset 1"(FALSE ("Offset 1")) -> ()
                n891 = local write "Clear graph 1"(TRUE ("그래프 지우기")) -> ()
                n892 = local read "Offset Souce"() -> (w1382:enum32{"Normal", "Raw"})
                n893 = Equal?(x=w1382, y=enum32{"Normal", "Raw"}."Normal" ("Offset Souce")) -> (x = y?=w1380:bool)
                n894 = for {
                  N: 50 -> [_]
                  tunnel: [w1408] -> w1396 mode=indexing
                  tunnel: [w1407] -> w1395 mode=indexing
                  tunnel: [w1406] -> w1394 mode=indexing
                  tunnel: [w1405] -> w1393 mode=indexing
                  tunnel: [w1404] -> w1392 mode=indexing
                  tunnel: [w1403] -> w1391 mode=indexing
                  tunnel: w1380 -> [w1400]
                  n895 = local read "CDC Offet"() -> (w1401:T8)
                  n896 = call "SUB-BLE Rx data (Mon)-Wait.vi"("Timeout(ms)"=u16 200) -> ("RxReady"=w1409:bool)  [unwired: 4 in]
                  n897 = case shown="참" w1409 {
                    tunnel: [w1412 w1415] -> w1402
                    tunnel: w1401 -> [w1412 _]
                    tunnel: w1400 -> [_ w1413]
                    frame False {
                    }
                    frame True {
                      n898 = call "SUB-BLE Rx data (Mon)-Classify.vi"() -> ("data out"=w1416:u8[], "Rx-mon"=w1414:bool)  [unwired: 5 in, 3 out]
                      n899 = case shown="거짓" w1414 {
                        tunnel: w1416 -> [w1421 w1423]
                        tunnel: [w1420 w1422] -> w1415
                        tunnel: w1413 -> [w1419 _]
                        frame False {
                          n900 = call "SUB-BLE Rx data (Debug)-CDC.vi"("data in"=w1421) -> ("CDC debug"=w1417:T8, "CDC mon"=w1418:T8)  [unwired: 6 in]
                          n901 = Select(t=w1418, s=w1419, f=w1417) -> (s? t:f=w1420:T8)
                        }
                        frame True {
                          n902 = call "SUB-BLE Rx data (Mon)-CDC IMU.vi"("data in"=w1423) -> ("CDC data"=w1422:T8)  [unwired: 4 in, 3 out]
                        }
                      }
                    }
                  }
                  n903 = Unbundle By Name(w1402) -> ("Left Wing-A, C1/C0"=w1408:dbl, "Left Wing-B, C2/C0"=w1407:dbl, "Left Wing-C, C3/C0"=w1406:dbl, "Right Wing-A, C4/C0"=w1405:dbl, "Right Wing-B, C5/C0"=w1404:dbl, "Right Wing-C, C6/C0"=w1403:dbl)
                  n904 = Wait Until Next ms Multiple(millisecond multiple=u32 20 ("ms 배수")) -> ()  [unwired: 1 out]
                }
                n905 = call-poly <vilib>:"Mean.vi"("X"=w1396) -> ("mean"=w1388:dbl)  [unwired: 1 out]
                n906 = call-poly <vilib>:"Mean.vi"("X"=w1395) -> ("mean"=w1387:dbl)  [unwired: 1 out]
                n907 = call-poly <vilib>:"Mean.vi"("X"=w1394) -> ("mean"=w1386:dbl)  [unwired: 1 out]
                n908 = call-poly <vilib>:"Mean.vi"("X"=w1393) -> ("mean"=w1385:dbl)  [unwired: 1 out]
                n909 = call-poly <vilib>:"Mean.vi"("X"=w1392) -> ("mean"=w1384:dbl)  [unwired: 1 out]
                n910 = call-poly <vilib>:"Mean.vi"("X"=w1391) -> ("mean"=w1383:dbl)  [unwired: 1 out]
                n911 = Bundle By Name(cluster=T8 {"Left Wing-A, C1/C0"=0.0, "Left Wing-B, C2/C0"=0.0, "Left Wing-C, C3/C0"=0.0, "Right Wing-A, C4/C0"=0.0, "Right Wing-B, C5/C0"=0.0, "Right Wing-C, C6/C0"=0.0} ("CDC data"), "Left Wing-A, C1/C0"=w1388, "Left Wing-B, C2/C0"=w1387, "Left Wing-C, C3/C0"=w1386, "Right Wing-A, C4/C0"=w1385, "Right Wing-B, C5/C0"=w1384, "Right Wing-C, C6/C0"=w1383) -> (w1389:T8)
                n912 = local write "CDC Offet"(w1389) -> ()
              }
            }
          }
          frame #9 {
            # "데이터 로깅-GUI data"
            n913 = disable-structure shown="활성화" {
              frame Disabled {
                n914 = local read "Data Logging"() -> (w1459:bool)
                n915 = case shown="참" w1459 {
                  frame False {
                    n916 = local read "Logging No."() -> (w1461:u32)
                    n917 = Not Equal To 0?(x=w1461) -> (x != 0?=w1460:bool)
                    n918 = case shown="참" w1460 {
                      frame False {
                      }
                      frame True {
                        n919 = local read "log refnum"() -> (w1463:refnum<file>)
                        n920 = local write "Logging No."(u32 0 ("Logging No.")) -> ()
                        n921 = Close File(refnum=w1463) -> ()  [unwired: 1 in, 2 out]
                      }
                    }
                  }
                  frame True {
                    n922 = stacked-sequence {
                      seq-local: [w1464 _] -> [_ w1516]
                      frame #0 {
                        n923 = local read "IMU data"() -> (w1467:T9)
                        n924 = local read "CDC data"() -> (w1484:T8)
                        n925 = Unbundle By Name(w1484) -> ("Left Wing-A, C1/C0"=w1481:dbl, "Left Wing-B, C2/C0"=w1480:dbl, "Left Wing-C, C3/C0"=w1479:dbl, "Right Wing-A, C4/C0"=w1478:dbl, "Right Wing-B, C5/C0"=w1477:dbl, "Right Wing-C, C6/C0"=w1476:dbl)
                        n926 = Unbundle By Name(w1467) -> ("Gyroscope X"=w1470:dbl, "Gyroscope Y"=w1471:dbl, "Gyroscope Z"=w1472:dbl, "Accelerometer X"=w1473:dbl, "Accelerometer Y"=w1474:dbl, "Accelerometer Z"=w1475:dbl)
                        n927 = Format Into String(format string="%.7f,%.7f,%.7f,%.7f,%.7f,%.7f," ("포맷 문자열"), initial string=",,(GUI) CDC Data," ("포맷 문자열"), w1481, w1480, w1479, w1478, w1477, w1476) -> (resulting string=w1466:string)  [unwired: 1 in, 1 out]
                        n928 = Format Into String(format string="%.6f,%.6f,%.6f,%.6f,%.6f,%.6f," ("포맷 문자열"), initial string=",(GUI) IMU Data," ("포맷 문자열"), w1470, w1471, w1472, w1473, w1474, w1475) -> (resulting string=w1465:string)  [unwired: 1 in, 1 out]
                        n929 = Concatenate Strings(w1466, w1465) -> (w1464:string)
                      }
                      frame #1 {
                        w1510 = T24 1 items=["사용자 홈"=0, "사용자 데스크탑"=1, "사용자 문서"=2, "사용자 어플리케이션 데이터"=3, "사용자 환경"=4, "사용자 임시"=5, "퍼블릭 문서"=6, "퍼블릭 어플리케이션 데이터"=7, "퍼블릭 환경"=8, "퍼블릭 캐시"=13, "시스템 코어 라이브러리"=9, "시스템 설치된 라이브러리"=10, "어플리케이션 파일"=11, "부팅 볼륨 루트"=12] ("system directory type")
                        # "첫행(타이틀)"
                        n930 = local read "Log no"() -> (w1485:string)
                        n931 = local read "Logging No."() -> (w1499:u32)
                        n932 = Format Date/Time String(time format string (%c)="Data Logging Start...  %Y/%m/%d %H:%M:%S" ("상태")) -> (date/time string=w1490:string)  [unwired: 2 in]
                        n933 = Format Into String(format string="\\\\GEN4 Data Logging(%s).csv" ("문자열"), w1485) -> (resulting string=w1486:string)  [unwired: 2 in, 1 out]
                        n934 = local read "RxD"() -> (w1520:string)
                        n935 = call <vilib>:"Get System Directory.vi"("system directory type"=w1510) -> ("system directory"=w1509:path)  [unwired: 10 in]
                        n936 = Format Into String(format string="\\r\\n\\r\\n%s\\r\\n%s\\r\\n" ("포맷 문자열"), w1490, "No.,Time,,Type,F/W ver.,(Raw)Left Wing-A,(Raw)Left Wing-B,(Raw)Left Wing-C,(Raw)Right Wing-A,(Raw)Right Wing-B,(Raw)Right Wing-C,(Raw)CDC Status,(Raw)Gyroscope X,(Raw)Gyroscope Y,(Raw)Gyroscope Z,(Raw)Accelerometer X,(Raw)Accelerometer Y,(Raw)Accelerometer Z,,Type,(GUI)Left Wing-A,(GUI)Left Wing-B,(GUI)Left Wing-C,(GUI)Right Wing-A,(GUI)Right Wing-B,(GUI)Right Wing-C,,Type,(GUI)Gyroscope X,(GUI)Gyroscope Y,(GUI)Gyroscope Z,(GUI)Accelerometer X,(GUI)Accelerometer Y,(GUI)Accelerometer Z" ("문자열")) -> (resulting string=w1488:string)  [unwired: 2 in, 1 out]
                        n937 = Increment(x=w1499) -> (x+1=w1515:u32)
                        n938 = Path To String(path=w1509) -> (string=w1508:string)
                        n939 = Equal To 0?(x=w1499) -> (x = 0?=w1497:bool)
                        n940 = Format Date/Time String(time format string (%c)="%Y/%m/%d %H:%M:%S%3u,,RXD Raw Data," ("상태")) -> (date/time string=w1522:string)  [unwired: 2 in]
                        n941 = Match Pattern(string=w1520, regular expression="#:" ("검색 문자열")) -> (after substring=w1518:string)  [unwired: 1 in, 3 out]
                        n942 = Format Into String(format string="%d," ("포맷 문자열"), w1499) -> (resulting string=w1513:string)  [unwired: 2 in, 1 out]
                        n943 = Concatenate Strings(w1508, w1486) -> (w1507:string)
                        n944 = local write "Logging No."(w1515) -> ()
                        n945 = String To Path(string=w1507) -> (path=w1506:path)
                        n946 = Open/Create/Replace File(file path (use dialog)=w1506, operation (0:open)=T22."open or create" ("동작(0:open)"), access (0:read/write)=enum16{"read/write", "read-only", "write-only"}."read/write" ("접근(0:읽기/쓰기)")) -> (refnum out=w1501:refnum<file>, error out=w1500:errorcluster)  [unwired: 3 in, 1 out]
                        n947 = Select(t=w1488, s=w1497, f="") -> (s? t:f=w1496:string)
                        n948 = Concatenate Strings(w1513, w1522, w1518, w1516, "\r\n") -> (w1495:string)
                        n949 = Get File Position(4:w1500, 7:w1501) -> (0:w1511:errorcluster, 2:w1498:i64, 3:w1512:refnum<file>)
                        n950 = Concatenate Strings(w1496, w1495) -> (w1494:string)
                        n951 = call <vilib>:"Write File+ (string).vi"("string"=w1494, "error in (no error)"=w1511, "pos offset (bytes:0)"=w1498, "refnum"=w1512) -> ("error out"=w1502:errorcluster, "dup refnum"=w1503:refnum<file>)  [unwired: 3 in, 1 out]
                        "log refnum" <- w1503
                        n952 = disable-structure shown="비활성화" {
                          disable-tunnel: w1503 -> [w1524 _]
                          disable-tunnel: w1502 -> [w1523 _]
                          frame Disabled {
                            n953 = Close File(refnum=w1524, error in=w1523) -> ()  [unwired: 2 out]
                          }
                          frame Enabled {
                          }
                        }
                      }
                    }
                  }
                }
              }
              frame Enabled {
              }
            }
          }
          frame #10 {
            # "데이터 로깅-BLE data"
            n954 = local read "Timer-ble log"() -> (w1531:u32)
            n955 = Tick Count (ms)() -> (millisecond timer value=w1532:u32)
            n956 = local read "log data1"() -> (w1529:bool)
            n957 = local read "Data Logging"() -> (w1530:bool)
            n958 = Subtract(x=w1532, y=w1531) -> (x-y=w1528:u32)
            n959 = Greater Or Equal?(x=w1528, y=u32 3000) -> (x >= y?=w1526:bool)
            n960 = Compound Arithmetic op=AND ("복합 연산")(w1530, w1529, w1526) -> (w1525:bool)
            n961 = case shown="참" w1525 {
              frame False {
              }
              frame True {
                n962 = stacked-sequence {
                  seq-local: [w1533 _ _] -> [_ _ w1538]
                  frame #0 {
                    n963 = local read "log ble buf"() -> (w1533:string)
                  }
                  frame #1 {
                    n964 = Tick Count (ms)() -> (millisecond timer value=w1536:u32)
                    n965 = local write "Timer-ble log"(w1536) -> ()
                    n966 = local write "log data1"(FALSE ("log data1")) -> ()
                    n967 = local write "log ble buf"("" ("log ble buf")) -> ()
                  }
                  frame #2 {
                    n968 = String Length(string=w1538) -> (length=w1537:i32)
                    n969 = case shown="1.." w1537 {
                      tunnel: w1538 -> [_ w1539]
                      frame 0, Default {
                      }
                      frame 1.. {
                        w1554 = T24 1 items=["사용자 홈"=0, "사용자 데스크탑"=1, "사용자 문서"=2, "사용자 어플리케이션 데이터"=3, "사용자 환경"=4, "사용자 임시"=5, "퍼블릭 문서"=6, "퍼블릭 어플리케이션 데이터"=7, "퍼블릭 환경"=8, "퍼블릭 캐시"=13, "시스템 코어 라이브러리"=9, "시스템 설치된 라이브러리"=10, "어플리케이션 파일"=11, "부팅 볼륨 루트"=12] ("system directory type")
                        n970 = local read "Log no"() -> (w1540:string)
                        n971 = Format Into String(format string="\\\\GEN4 BLE Data Logging(%s).txt" ("문자열"), w1540) -> (resulting string=w1541:string)  [unwired: 2 in, 1 out]
                        n972 = call <vilib>:"Get System Directory.vi"("system directory type"=w1554) -> ("system directory"=w1553:path)  [unwired: 10 in]
                        n973 = Path To String(path=w1553) -> (string=w1552:string)
                        n974 = Concatenate Strings(w1552, w1541) -> (w1551:string)
                        n975 = String To Path(string=w1551) -> (path=w1550:path)
                        n976 = Open/Create/Replace File(file path (use dialog)=w1550, operation (0:open)=T22."open or create" ("동작(0:open)"), access (0:read/write)=enum16{"read/write", "read-only", "write-only"}."read/write" ("접근(0:읽기/쓰기)")) -> (refnum out=w1545:refnum<file>, error out=w1544:errorcluster)  [unwired: 3 in, 1 out]
                        n977 = Get File Position(4:w1544, 7:w1545) -> (0:w1555:errorcluster, 2:w1543:i64, 3:w1556:refnum<file>)
                        n978 = call <vilib>:"Write File+ (string).vi"("string"=w1539, "error in (no error)"=w1555, "pos offset (bytes:0)"=w1543, "refnum"=w1556) -> ("error out"=w1546:errorcluster, "dup refnum"=w1547:refnum<file>)  [unwired: 3 in, 1 out]
                        n979 = disable-structure shown="비활성화" {
                          disable-tunnel: w1547 -> [w1558 _]
                          disable-tunnel: w1546 -> [w1557 _]
                          frame Disabled {
                            n980 = Close File(refnum=w1558, error in=w1557) -> ()  [unwired: 2 out]
                          }
                          frame Enabled {
                          }
                        }
                      }
                    }
                  }
                }
              }
            }
          }
          frame #11 {
            n981 = local write "Rx-debug"(FALSE ("Rx-debug")) -> ()
            n982 = local write "Rx-mon"(FALSE) -> ()
          }
          frame #12 {
            # "디버깅 위해 창의 우측 크게 조정"
            # "창크게"
            n983 = local read "창크게"() -> (w1561:bool)
            n984 = case shown="참" w1561 {
              frame False {
              }
              frame True {
                n985 = First Call?() -> (First Call?: T/F=w1563:bool)
                n986 = case shown="참" w1563 {
                  frame False {
                  }
                  frame True {
                    w1580 = 250  # 확장 창 크기
                    n987 = Current VI's Path() -> (path=w1570:path)
                    n988 = Open VI Reference(vi path=w1570) -> (vi reference=w1571:refnum<vi>, error out=w1572:errorcluster)  [unwired: 5 in]
                    n989 = property class="VI"(reference=w1571, error in=w1572) -> (reference out=w1569:refnum<vi>, error out=w1567:errorcluster, "Front Panel.PanelBounds"=w1565:T25)
                    n990 = Unbundle By Name(w1565) -> ("Left"=w1579:i16, "Top"=w1577:i16, "Right"=w1575:i16, "Bottom"=w1576:i16)
                    n991 = expression code="x/2"(w1580) -> (w1574:i32)
                    n992 = Add(x=w1575, y=w1574) -> (x+y=w1573:i32)
                    n993 = Subtract(x=w1579, y=w1574) -> (x-y=w1578:i32)
                    n994 = Bundle By Name(cluster=w1565, "Left"=w1578, "Top"=w1577, "Right"=w1573, "Bottom"=w1576) -> (w1564:T25)
                    n995 = property class="VI"(reference=w1569, error in=w1567, "Front Panel.PanelBounds"=w1564) -> (reference out=w1568:refnum<vi>, error out=w1566:errorcluster)
                    n996 = Close Reference(reference=w1568, error in (no error)=w1566) -> ()  [unwired: 1 out]
                  }
                }
                n997 = local write "창크게"(FALSE ("창크게")) -> ()
              }
            }
          }
          frame #13 {
            n998 = local read "Comm con status 1"() -> (w1582:bool)
            n999 = case shown="참" w1582 {
              frame False {
              }
              frame True {
                n1000 = local read "ms timer 5"() -> (w1589:u32)
                n1001 = Tick Count (ms)() -> (millisecond timer value=w1588:u32)
                n1002 = Subtract(x=w1588, y=w1589) -> (x-y=w1590:u32)
                n1003 = Greater Or Equal?(x=w1590, y=u32 100) -> (x >= y?=w1586:bool)
                n1004 = case shown="참" w1586 {
                  frame False {
                  }
                  frame True {
                    n1005 = local read "Port-act 1"() -> (w1595:refnum<visa-resource-name>)
                    n1006 = Tick Count (ms)() -> (millisecond timer value=w1591:u32)
                    n1007 = property on="BLE Interval buf" class="WFChart (엄격한)"() -> ("History Data"=w1597:u32[])  [unwired: 2 in, 2 out]
                    n1008 = local write "ms timer 5"(w1591) -> ()
                    n1009 = property class="Instr"(reference=w1595) -> ("Serial Settings:Number of Bytes at Serial Port"=w1594:u32)  [unwired: 1 in, 2 out]
                    n1010 = call-poly <vilib>:"Mean.vi"("X"=w1597) -> ("mean"=w1596:dbl)  [unwired: 1 out]
                    "BLE AVG-Interval Graph" <- w1596
                    n1011 = case shown="0, 기본" w1594 {
                      frame 0, Default {
                        w1599 = T3 3 items=["System", "Persistent Store", "Attribute database", "Connection", "Attribute client", "Security Manager", "Generic Access Profile", "Hardware"] ("Command Class (System)")
                        w1602 = T2 0 items=["Command / Response"=0, "Event"=128] ("Message Type (Command / Response)")
                        # "Get Rssi"
                        n1012 = local read "Port-act 1"() -> (w1603:refnum<visa-resource-name>)
                        n1013 = Build Array(u8 0 ("Message ID (0x00)")) -> (w1600:u8[])
                        n1014 = call "ble_write_message.vi"("Command Class (System)"=w1599, "Message Type (Command / Response)"=w1602, "Payload(Empty)"=w1600, "Message ID (0x00)"=u8 1, "COM Bluegiga in"=w1603) -> ()  [unwired: 4 in, 3 out]
                      }
                      frame 1 {
                      }
                    }
                    n1015 = local write "BLE Interval Time(ms)"(w1596) -> ()
                    n1016 = property on="BLE RSSI buf" class="WFChart (엄격한)"() -> ("History Data"=w1593:i16[])  [unwired: 2 in, 2 out]
                    n1017 = call-poly <vilib>:"Mean.vi"("X"=w1593) -> ("mean"=w1592:dbl)  [unwired: 1 out]
                    "BLE RSSI Graph" <- w1592
                    n1018 = local write "BLE RSSI (dBm)"(w1592) -> ()
                  }
                }
              }
            }
            n1019 = case shown="참" "Grahp Clear" {
              frame False {
              }
              frame True {
                # "BLE 버퍼 클리어"
                n1020 = local write "BLE Interval Time(ms)"(0.0 ("BLE Interval Time(ms)")) -> ()
                n1021 = property on="BLE Interval buf" class="WFChart (엄격한)"("History Data"=u32[] [] ("히스토리 데이터")) -> ()  [unwired: 2 in, 2 out]
                n1022 = property on="BLE Interval Graph" class="WFChart (엄격한)"("History Data"=dbl[] [] ("히스토리 데이터")) -> ()  [unwired: 2 in, 2 out]
                n1023 = local write "BLE RSSI (dBm)"(0.0 ("BLE RSSI (dBm)")) -> ()
                n1024 = property on="BLE RSSI buf" class="WFChart (엄격한)"("History Data"=i16[] [] ("히스토리 데이터")) -> ()  [unwired: 2 in, 2 out]
                n1025 = property on="BLE RSSI Graph" class="WFChart (엄격한)"("History Data"=i16[] [] ("히스토리 데이터")) -> ()  [unwired: 2 in, 2 out]
                n1026 = call "SUB-BLE Rx data Clear.vi"() -> ()  [unwired: 6 in]
              }
            }
            n1027 = case shown="참" "CDC Graph plot" {
              frame False {
              }
              frame True {
                n1028 = control-ref of="CDC(PCAP02) Graph"() -> (w1585:refnum<vi>)
                n1029 = local write "Clear graph 1"(TRUE ("그래프 지우기")) -> ()
                n1030 = call "SUB-Graph plot select.vi"("CDC(PCAP02) Graph 2"=w1585) -> ()  [unwired: 3 in]
              }
            }
          }
        }
        n1031 = Wait Until Next ms Multiple(millisecond multiple=u32 4 ("ms 배수")) -> ()  [unwired: 1 out]
        n1032 = local read "stop"() -> (w477:bool)
      }
      n1033 = while {
        stop <- w453 stop-if-true
        # "값이 변경된 경우 데이타 전송 플레그=온"
        # "Event"
        n1034 = event shown="[1] 키 다운" {
          selector: _ -> [_ _ _ _ _ _]
          dyn-events: _ -> [_ _ _ _ _ _]
          timeout: 50 -> [_ _ _ _ _ _]
          event Timeout {
            n1035 = event-data() -> ()  [unwired: 3 out]
          }
          event Key Down {
            # "Ctrl + 1"
            n1036 = event-data() -> ("Char"=w461:i16, "VKey"=w459:T21, "Mods"=w463:cluster{"Num Pad":bool, "Menu Key":bool})  [unwired: 6 out]
            n1037 = Unbundle By Name(w463) -> ("Menu Key"=w455:bool)
            n1038 = Equal?(x=eventvkey."ASCII" ("V 키"), y=w459) -> (x = y?=w457:bool)
            n1039 = Equal?(x=i16 49 ("문자"), y=w461) -> (x = y?=w458:bool)
            n1040 = And(x=w458, y=w457) -> (x .and. y?=w456:bool)
            n1041 = And(x=w456, y=w455) -> (x .and. y?=w454:bool)
            n1042 = case shown="참" w454 {
              frame False {
              }
              frame True {
                n1043 = local write "창크게"(TRUE ("창크게")) -> ()
              }
            }
          }
          event "Comm con 1": Value Change {
            n1044 = event-data() -> ("NewVal"=w465:bool)  [unwired: 6 out]
            n1045 = case shown="참" w465 {
              frame False {
                # "BLE Close"
                n1046 = local write "Port open 1"(FALSE) -> ()
                n1047 = local write "Port close 1"(TRUE) -> ()
              }
              frame True {
                # "BLE Open"
                n1048 = local write "Port open 1"(TRUE) -> ()
                n1049 = local write "Port close 1"(FALSE) -> ()
              }
            }
          }
          event "Setting load": Value Change {
            n1050 = event-data() -> ("NewVal"=w470:bool)  [unwired: 6 out]
            n1051 = case shown="참" w470 {
              frame False {
              }
              frame True {
                n1052 = local write "Setting load(led)"(TRUE ("Power On Flag")) -> ()
              }
            }
          }
          event "Data Logging": Value Change {
            n1053 = event-data() -> ()  [unwired: 7 out]
            n1054 = Tick Count (ms)() -> (millisecond timer value=w472:u32)
            n1055 = local write "Timer-ble log"(w472) -> ()
          }
          event Panel Close? {
            n1056 = event-data() -> ()  [unwired: 5 out]
            n1057 = local write "stop"(TRUE ("stop")) -> ()
            n1058 = event-data("Discard?"=TRUE ("stop")) -> ()  [unwired: 1 in, 1 out]
          }
        }
        n1059 = local read "stop"() -> (w453:bool)
      }
      n1060 = while {
        stop <- w337 stop-if-true
        # "BLE RxD handle"
        n1061 = local read "Comm con status 1"() -> (w336:bool)
        n1062 = local read "Port-act 1"() -> (w335:refnum<visa-resource-name>)
        n1063 = case shown="참" w336 {
          tunnel: w335 -> [_ w342]
          frame False {
          }
          frame True {
            n1064 = property class="Instr"(reference=w342) -> (reference out=w341:refnum<visa-resource-name>, error out=w340:errorcluster, "Serial Settings:Number of Bytes at Serial Port"=w339:u32)  [unwired: 1 in]
            n1065 = case shown="4.." w339 {
              tunnel: w341 -> [_ w363]
              tunnel: w340 -> [_ w362]
              frame 0, Default {
                # "BLE Tx sender"
                n1066 = local read "Comm con status 1"() -> (w345:bool)
                n1067 = And(x="Send", y=w345) -> (x .and. y?=w344:bool)
                n1068 = And(x=w345, y="Debugging Mode") -> (x .and. y?=w343:bool)
                n1069 = case shown="참" w344 {
                  frame False {
                  }
                  frame True {
                    (unwired) u16 12 ("Handle")
                    # "데이터 전송\n- 핸들/0x01"
                    n1070 = local read "Data(h)"() -> (w357:string)
                    n1071 = local read "Connection Status"() -> (w358:T4)
                    n1072 = local read "Port-act 1"() -> (w359:refnum<visa-resource-name>)
                    n1073 = String To Byte Array(string=w357) -> (unsigned byte array=w356:u8[])
                    n1074 = local read "Handle"() -> (w360:u8)
                    n1075 = call-poly "ble_write_by_handle.vi"("Connection Status"=w358, "Handle"=w360, "data (uint8array)"=w356, "COM Bluegiga in"=w359) -> ()  [unwired: 6 in, 2 out]
                  }
                }
                n1076 = case shown="참" w343 {
                  frame False {
                  }
                  frame True {
                    # "데이터 전송\n- 핸들 0x0B"
                    n1077 = local read "Mode"() -> (w351:bool)
                    n1078 = Select(t="JsP" ("문자열"), s=w351, f="imt" ("문자열")) -> (s? t:f=w350:string)
                    n1079 = local read "Connection Status"() -> (w354:T4)
                    n1080 = local read "Port-act 1"() -> (w355:refnum<visa-resource-name>)
                    n1081 = String To Byte Array(string=w350) -> (unsigned byte array=w353:u8[])
                    n1082 = call-poly "ble_write_by_handle.vi"("Connection Status"=w354, "Handle"=u16 11, "data (uint8array)"=w353, "COM Bluegiga in"=w355) -> ()  [unwired: 6 in, 2 out]
                  }
                }
              }
              frame 4.. {
                # "Rx Packet Data - Process"
                n1083 = call "ble_read_message.vi"("error in (no error)"=w362, "COM Bluegiga in"=w363) -> ("message package"=w361:u8[])  [unwired: 7 in, 2 out]
                n1084 = stacked-sequence {
                  seq-local: [_ w367 _ _ _ _] -> [_ _ w395 w405 w409 w419]
                  tunnel: w361 -> [_ w368 _ _ _ _]
                  frame #0 {
                    n1085 = local write "Packet Detect"(FALSE ("Packet Detect")) -> ()
                  }
                  frame #1 {
                    # "ble_evt_attclient_attribute_value"
                    n1086 = call "BLED1112-Rx Packet parser (EVENT-Attribute Client).vi"("message package"=w368) -> ("message out"=w367:u8[], "Packet OK"=w366:bool, "Data Structure"=w365:T1)  [unwired: 2 in]
                    n1087 = case shown="참" w366 {
                      tunnel: w365 -> [_ w373]
                      frame False {
                      }
                      frame True {
                        n1088 = local read "Data Logging"() -> (w372:bool)
                        n1089 = Unbundle By Name(w373) -> ("Attribute value (data)"=w374:u8[])
                        n1090 = local write "Packet Detect"(TRUE ("Packet Detect")) -> ()
                        n1091 = Byte Array To String(unsigned byte array=w374) -> (string=w377:string)
                        n1092 = local write "Rx buf 1"(w377) -> ()
                        n1093 = call "SUB-BLE Rx data save.vi"("Rx Packet Structure"=w373, "BLE RxD"=w374) -> ("Full packet"=w369:u8[], "Mon Packet?"=w370:bool)  [unwired: 1 in, 1 out]
                        n1094 = And(x=w370, y=w372) -> (x .and. y?=w371:bool)
                        n1095 = case shown="참" w370 {
                          frame False {
                          }
                          frame True {
                            n1096 = local read "ms timer 4"() -> (w381:u32)
                            n1097 = Tick Count (ms)() -> (millisecond timer value=w379:u32)
                            n1098 = Subtract(x=w379, y=w381) -> (x-y=→"BLE Interval buf":u32)
                            n1099 = local write "ms timer 4"(w379) -> ()
                          }
                        }
                        n1100 = local read "Rx Cnt"() -> (w375:i32)
                        n1101 = case shown="참" w371 {
                          tunnel: w369 -> [_ w386]
                          tunnel: w375 -> [_ w383]
                          frame False {
                          }
                          frame True {
                            # "Save log data"
                            n1102 = local read "log ble buf"() -> (w391:string)
                            n1103 = Format Into String(format string="%06d  " ("포맷 문자열"), w383) -> (resulting string=w384:string)  [unwired: 2 in, 1 out]
                            n1104 = call <vilib>:"Space Constant.vi"() -> ("String"=w382:string)
                            n1105 = Array To Spreadsheet String(delimiter (Tab)=w382, array=w386, 3:"%02X" ("포맷 문자열")) -> (spreadsheet string=w387:string)
                            n1106 = Format Date/Time String(time format string (%c)="%H:%M:%S%3u>  " ("상태")) -> (date/time string=w389:string)  [unwired: 2 in]
                            n1107 = Concatenate Strings(w391, w384, w389, w387) -> (w390:string)
                            n1108 = local write "log ble buf"(w390) -> ()
                            n1109 = local write "log data1"(TRUE ("log data1")) -> ()
                          }
                        }
                        n1110 = Increment(x=w375) -> (x+1=w378:i32)
                        n1111 = local write "Rx Cnt"(w378) -> ()
                        "Rx Packet Structure" <- w373
                      }
                    }
                  }
                  frame #2 {
                    # "Rx Packet parser (EVENT-Connection status)"
                    n1112 = local read "Packet Detect"() -> (w394:bool)
                    n1113 = case shown="거짓" w394 {
                      tunnel: w395 -> [w398 _]
                      frame False {
                        n1114 = call "BLED1112-Rx Packet parser (EVENT-Connection status).vi"("message package"=w398) -> ("Packet OK"=w397:bool, "Data Structure"=w396:T26)  [unwired: 2 in, 1 out]
                        n1115 = case shown="참" w397 {
                          tunnel: w396 -> [_ w403]
                          frame False {
                          }
                          frame True {
                            n1116 = Unbundle By Name(w403) -> ("bonding(0xFF)"=w402:u8)
                            n1117 = local write "Packet Detect"(TRUE ("Packet Detect")) -> ()
                            n1118 = Not Equal?(x=w402, y=255 ("Rx Cnt")) -> (x != y?=w400:bool)
                            n1119 = local write "Disconnected"(w400) -> ()
                          }
                        }
                      }
                      frame True {
                      }
                    }
                  }
                  frame #3 {
                    # "Rx Packet parser (RESPONSE GAP)"
                    n1120 = local read "Packet Detect"() -> (w404:bool)
                    n1121 = case shown="거짓" w404 {
                      tunnel: w405 -> [w407 _]
                      frame False {
                        n1122 = call "BLED1112-Rx Packet parser (RESPONSE-GAP).vi"("message package"=w407) -> ("Packet OK"=w406:bool)  [unwired: 2 in, 2 out]
                        n1123 = case shown="참" w406 {
                          frame False {
                          }
                          frame True {
                            n1124 = local write "Packet Detect"(TRUE ("Packet Detect")) -> ()
                          }
                        }
                      }
                      frame True {
                      }
                    }
                  }
                  frame #4 {
                    # "Rx Packet parser (EVENT-Disconnected)"
                    n1125 = local read "Packet Detect"() -> (w410:bool)
                    n1126 = case shown="거짓" w410 {
                      tunnel: w409 -> [w412 _]
                      frame False {
                        n1127 = call "BLED1112-Rx Packet parser (EVENT-Disconnected).vi"("message package"=w412) -> ("Packet OK"=w411:bool)  [unwired: 2 in, 2 out]
                        n1128 = case shown="참" w411 {
                          frame False {
                          }
                          frame True {
                            n1129 = local write "Packet Detect"(TRUE ("Packet Detect")) -> ()
                            n1130 = local write "Disconnected"(TRUE ("Packet Detect")) -> ()
                            n1131 = local write "Comm con status 1"(FALSE ("Packet Detect")) -> ()
                            n1132 = local write "Comm con 1"(FALSE ("Packet Detect")) -> ()
                            n1133 = local write "ACT-Comm"(FALSE ("Packet Detect")) -> ()
                            n1134 = One Button Dialog(message="BLE Disconnected!" ("메시지")) -> ()  [unwired: 1 in, 1 out]
                          }
                        }
                      }
                      frame True {
                      }
                    }
                  }
                  frame #5 {
                    # "Rx Packet parser (Get Rssi))"
                    n1135 = local read "Packet Detect"() -> (w420:bool)
                    n1136 = case shown="거짓" w420 {
                      tunnel: w419 -> [w423 _]
                      frame False {
                        n1137 = call "BLED1112-Rx Packet parser (Get Rssi).vi"("message package"=w423) -> ("Packet OK"=w422:bool, "Data Structure"=w421:T27)  [unwired: 2 in, 1 out]
                        n1138 = case shown="참" w422 {
                          tunnel: w421 -> [_ w425]
                          frame False {
                          }
                          frame True {
                            n1139 = local write "Packet Detect"(TRUE ("Packet Detect")) -> ()
                            n1140 = Unbundle By Name(w425) -> ("rssi"=→"BLE RSSI buf":i16)
                          }
                        }
                      }
                      frame True {
                      }
                    }
                  }
                }
              }
            }
          }
        }
        n1141 = Wait Until Next ms Multiple(millisecond multiple=u32 1 ("ms 배수")) -> ()  [unwired: 1 out]
        n1142 = local read "stop"() -> (w337:bool)
      }
      n1143 = while {
        stop <- w436 stop-if-true
        # "Load test-one time"
        n1144 = stacked-sequence {
          frame #0 {
            n1145 = local read "Force Set"() -> (w438:bool)
            n1146 = case shown="참" w438 {
              frame False {
              }
              frame True {
                n1147 = stacked-sequence {
                  frame #0 {
                    n1148 = local read "Port-FTS"() -> (w442:refnum<visa-resource-name>)
                    n1149 = local read "Load(lb)"() -> (w441:dbl)
                    n1150 = call "_시리얼_Mark10-제어 (압력설정).vi"("FTS 제어 상태"=T20 "압력제어 시작", "압력 설정(lb)"=w441, "시리얼 포트"=w442) -> ("통신 정상"=w439:bool)  [unwired: 2 out]
                    n1151 = case shown="거짓" w439 {
                      frame False {
                        n1152 = One Button Dialog(message="Can't find equipment!" ("메시지")) -> ()  [unwired: 1 in, 1 out]
                      }
                      frame True {
                      }
                    }
                  }
                  frame #1 {
                    n1153 = local write "Force Set"(FALSE ("Force Set")) -> ()
                  }
                }
              }
            }
          }
          frame #1 {
            n1154 = local read "Head Up"() -> (w445:bool)
            n1155 = case shown="참" w445 {
              frame False {
              }
              frame True {
                n1156 = stacked-sequence {
                  frame #0 {
                    n1157 = local read "Port-FTS"() -> (w449:refnum<visa-resource-name>)
                    n1158 = local read "Load(lb)"() -> (w448:dbl)
                    n1159 = call "_시리얼_Mark10-제어 (압력설정).vi"("FTS 제어 상태"=T20 "헤더 상단 이동", "압력 설정(lb)"=w448, "시리얼 포트"=w449) -> ("통신 정상"=w446:bool)  [unwired: 2 out]
                    n1160 = case shown="거짓" w446 {
                      frame False {
                        n1161 = One Button Dialog(message="Can't find equipment!" ("메시지")) -> ()  [unwired: 1 in, 1 out]
                      }
                      frame True {
                      }
                    }
                  }
                  frame #1 {
                    n1162 = local write "Head Up"(FALSE ("Force Set")) -> ()
                  }
                }
              }
            }
          }
        }
        n1163 = Wait Until Next ms Multiple(millisecond multiple=u32 300 ("ms 배수")) -> ()  [unwired: 1 out]
        n1164 = local read "stop"() -> (w436:bool)
      }
      n1165 = while {
        stop <- w431 stop-if-true
        # "test-LED blink"
        n1166 = local read "Test Start"() -> (w430:bool)
        n1167 = local read "Force Set"() -> (w429:bool)
        n1168 = local read "Head Up"() -> (w427:bool)
        n1169 = Compound Arithmetic op=OR ("복합 연산")(w430, w429, w427) -> (w428:bool)
        n1170 = case shown="거짓" w428 {
          frame False {
            n1171 = local write "FTS Testing"(FALSE ("FTS 시험 진행")) -> ()
          }
          frame True {
            n1172 = local read "FTS Testing"() -> (w435:bool)
            n1173 = Not(x=w435) -> (.not. x?=w434:bool)
            n1174 = local write "FTS Testing"(w434) -> ()
          }
        }
        n1175 = Wait Until Next ms Multiple(millisecond multiple=u32 300 ("ms 배수")) -> ()  [unwired: 1 out]
        n1176 = local read "stop"() -> (w431:bool)
      }
    }
    frame #6 {
      # "시리얼 포트 닫기"
      n1177 = local read "Comm con 1"() -> (w1610:bool)
      n1178 = case shown="참" w1610 {
        frame False {
        }
        frame True {
          # "BLE 통신 종료"
          n1179 = local read "Port-act 1"() -> (w1611:refnum<visa-resource-name>)
          n1180 = local read "Connection Status"() -> (w1616:T4)
          n1181 = call "_시리얼_buf clear.vi"("시리얼 포트"=w1611) -> ("에러 출력"=w1614:errorcluster, "시리얼 포트 2"=w1615:refnum<visa-resource-name>)  [unwired: 3 in]
          n1182 = call "ble_disconnect_device.vi"("Connection Status"=w1616, "error in (no error)"=w1614, "COM Bluegiga in"=w1615) -> ("error out"=w1613:errorcluster, "COM Bluegiga out"=w1612:refnum<visa-resource-name>)  [unwired: 7 in]
          n1183 = VISA Close(VISA resource name=w1612, error in (no error)=w1613) -> ()  [unwired: 1 out]
        }
      }
    }
    frame #7 {
      # "프로그램 설정값-파일로 저장한다."
      n1184 = call <vilib>:"Open Config Data.vi"("configuration file path"=w1621) -> ("error out"=w1624:errorcluster, "refnum"=w1623:T23)  [unwired: 2 in, 7 out]
      n1185 = stacked-sequence {
        tunnel: w1623 -> [w1628 w1631 w1636 w1641 w1646]
        tunnel: w1624 -> [w1627 w1630 w1635 w1640 w1645]
        tunnel: "GUI Setting" ("section") -> [w1629 w1632 w1637 w1642 _]
        tunnel: [_ _ _ _ w1646] -> w1620
        tunnel: [_ _ _ _ w1645] -> w1619
        frame #0 {
          w1626 = "Com Port-Board1"  # Key 1
          n1186 = local read "Port-set 1"() -> (w1625:refnum<visa-resource-name>)
          n1187 = call-poly <vilib>:"Write Key.vi"("section"=w1629, "error in (no error)"=w1627, "value"=w1625, "key"=w1626, "refnum"=w1628) -> ()  [unwired: 1 in, 6 out]
        }
        frame #1 {
          w1634 = "Com Port-FTS"  # Key 1
          n1188 = local read "Port-FTS"() -> (w1633:refnum<visa-resource-name>)
          n1189 = call-poly <vilib>:"Write Key.vi"("section"=w1632, "error in (no error)"=w1630, "value"=w1633, "key"=w1634, "refnum"=w1631) -> ()  [unwired: 1 in, 6 out]
        }
        frame #2 {
          w1639 = "Logno"  # Key 1
          n1190 = local read "Log no"() -> (w1638:string)
          n1191 = call-poly <vilib>:"Write Key.vi"("section"=w1637, "error in (no error)"=w1635, "value"=w1638, "key"=w1639, "refnum"=w1636) -> ()  [unwired: 1 in, 6 out]
        }
        frame #3 {
          w1644 = "Interval(ms)"  # Key 1
          n1192 = local read "Update(ms)"() -> (w1643:u16)
          n1193 = call-poly <vilib>:"Write Key.vi"("section"=w1642, "error in (no error)"=w1640, "value"=w1643, "key"=w1644, "refnum"=w1641) -> ()  [unwired: 7 out]
        }
        frame #4 {
        }
      }
      n1194 = call <vilib>:"Close Config Data.vi"("error in (no error)"=w1619, "refnum"=w1620) -> ()  [unwired: 1 in, 9 out]
      n1195 = call "Read and Write Controls to Automatic Config File.vi"("Action"=RWC_Actions."Write", "Control References"=w1617) -> ()  [unwired: 9 in, 1 out]
    }
    frame #8 {
      # "종료"
      n1196 = call "SUB-Exit.vi"() -> ()  [unwired: 4 in]
    }
  }
  n1197 = local write "Offset Souce"(enum32{"Normal", "Raw"}."Normal" ("Offset Souce")) -> ()
  n1198 = local write "Mode"(TRUE ("Mode")) -> ()
  n1199 = local write "Rx-debug"(FALSE ("Rx-debug")) -> ()
  n1200 = local write "Packet No."(0 ("Packet No.")) -> ()
